vi "Omniax_MotorDrive_XYZR_20100916stable2.vi"() -> ()   [LabVIEW 2009]
uses:
  <vilib>/Utility/file.llb/Read From Spreadsheet File (DBL).vi
  <vilib>/Utility/file.llb/Read From Spreadsheet File (string).vi
  <vilib>/Instr/_visa.llb/VISA Configure Serial Port (Instr).vi
  <vilib>/Utility/file.llb/Write To Spreadsheet File (string).vi
  <vilib>/Utility/file.llb/Write To Spreadsheet File (DBL).vi
panel:
  out "Scanning":bool
  out "Laser Shutter":bool
  in  "SHUTTER SYNC":bool
  in  "Laser Shutter":bool
  out "#th loop":dbl
  in  "# of loops":dbl
  in  "LOOP":bool
  out "OP":bool
  out "CL":bool
  out "Valve \nopend/closed":bool
  in  "OK Button":bool
  out "STATUS":string
  in  "Delete Button":bool
  in  "String":string
  in  "Add Button":bool
  in  "Set Button":bool
  in  "Preset positions":i32(ring) items=["ZERO", "Default", "CDOSE", "QMS", "test", "test2", "test3", "yag position", "Sample Long Edge  ", "SPUTTER POS"]
  out "Presets":i32[][](array[numeric])
  out "X MINPOS":i32=-94296
  out "X MAXPOS":i32=-34296
  out "Y MINPOS":i32=-94296
  out "Y MAXPOS":i32=-34296
  out "R MAXPOS":i32=-34296
  out "R MINPOS":i32=-94296
  out "Z MINPOS":i32=-94296
  out "Z MAXPOS":i32=-34296
  in  "HARDSTOP":bool
  in  "GO":bool
  out "XYZR VEL PV Array":i32[](array[numeric])
  out "XYZ in RANGE Array":bool[](array[boolean])
  out "STEP SP Array":i32[](array[numeric])
  out "RUNHOLDArray":i32[](array[numeric])
  out "ZCONSTArray":dbl[](array[numeric])
  out "RCONSTArray":dbl[](array[numeric])
  out "XCONSTArray":dbl[](array[numeric])
  out "YCONSTArray":dbl[](array[numeric])
  out "Error Array":errorcluster[](array[cluster])
  out "COM PORT Array":refnum<visa-resource-name>[](array[refnum])
  out "Z COM PORT":refnum<visa-resource-name>="COM6"
  in  "Tab Control 3":enum32{"Status", "Reset"}(tab)
  out "Y in Range":bool
  out "Y Scan":bool
  out "Y in Motion":bool
  out "Y Backlash corr":bool
  out "X  in Range":bool
  out "X Scan":bool
  out "X  in Motion":bool
  out "X Backlash corr":bool
  out "Z in Range":bool
  out "Z Scan":bool
  out "Z in Motion":bool
  out "Z Backlash corr":bool
  out "R in Range":bool
  out "R Scan":bool
  out "R in Motion":bool
  out "R Backlash corr":bool
  out "X Ready":bool
  out "Y Ready":bool
  out "Z Ready":bool
  out "R Ready":bool
  in  "Reset Y Position mm":dbl
  out "Reset Y Motor Steps":i32
  in  "Reset X Position mm":dbl
  out "Reset X Motor Steps":i32
  in  "Reset Z Position mm":dbl
  out "Reset Z Motor Steps":i32
  in  "Reset R Position deg":dbl
  out "Reset R Motor Steps":i32
  in  "Reset":bool
  in  "Tab Control 2":enum32{"mm", "step"}(tab)
  in  "X Scan Length SP mm":dbl
  in  "X Scan Velocity SP mm/sec":dbl
  in  "Y Scan Length SP mm":dbl
  in  "Y Scan Velocity SP mm/sec":dbl
  in  "Set Scan \nParameters":bool
  in  "Z Scan Length SP mm":dbl
  in  "Z Scan Velocity SP mm/sec":dbl
  in  "R Scan Length SP deg":dbl
  in  "R Scan Velocity SP deg/sec":dbl
  in  "Z as dominating length":bool
  in  "X Scan Velocity SP steps/sec":i32=1 min=1 max=102400 step=1
  in  "X Scan Length SP steps":i32 min=-2304000 max=2304000 step=100
  out "X Scan length MV mm":dbl
  out "X Scan velocity MV mm/sec":dbl format="%#_6f"
  in  "Y Scan Velocity SP steps/sec":i32=1 min=1 max=102400 step=1
  in  "Y Scan Length SP steps":i32 min=-2304000 max=2304000 step=100
  out "Y Scan length MV mm":dbl
  out "Y Scan velocity MV mm/sec":dbl format="%#_6f"
  in  "Z Scan Velocity SP steps/sec":i32=1 min=1 max=204800 step=1
  in  "Z Scan Length SP steps":i32 min=-10240000 max=92160000 step=100
  out "Z Scan length MV mm":dbl
  out "Z Scan velocity MV mm/sec":dbl format="%#_6f"
  in  "R Scan Velocity SP steps/sec":i32=1 min=1 max=102400 step=1
  in  "R Scan Length SP steps":i32 min=-1501867 max=4642133 step=100
  out "R Scan length MV deg":dbl
  out "R Scan velocity MV deg/sec":dbl format="%#_6f"
  out "atan Y/Z":dbl
  in  "Tab Control":enum32{"mm", "step"}(tab)
  in  "X Position SP mm":dbl
  in  "X Velocity SP mm/sec":dbl
  in  "X Move Set":bool
  in  "Y Move Set":bool
  in  "Y Position SP mm":dbl
  in  "Y Velocity SP mm/sec":dbl
  in  "Z Position SP mm":dbl
  in  "Z Velocity SP mm/sec":dbl
  in  "Z Move Set":bool
  in  "R Position SP deg":dbl
  in  "R Velocity SP deg/sec":dbl
  in  "R Move Set":bool
  in  "X Velocity SP step/sec":i32 min=1 max=128000
  out "X Velocity MV mm/sec":dbl
  in  "Y Velocity SP step/sec":i32 min=1 max=128000
  out "Y Velocity MV mm/sec":dbl
  in  "Z Velocity SP step/sec":i32 min=1 max=204800
  out "Z Velocity MV mm/sec":dbl
  in  "R Velocity SP step/sec":i32 min=1 max=20000
  out "R Velocity MVdeg/sec":dbl
  in  "Y Step SP":i32=-20000 min=-2304000 max=2304000 step=500
  out "Y Position MV mm":dbl
  in  "X Step SP":i32=-20000 min=-2304000 max=2304000 step=500
  out "X Position MV mm":dbl
  in  "Z Step SP":i32=-20000 min=0 max=102400000 step=500
  out "Z Position MV mm":dbl
  in  "R Step SP":i32=-20000 min=-6144000 max=0 step=500
  out "R Position MV deg":dbl
  out "X Step PV":i32 max=2000
  out "Y Step PV":i32 max=2000
  out "Z Step PV":i32 max=2000
  out "R Step PV":i32 max=2000
  in  "Clear ZY":bool
  out "ZY Graph":cluster{dbl[], dbl[]}(graph)
  out "ZR Graph":cluster{"Y":dbl[], "Y":dbl[]}[](graph)
  out "XY Graph":cluster{"Y":dbl[], "Y":dbl[]}[](graph)
  out "X Scan Duration":dbl
  out "Y Scan Duration":dbl
  out "Z Scan Duration":dbl
  out "R Scan Duration":dbl
  out "R Backlash steps/sec":i32
  out "R Backlash":i32
  out "R Holding Current %":i32
  out "R Run Current %":i32
  out "R offset deg":dbl
  out "R deg/rev":dbl
  out "R steps/rev":u32
  out "R velocity PV step/sec":i32
  out "R COM PORT":refnum<visa-resource-name>="COM5"
  out "R Position deg PV":dbl
  out "Z Backlash steps/sec":i32
  out "Z Backlash":i32
  out "Z Holding Current %":i32
  out "Z Run Current %":i32
  out "Z offset mm":dbl
  out "Z mm/rev":dbl
  out "Z steps/rev":u32
  out "Z  velocity PV step/sec":i32
  out "Z Position mm PV":dbl
  out "X Position mm PV":dbl
  out "X velocity PV step/sec":i32
  in  "Send scan parameter":bool
  out "X Backlash steps/sec":i32
  out "X Backlash":i32
  out "X Holding Current %":i32
  out "X Run Current %":i32
  out "X offset mm":dbl
  out "X mm/rev":dbl
  out "X steps/rev":u32
  out "X COM PORT":refnum<visa-resource-name>="COM5"
  out "Y Backlash steps/sec":i32
  out "Y Backlash":i32
  out "Y Holding Current %":i32
  out "Y Run Current %":i32
  in  "Scan Cancel":bool
  out "Y Position mm PV":dbl
  out "Y offset mm":dbl
  out "Y mm/rev":dbl
  out "Y steps/rev":u32
  out "Y velocity PV step/sec":i32
  in  "Scan Go":bool
  in  "Stop":bool
  out "Y COM PORT":refnum<visa-resource-name>="COM5"
  # "MX"
  # "MY"
  # "MZ"
  # "MR"
  # "Indicators"
  # "L"
  # "M"
  # "B"
  # "S"
  # "R"
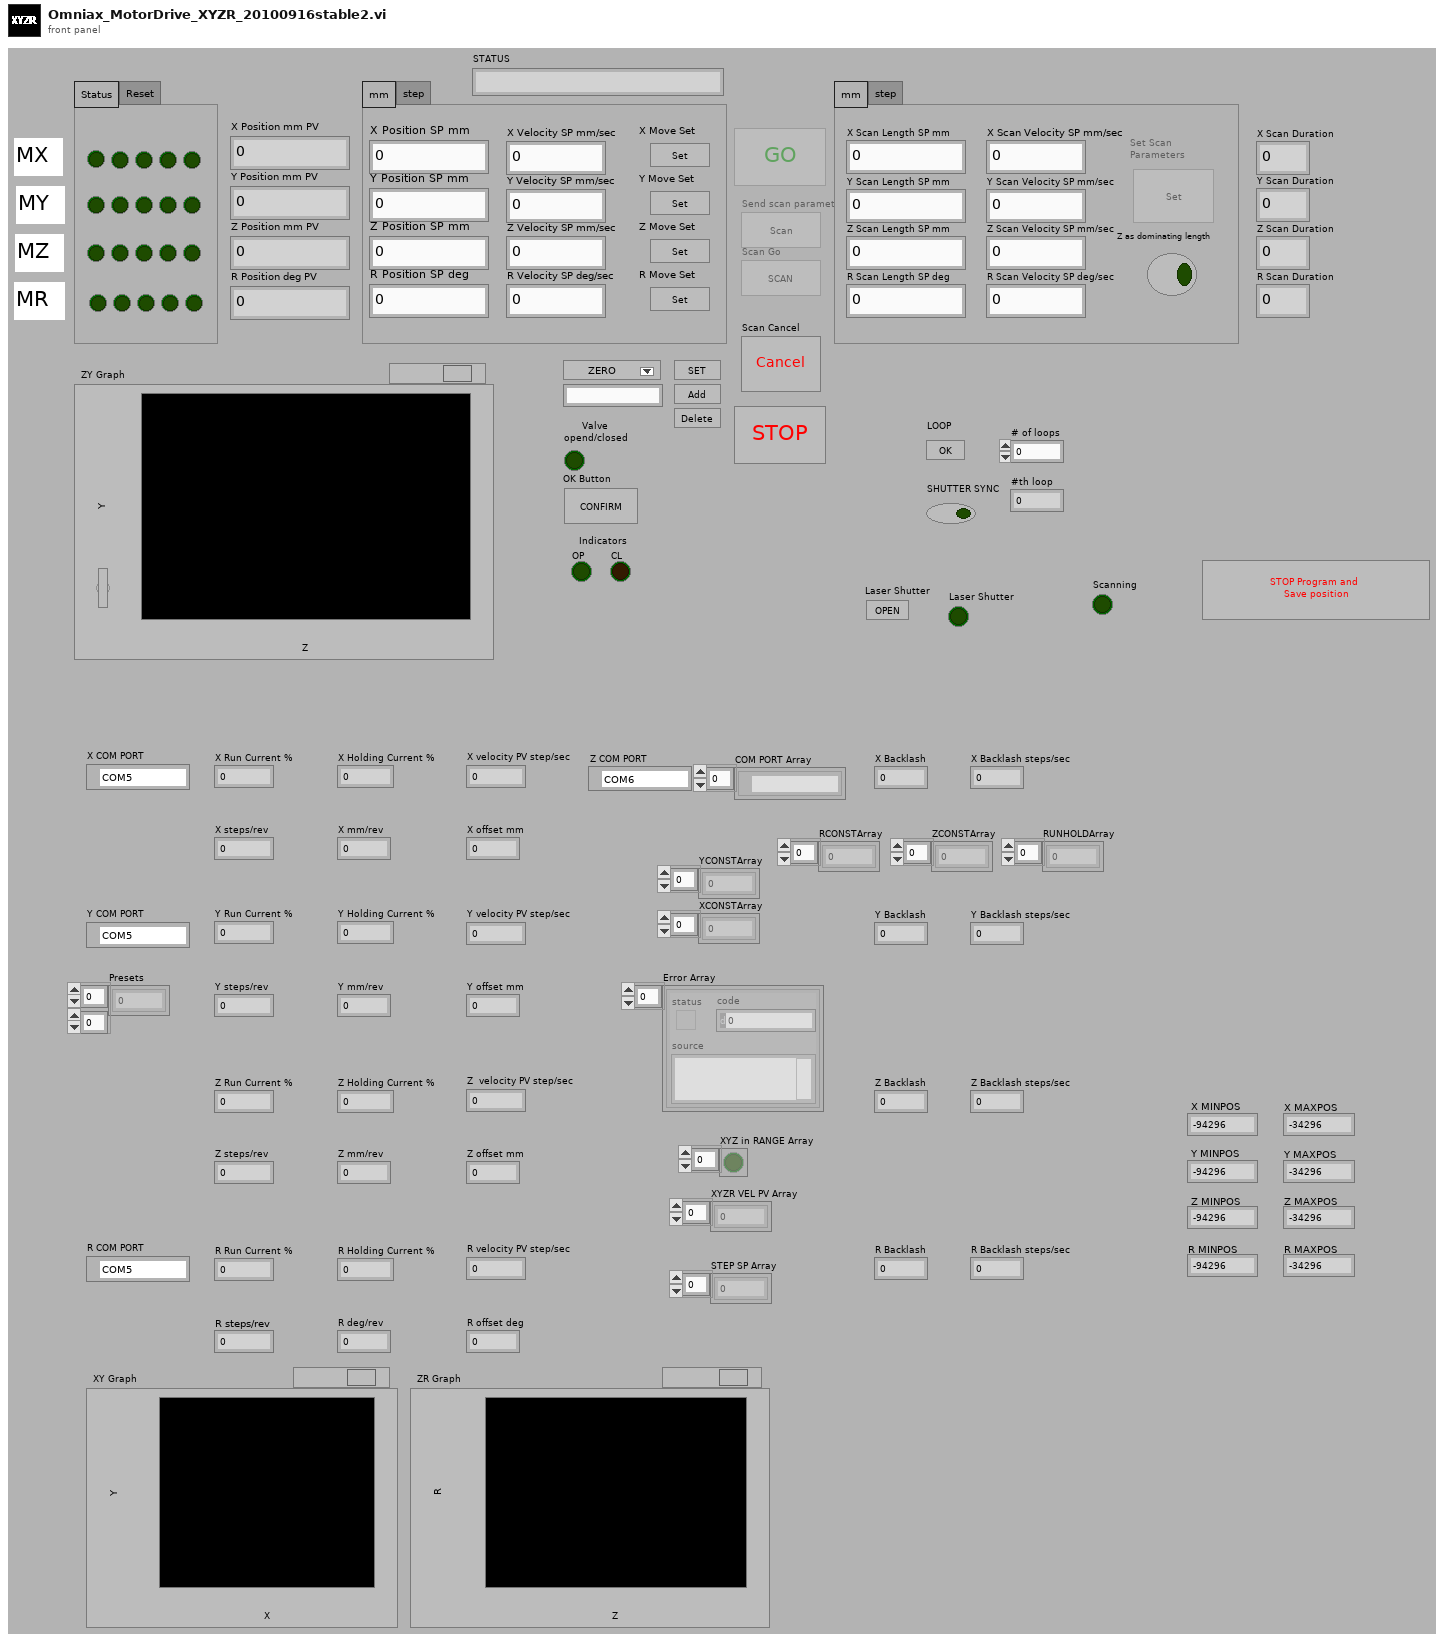
[diagram p1: front panel]
types:
  T1 = cluster{"Error Array OUT[0]":errorcluster, "Error Array OUT[1]":errorcluster, "Error Array OUT[2]":errorcluster, "Error Array OUT[3]":errorcluster, "Error Array OUT[4]":errorcluster, "Error Array OUT[5]":errorcluster, "Error Array OUT[6]":errorcluster, "Error Array OUT[7]":errorcluster, "Error Array OUT[8]":errorcluster}
  T2 = cluster{"COM PORT Array OUT[0]":refnum<visa-resource-name>, "COM PORT Array OUT[1]":refnum<visa-resource-name>, "COM PORT Array OUT[2]":refnum<visa-resource-name>, "COM PORT Array OUT[3]":refnum<visa-resource-name>, "COM PORT Array OUT[4]":refnum<visa-resource-name>, "COM PORT Array OUT[5]":refnum<visa-resource-name>, "COM PORT Array OUT[6]":refnum<visa-resource-name>, "COM PORT Array OUT[7]":refnum<visa-resource-name>, "COM PORT Array OUT[8]":refnum<visa-resource-name>}
  T3 = cluster{"STEP SP Array OUT[0]":i32, "STEP SP Array OUT[1]":i32, "STEP SP Array OUT[2]":i32, "STEP SP Array OUT[3]":i32, "STEP SP Array OUT[4]":i32, "STEP SP Array OUT[5]":i32, "STEP SP Array OUT[6]":i32, "STEP SP Array OUT[7]":i32, "STEP SP Array OUT[8]":i32}
  T4 = cluster{"XYZR MAX MIN POS[0]":i32, "XYZR MAX MIN POS[1]":i32, "XYZR MAX MIN POS[2]":i32, "XYZR MAX MIN POS[3]":i32, "XYZR MAX MIN POS[4]":i32, "XYZR MAX MIN POS[5]":i32, "XYZR MAX MIN POS[6]":i32, "XYZR MAX MIN POS[7]":i32, "XYZR MAX MIN POS[8]":i32}
  T5 = cluster{"XYZ in RANGE Array OUT[0]":bool, "XYZ in RANGE Array OUT[1]":bool, "XYZ in RANGE Array OUT[2]":bool, "XYZ in RANGE Array OUT[3]":bool, "XYZ in RANGE Array OUT[4]":bool, "XYZ in RANGE Array OUT[5]":bool, "XYZ in RANGE Array OUT[6]":bool, "XYZ in RANGE Array OUT[7]":bool, "XYZ in RANGE Array OUT[8]":bool}
  T6 = cluster{"XY Max Min array OUT[0]":dbl, "XY Max Min array OUT[1]":dbl, "XY Max Min array OUT[2]":dbl, "XY Max Min array OUT[3]":dbl, "XY Max Min array OUT[4]":dbl, "XY Max Min array OUT[5]":dbl, "XY Max Min array OUT[6]":dbl, "XY Max Min array OUT[7]":dbl, "XY Max Min array OUT[8]":dbl}
  T7 = cluster{"XYZR VEL PV Array OUT[0]":i32, "XYZR VEL PV Array OUT[1]":i32, "XYZR VEL PV Array OUT[2]":i32, "XYZR VEL PV Array OUT[3]":i32, "XYZR VEL PV Array OUT[4]":i32, "XYZR VEL PV Array OUT[5]":i32, "XYZR VEL PV Array OUT[6]":i32, "XYZR VEL PV Array OUT[7]":i32, "XYZR VEL PV Array OUT[8]":i32}
  T8 = cluster{"[0]":i32, "[1]":i32, "[2]":i32, "[3]":i32, "[4]":i32, "[5]":i32, "[6]":i32, "[7]":i32, "[8]":i32}
  T9 = enum8{"Enabled", "Disabled", "Disabled and Grayed Out"}
  T10 = enum16{"Stop", "Reset", "Run Current", "Holding Current", "Accel Rate", "Decel Rate", "Move to Relative Position", "Move to Absolute Position", "Echo Mode", "Print Parameter", "Send String", "Microstep Resolution", "Set Current Position", "Max Velocity"}
  T11 = cluster{"Presets[0]":i32, "Presets[1]":i32, "Presets[2]":i32, "Presets[3]":i32, "Presets[4]":i32, "Presets[5]":i32, "Presets[6]":i32, "Presets[7]":i32, "Presets[8]":i32}
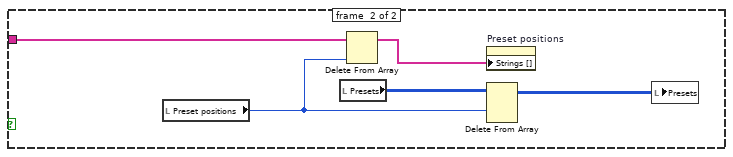
[diagram p4: hidden frame]
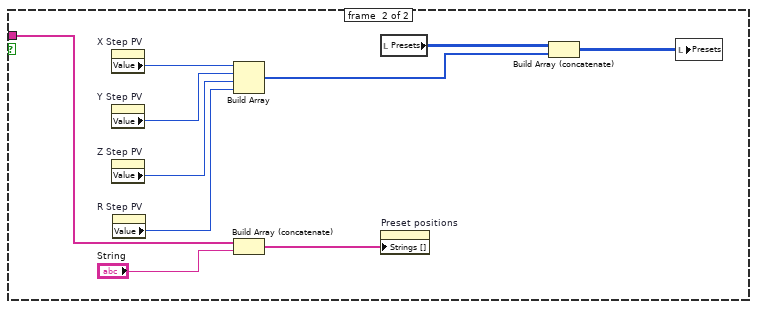
[diagram p5: hidden frame]
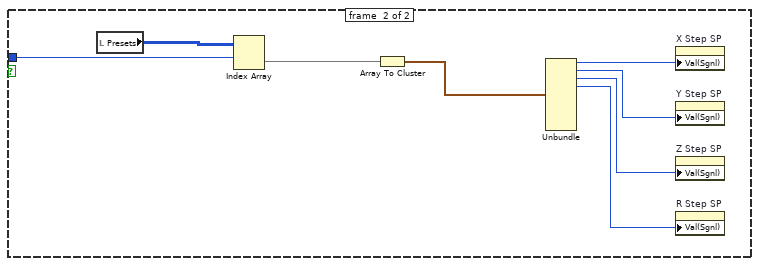
[diagram p6: hidden frame]
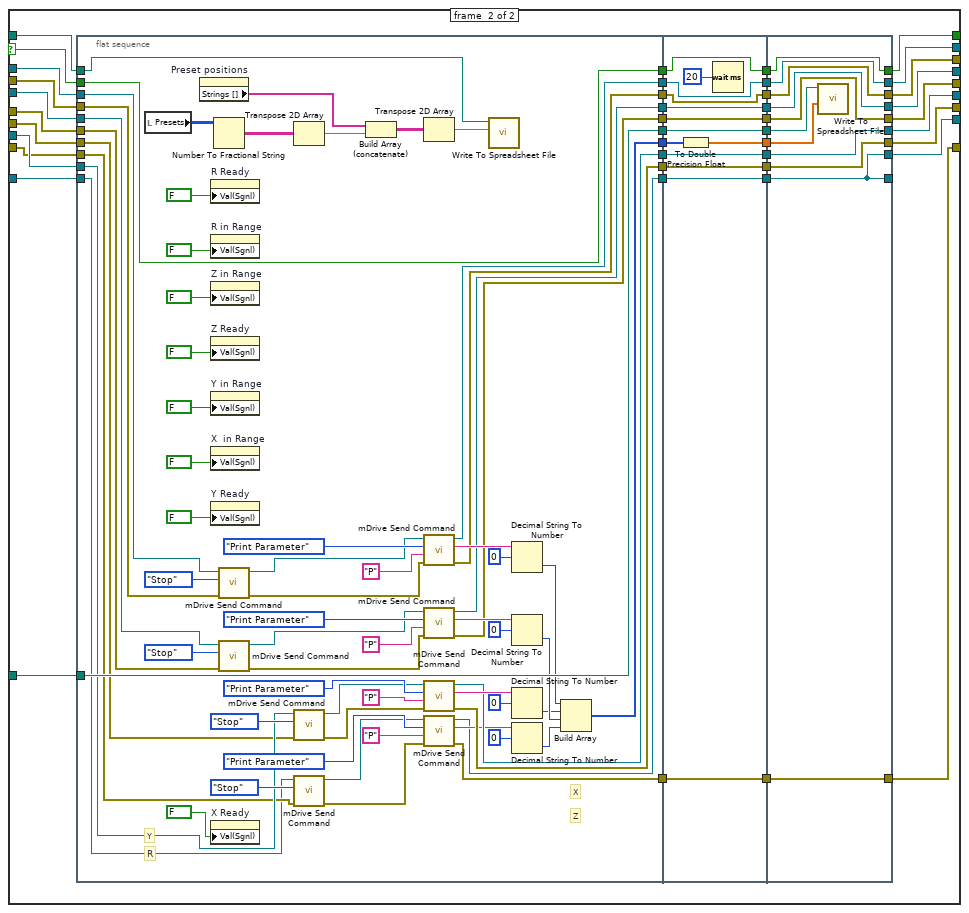
[diagram p7: hidden frame]
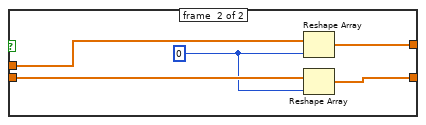
[diagram p8: hidden frame]
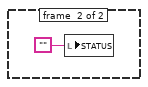
[diagram p10: hidden frame]
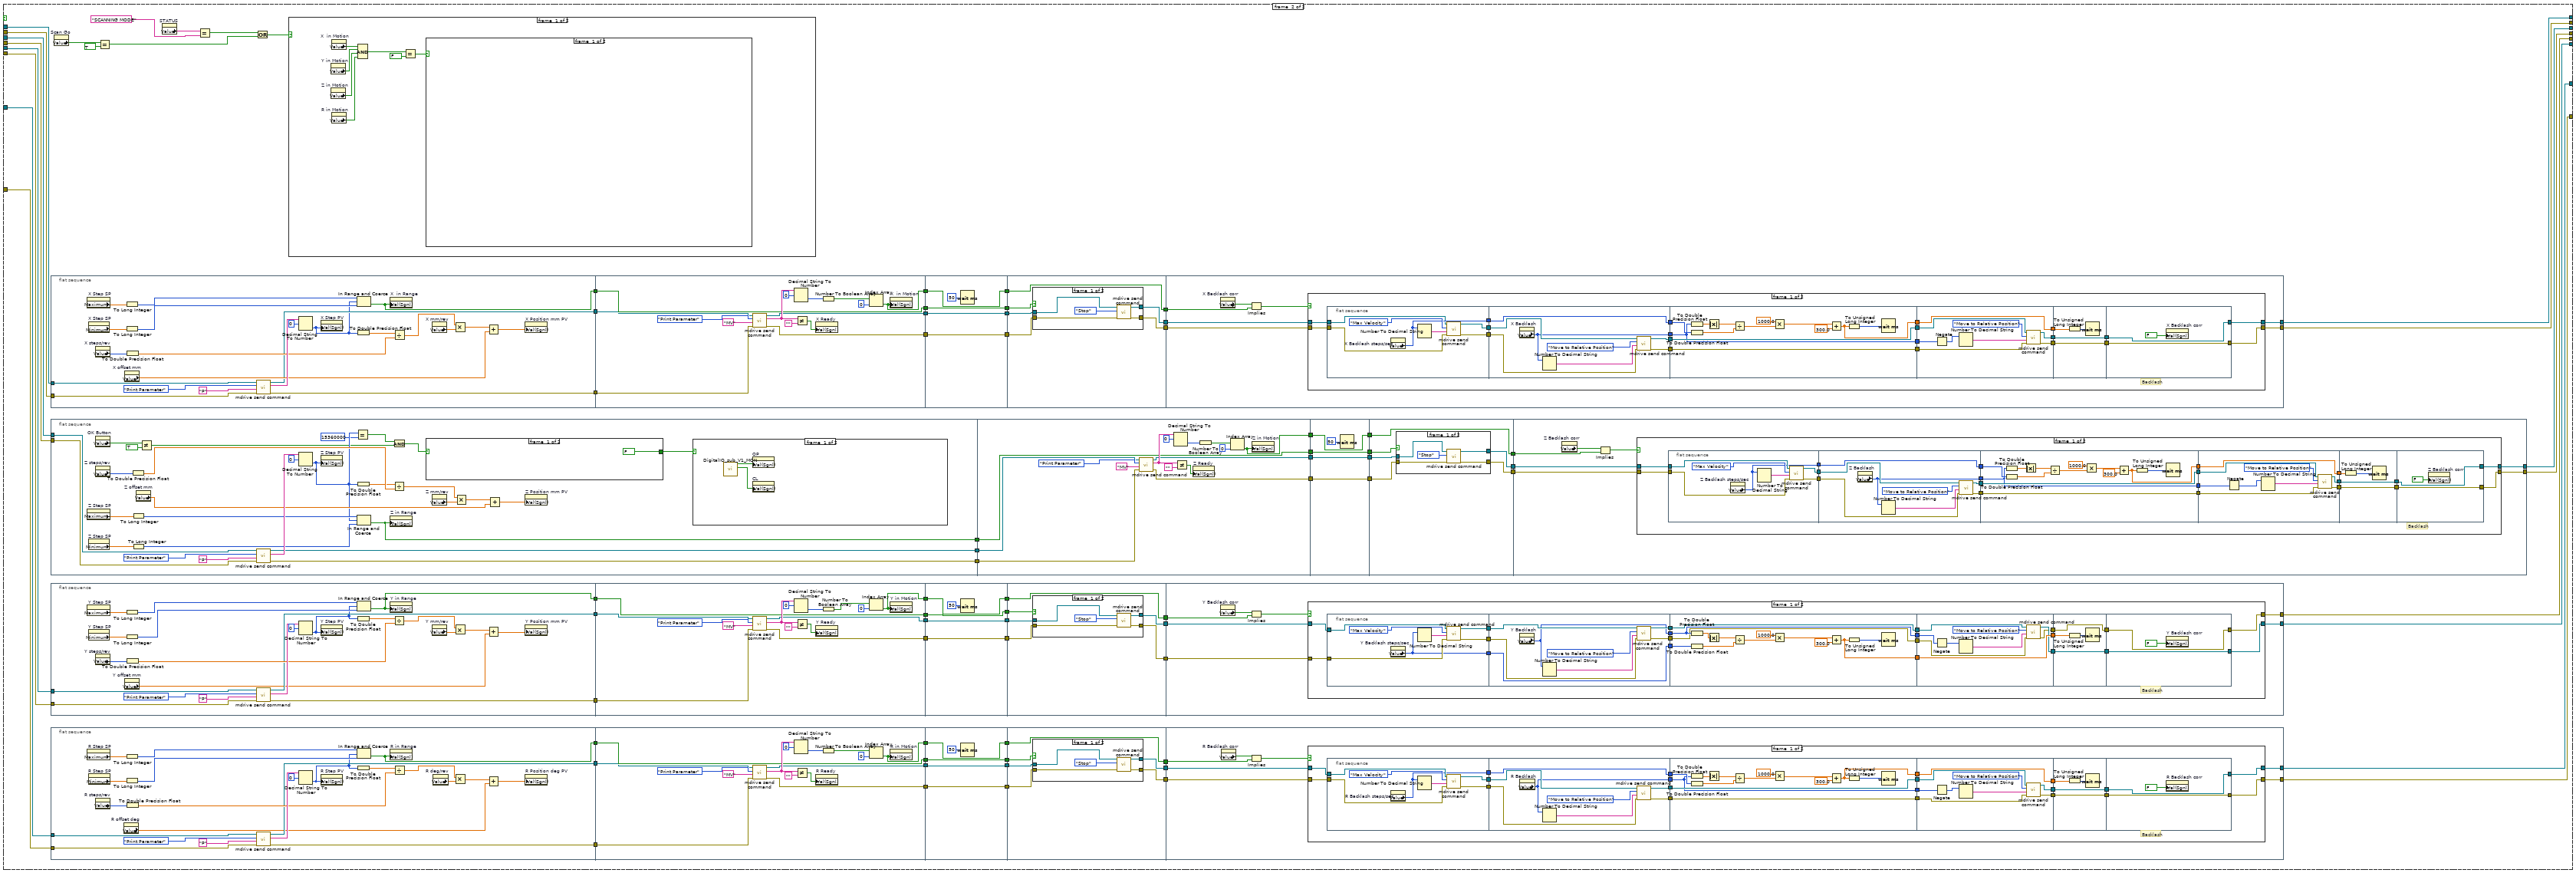
[diagram p11: hidden frame]
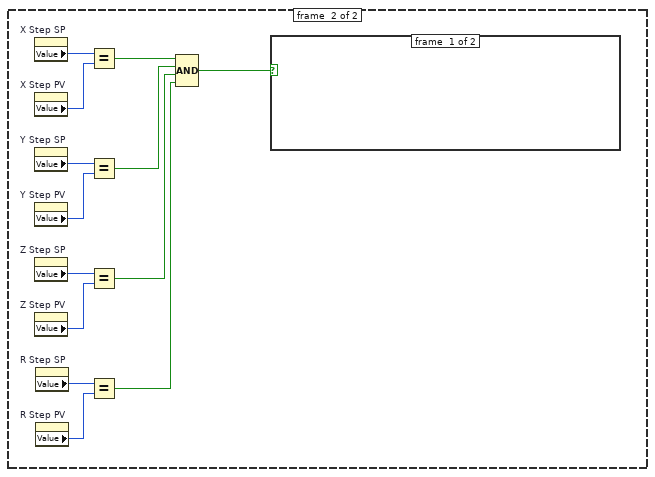
[diagram p12: hidden frame]
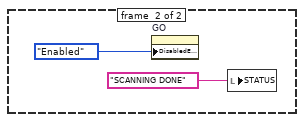
[diagram p13: hidden frame]
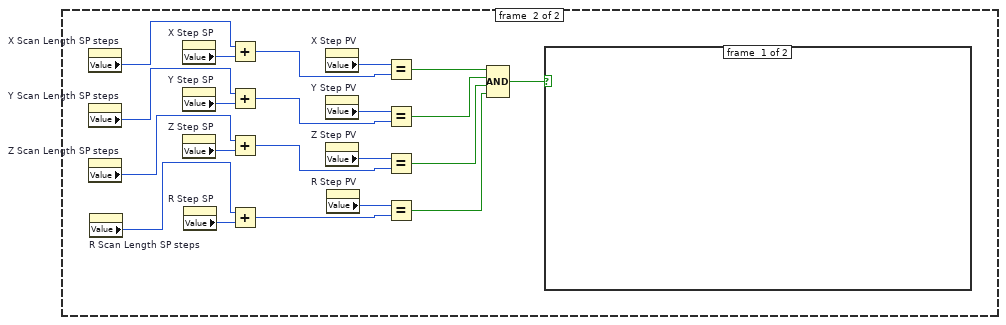
[diagram p14: hidden frame]
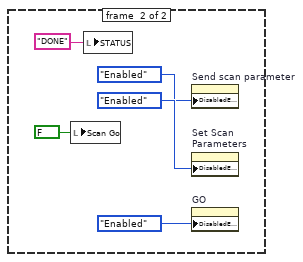
[diagram p15: hidden frame]
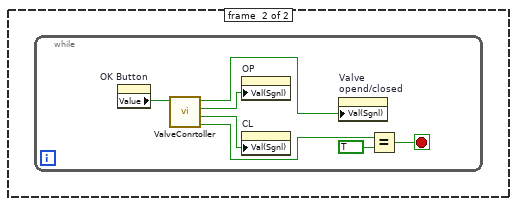
[diagram p20: hidden frame]
diagram:
  (unwired) FALSE ("LOOP MODE")
  n1 = flat-sequence {
    tunnel: [w153] -> w10
    tunnel: [w152] -> w9
    tunnel: [w151] -> w8
    tunnel: [w150] -> w7
    tunnel: [w149] -> w6
    tunnel: [w148] -> w5
    tunnel: [w147] -> w4
    tunnel: [w146] -> w3
    tunnel: [w143] -> w2
    tunnel: [w113] -> w1
    tunnel: [w188] -> w13
    tunnel: [w189] -> w14
    tunnel: [w190] -> w15
    tunnel: [w191] -> w16
    tunnel: [w192] -> w17
    tunnel: [w193] -> w18
    tunnel: [w194] -> w19
    tunnel: [w195] -> w20
    tunnel: [w196] -> w21
    tunnel: [w197] -> w22
    tunnel: w10 -> [w197]
    tunnel: w9 -> [w196]
    tunnel: w8 -> [w195]
    tunnel: w7 -> [w194]
    tunnel: w6 -> [w193]
    tunnel: w5 -> [w192]
    tunnel: w4 -> [w191]
    tunnel: w3 -> [w190]
    tunnel: w2 -> [w189]
    tunnel: w1 -> [w188]
    frame #0 {
      w113 = path "C:/Documents and Settings/b_ogasawara/Desktop/lv1/LV codes/IMS/PRESET.TXT"
      w111 = 0 ("element")
      w143 = path "C:/Documents and Settings/b_ogasawara/Desktop/lv1/LV codes/IMS/POS.TXT"
      w173 = refnum<visa-resource-name> "COM7" ("COM PORT")
      w174 = refnum<visa-resource-name> "COM5" ("COM PORT")
      w175 = refnum<visa-resource-name> "COM6" ("VISA resource name")
      w176 = refnum<visa-resource-name> "COM4" ("COM PORT")
      n2 = property on="Z Step SP" class="DigNum (strict)"() -> ("Maximum"=w68:dbl)  [unwired: 2 in, 2 out]
      n3 = property on="R Step SP" class="DigNum (strict)"() -> ("Maximum"=w66:dbl)  [unwired: 2 in, 2 out]
      n4 = property on="Z Step SP" class="DigNum (strict)"() -> ("Minimum"=w69:dbl)  [unwired: 2 in, 2 out]
      n5 = property on="R Step SP" class="DigNum (strict)"() -> ("Minimum"=w67:dbl)  [unwired: 2 in, 2 out]
      n6 = property on="X steps/rev" class="DigNum (strict)"() -> ("Value"=w84:u32)  [unwired: 2 in, 2 out]
      n7 = property on="Y steps/rev" class="DigNum (strict)"() -> ("Value"=w83:u32)  [unwired: 2 in, 2 out]
      n8 = property on="Z steps/rev" class="DigNum (strict)"() -> ("Value"=w82:u32)  [unwired: 2 in, 2 out]
      n9 = property on="R steps/rev" class="DigNum (strict)"() -> ("Value"=w81:u32)  [unwired: 2 in, 2 out]
      n10 = call "DigitalIO_sub_V1_MON.vi"() -> ("CL"=w70:bool, "OP"=w71:bool)  [unwired: 8 in]
      n11 = local read "RUNHOLDArray"() -> (w163:i32[])
      n12 = local read "STEP SP Array"() -> (w166:i32[])
      n13 = local read "XYZ in RANGE Array"() -> (w165:bool[])
      n14 = local read "XYZR VEL PV Array"() -> (w164:i32[])
      n15 = property on="R offset deg" class="DigNum (strict)"() -> ("Value"=w76:dbl)  [unwired: 2 in, 2 out]
      n16 = property on="X offset mm" class="DigNum (strict)"() -> ("Value"=w73:dbl)  [unwired: 2 in, 2 out]
      n17 = property on="Y offset mm" class="DigNum (strict)"() -> ("Value"=w74:dbl)  [unwired: 2 in, 2 out]
      n18 = property on="Z offset mm" class="DigNum (strict)"() -> ("Value"=w75:dbl)  [unwired: 2 in, 2 out]
      n19 = property on="OP" class="Bool (strict)"("Val(Sgnl)"=w71) -> ()  [unwired: 2 in, 2 out]
      n20 = property on="CL" class="Bool (strict)"("Val(Sgnl)"=w70) -> ()  [unwired: 2 in, 2 out]
      n21 = Build Array(w176, w175, w174, w173) -> (w171:refnum<visa-resource-name>[])
      n22 = Build Array(w68, w69, w66, w67) -> (w65:dbl[])
      n23 = local write "STATUS"("INITIALIZING" ("STATUS")) -> ()
      n24 = for {
        N: 4 -> [_]
        tunnel: w171 -> [w179] mode=indexing
        tunnel: [w178] -> w169 mode=indexing
        tunnel: [w177] -> w170 mode=indexing
        w181 = u16 0 items=["None", "XON/XOFF", "RTS/CTS", "XON/XOFF & RTS/CTS", "DTR/DSR", "XON/XOFF & DTR/DSR"] ("flow control (0:none)")
        w182 = u16 10 items=["1.0"=10, "1.5"=15, "2.0"=20] ("stop bits (10: 1 bit)")
        # "Stop bits"
        n25 = call-poly "VISA Configure Serial Port"("VISA resource name"=w179, "timeout (10sec)"=u32 10000, "baud rate (9600)"=u32 9600, "data bits (8)"=u16 8, "parity (0:none)"=enum16{"None", "Odd", "Even", "Mark", "Space"}."None", "stop bits (10: 1 bit)"=w182, "flow control (0:none)"=w181) -> ("VISA resource name out"=w178:refnum<visa-resource-name>, "error out"=w177:errorcluster)  [unwired: 7 in]
      }
      "COM PORT Array" <- w169
      "Error Array" <- w170
      n26 = call "InitializeMotorsXYZR_V2.vi"("COM PORT Array IN"=w169, "STEP SP Array IN"=w166, "XYZ in RANGE Array IN"=w165, "XYZR VEL PV Array IN"=w164, "RUNHOLDArray IN"=w163, "Error Array IN"=w170, "ZR Max Min array"=w65) -> ("XY Max Min array OUT"=w64:dbl[], "COM PORT Array OUT"=w168:refnum<visa-resource-name>[], "STEP SP Array OUT"=w162:i32[], "XYZ in RANGE Array OUT"=w161:bool[], "XYZR VEL PV Array OUT"=w160:i32[], "XYZR MAX MIN POS"=w145:i32[], "Error Array OUT"=w167:errorcluster[])  [unwired: 6 in]
      n27 = Array To Cluster(array=w167) -> (cluster=w158:T1)
      n28 = Array To Cluster(array=w168) -> (cluster=w159:T2)
      n29 = Array To Cluster(array=w162) -> (cluster=w157:T3)
      n30 = Array To Cluster(array=w145) -> (cluster=w154:T4)
      n31 = Array To Cluster(array=w161) -> (cluster=w156:T5)
      n32 = Array To Cluster(array=w64) -> (cluster=w63:T6)
      n33 = Array To Cluster(array=w160) -> (cluster=w155:T7)
      n34 = Unbundle(w157) -> ("STEP SP Array OUT[0]"=w127:i32, "STEP SP Array OUT[1]"=w128:i32, "STEP SP Array OUT[2]"=w129:i32, "STEP SP Array OUT[3]"=w130:i32)  [unwired: 5 out]
      n35 = Unbundle(w154) -> ("XYZR MAX MIN POS[0]"=w138:i32, "XYZR MAX MIN POS[1]"=w137:i32, "XYZR MAX MIN POS[2]"=w136:i32, "XYZR MAX MIN POS[3]"=w135:i32, "XYZR MAX MIN POS[4]"=w134:i32, "XYZR MAX MIN POS[5]"=w133:i32, "XYZR MAX MIN POS[6]"=w132:i32, "XYZR MAX MIN POS[7]"=w131:i32)  [unwired: 1 out]
      n36 = Unbundle(w156) -> ("XYZ in RANGE Array OUT[0]"=w142:bool, "XYZ in RANGE Array OUT[1]"=w141:bool, "XYZ in RANGE Array OUT[2]"=w140:bool, "XYZ in RANGE Array OUT[3]"=w139:bool)  [unwired: 5 out]
      n37 = Unbundle(w63) -> ("XY Max Min array OUT[0]"=w62:dbl, "XY Max Min array OUT[1]"=w60:dbl, "XY Max Min array OUT[2]"=w59:dbl, "XY Max Min array OUT[3]"=w61:dbl)  [unwired: 5 out]
      n38 = Unbundle(w155) -> ("XYZR VEL PV Array OUT[0]"=w126:i32, "XYZR VEL PV Array OUT[1]"=w125:i32, "XYZR VEL PV Array OUT[2]"=w124:i32, "XYZR VEL PV Array OUT[3]"=w123:i32)  [unwired: 5 out]
      n39 = call-poly <vilib>:"Read From Spreadsheet File.vi"("file path (dialog if empty)"=w113) -> ("all rows"=w118:string[][])  [unwired: 6 in, 4 out]
      n40 = call-poly <vilib>:"Read From Spreadsheet File.vi"("file path (dialog if empty)"=w143) -> ("first row"=w144:dbl[])  [unwired: 6 in, 4 out]
      n41 = To Long Integer(number=w144) -> (32bit integer=w110:i32[])
      n42 = Transpose 2D Array(2D array=w118) -> (transposed array=w117:string[][])
      n43 = property on="X Step SP" class="DigNum (strict)"("Val(Sgnl)"=w127) -> ()  [unwired: 2 in, 2 out]
      n44 = property on="Y Step SP" class="DigNum (strict)"("Val(Sgnl)"=w128) -> ()  [unwired: 2 in, 2 out]
      n45 = property on="Z Step SP" class="DigNum (strict)"("Val(Sgnl)"=w129) -> ()  [unwired: 2 in, 2 out]
      n46 = property on="R Step SP" class="DigNum (strict)"("Val(Sgnl)"=w130) -> ()  [unwired: 2 in, 2 out]
      n47 = property on="X MAXPOS" class="DigNum (strict)"("Val(Sgnl)"=w138) -> ()  [unwired: 2 in, 2 out]
      n48 = property on="X MINPOS" class="DigNum (strict)"("Val(Sgnl)"=w137) -> ()  [unwired: 2 in, 2 out]
      n49 = property on="Y MAXPOS" class="DigNum (strict)"("Val(Sgnl)"=w136) -> ()  [unwired: 2 in, 2 out]
      n50 = property on="Y MINPOS" class="DigNum (strict)"("Val(Sgnl)"=w135) -> ()  [unwired: 2 in, 2 out]
      n51 = property on="Z MAXPOS" class="DigNum (strict)"("Val(Sgnl)"=w134) -> ()  [unwired: 2 in, 2 out]
      n52 = property on="Z MINPOS" class="DigNum (strict)"("Val(Sgnl)"=w133) -> ()  [unwired: 2 in, 2 out]
      n53 = property on="R MAXPOS" class="DigNum (strict)"("Val(Sgnl)"=w132) -> ()  [unwired: 2 in, 2 out]
      n54 = property on="R MINPOS" class="DigNum (strict)"("Val(Sgnl)"=w131) -> ()  [unwired: 2 in, 2 out]
      n55 = property on="X  in Range" class="Bool (strict)"("Val(Sgnl)"=w142) -> ()  [unwired: 2 in, 2 out]
      n56 = property on="Y in Range" class="Bool (strict)"("Val(Sgnl)"=w141) -> ()  [unwired: 2 in, 2 out]
      n57 = property on="Z in Range" class="Bool (strict)"("Val(Sgnl)"=w140) -> ()  [unwired: 2 in, 2 out]
      n58 = property on="R in Range" class="Bool (strict)"("Val(Sgnl)"=w139) -> ()  [unwired: 2 in, 2 out]
      n59 = property on="X velocity PV step/sec" class="DigNum (strict)"("Val(Sgnl)"=w126) -> ()  [unwired: 2 in, 2 out]
      n60 = property on="R velocity PV step/sec" class="DigNum (strict)"("Val(Sgnl)"=w123) -> ()  [unwired: 2 in, 2 out]
      n61 = property on="X Step SP" class="DigNum (strict)"("Maximum"=w62) -> ()  [unwired: 2 in, 2 out]
      n62 = property on="X Step SP" class="DigNum (strict)"("Minimum"=w60) -> ()  [unwired: 2 in, 2 out]
      n63 = property on="Y Step SP" class="DigNum (strict)"("Maximum"=w59) -> ()  [unwired: 2 in, 2 out]
      n64 = property on="Y Step SP" class="DigNum (strict)"("Minimum"=w61) -> ()  [unwired: 2 in, 2 out]
      n65 = property on="Y velocity PV step/sec" class="DigNum (strict)"("Val(Sgnl)"=w125) -> ()  [unwired: 2 in, 2 out]
      n66 = property on="Z  velocity PV step/sec" class="DigNum (strict)"("Val(Sgnl)"=w124) -> ()  [unwired: 2 in, 2 out]
      n67 = Array To Cluster(array=w110) -> (cluster=w109:T8)
      n68 = Delete From Array(array=w117, index (row)=0) -> (deleted portion=w112:string[], array with subset deleted=w115:string[][])  [unwired: 2 in]
      n69 = Transpose 2D Array(2D array=w115) -> (transposed array=w114:string[][])
      n70 = property on="Preset positions" class="Ring (strict)"("Strings []"=w112) -> ()  [unwired: 2 in, 2 out]
      n71 = Unbundle(w109) -> ("[0]"=w85:i32, "[1]"=w86:i32, "[2]"=w87:i32, "[3]"=w88:i32)  [unwired: 5 out]
      n72 = To Double Precision Float(number=w84) -> (double precision float=w105:dbl)
      n73 = To Double Precision Float(number=w85) -> (double precision float=w106:dbl)
      n74 = To Double Precision Float(number=w83) -> (double precision float=w101:dbl)
      n75 = To Double Precision Float(number=w86) -> (double precision float=w102:dbl)
      n76 = To Double Precision Float(number=w87) -> (double precision float=w98:dbl)
      n77 = To Double Precision Float(number=w82) -> (double precision float=w97:dbl)
      n78 = To Double Precision Float(number=w88) -> (double precision float=w94:dbl)
      n79 = To Double Precision Float(number=w81) -> (double precision float=w93:dbl)
      n80 = property on="Reset X Motor Steps" class="DigNum (strict)"("Val(Sgnl)"=w85) -> ()  [unwired: 2 in, 2 out]
      n81 = property on="Reset Y Motor Steps" class="DigNum (strict)"("Val(Sgnl)"=w86) -> ()  [unwired: 2 in, 2 out]
      n82 = property on="Reset Z Motor Steps" class="DigNum (strict)"("Val(Sgnl)"=w87) -> ()  [unwired: 2 in, 2 out]
      n83 = property on="Reset R Motor Steps" class="DigNum (strict)"("Val(Sgnl)"=w88) -> ()  [unwired: 2 in, 2 out]
      n84 = Decimal String To Number(string=w114) -> (number=w116:i32[][])  [unwired: 2 in, 1 out]
      n85 = Divide(x=w106, y=w105) -> (x/y=w108:dbl)
      n86 = Divide(x=w102, y=w101) -> (x/y=w104:dbl)
      n87 = Divide(x=w98, y=w97) -> (x/y=w100:dbl)
      n88 = Divide(x=w94, y=w93) -> (x/y=w96:dbl)
      n89 = Initialize Array(w111, w111, 4 ("dimension size")) -> (w121:i32[][])
      n90 = Build Array (concatenate)(w121, w116) -> (→"Presets":i32[][])
      n91 = property on="X mm/rev" class="DigNum (strict)"() -> ("Value"=w78:dbl)  [unwired: 2 in, 2 out]
      n92 = property on="Y mm/rev" class="DigNum (strict)"() -> ("Value"=w79:dbl)  [unwired: 2 in, 2 out]
      n93 = property on="Z mm/rev" class="DigNum (strict)"() -> ("Value"=w80:dbl)  [unwired: 2 in, 2 out]
      n94 = property on="R deg/rev" class="DigNum (strict)"() -> ("Value"=w77:dbl)  [unwired: 2 in, 2 out]
      n95 = Multiply(x=w108, y=w78) -> (x*y=w107:dbl)
      n96 = Multiply(x=w104, y=w79) -> (x*y=w103:dbl)
      n97 = Multiply(x=w100, y=w80) -> (x*y=w99:dbl)
      n98 = Multiply(x=w96, y=w77) -> (x*y=w95:dbl)
      n99 = Add(x=w107, y=w73) -> (x+y=w89:dbl)
      n100 = Add(x=w103, y=w74) -> (x+y=w90:dbl)
      n101 = Add(x=w99, y=w75) -> (x+y=w91:dbl)
      n102 = Add(x=w95, y=w76) -> (x+y=w92:dbl)
      n103 = property on="X Position mm PV" class="DigNum (strict)"("Val(Sgnl)"=w89) -> ()  [unwired: 2 in, 2 out]
      n104 = property on="X Position SP mm" class="DigNum (strict)"("Val(Sgnl)"=w89) -> ()  [unwired: 2 in, 2 out]
      n105 = property on="Y Position SP mm" class="DigNum (strict)"("Val(Sgnl)"=w90) -> ()  [unwired: 2 in, 2 out]
      n106 = property on="Y Position mm PV" class="DigNum (strict)"("Val(Sgnl)"=w90) -> ()  [unwired: 2 in, 2 out]
      n107 = property on="Z Position SP mm" class="DigNum (strict)"("Val(Sgnl)"=w91) -> ()  [unwired: 2 in, 2 out]
      n108 = property on="Z Position mm PV" class="DigNum (strict)"("Val(Sgnl)"=w91) -> ()  [unwired: 2 in, 2 out]
      n109 = property on="R Position deg PV" class="DigNum (strict)"("Val(Sgnl)"=w92) -> ()  [unwired: 2 in, 2 out]
      n110 = property on="R Position SP deg" class="DigNum (strict)"("Val(Sgnl)"=w92) -> ()  [unwired: 2 in, 2 out]
      n111 = Unbundle(w159) -> ("COM PORT Array OUT[0]"=w153:refnum<visa-resource-name>, "COM PORT Array OUT[1]"=w152:refnum<visa-resource-name>, "COM PORT Array OUT[2]"=w151:refnum<visa-resource-name>, "COM PORT Array OUT[3]"=w150:refnum<visa-resource-name>)  [unwired: 5 out]
      n112 = Unbundle(w158) -> ("Error Array OUT[0]"=w149:errorcluster, "Error Array OUT[1]"=w148:errorcluster, "Error Array OUT[2]"=w147:errorcluster, "Error Array OUT[3]"=w146:errorcluster)  [unwired: 5 out]
      "X COM PORT" <- w176
      "Z COM PORT" <- w175
      "Y COM PORT" <- w174
      "R COM PORT" <- w173
    }
    frame #1 {
      w186 = T9."Disabled and Grayed Out" ("Disabled")
      w187 = T9."Enabled" ("Disabled")
      n113 = property on="LOOP" class="Bool (strict)"("DisabledEnum"=w186) -> ()  [unwired: 2 in, 2 out]
      n114 = property on="GO" class="Bool"("DisabledEnum"=w187) -> ()  [unwired: 2 in, 2 out]
      n115 = property on="Set Scan \nParameters" class="Bool"("DisabledEnum"=w187) -> ()  [unwired: 2 in, 2 out]
      n116 = property on="Send scan parameter" class="Bool"("DisabledEnum"=w186) -> ()  [unwired: 2 in, 2 out]
    }
  }
  n117 = flat-sequence {
    frame #0 {
      n118 = property on="Y Scan" class="Bool (strict)"("Val(Sgnl)"=FALSE ("Value (Signaling)")) -> ()  [unwired: 2 in, 2 out]
      n119 = property on="Z Scan Velocity SP mm/sec" class="DigNum (strict)"("Val(Sgnl)"=0.1 ("Value (Signaling)")) -> ()  [unwired: 2 in, 2 out]
      n120 = property on="Z Scan Velocity SP steps/sec" class="DigNum (strict)"("Minimum"=1.0 ("Data Entry Limits:Maximum")) -> ()  [unwired: 2 in, 2 out]
      n121 = property on="R Scan" class="Bool (strict)"("Val(Sgnl)"=FALSE ("Value (Signaling)")) -> ()  [unwired: 2 in, 2 out]
      n122 = property on="X Scan Velocity SP mm/sec" class="DigNum (strict)"("Val(Sgnl)"=0.1 ("Value (Signaling)")) -> ()  [unwired: 2 in, 2 out]
      n123 = property on="R Velocity SP deg/sec" class="DigNum (strict)"("Val(Sgnl)"=0.1 ("Value (Signaling)")) -> ()  [unwired: 2 in, 2 out]
      n124 = property on="Z Scan Velocity SP steps/sec" class="DigNum (strict)"("Maximum"=204800.0 ("Data Entry Limits:Maximum")) -> ()  [unwired: 2 in, 2 out]
      n125 = property on="X Scan" class="Bool (strict)"("Val(Sgnl)"=FALSE ("Value (Signaling)")) -> ()  [unwired: 2 in, 2 out]
      n126 = property on="Y Scan Velocity SP mm/sec" class="DigNum (strict)"("Val(Sgnl)"=0.1 ("Value (Signaling)")) -> ()  [unwired: 2 in, 2 out]
      n127 = property on="Z Scan" class="Bool (strict)"("Val(Sgnl)"=FALSE ("Value (Signaling)")) -> ()  [unwired: 2 in, 2 out]
      n128 = property on="Scan Go" class="Bool (strict)"("DisabledEnum"=T9."Disabled and Grayed Out" ("Disabled")) -> ()  [unwired: 2 in, 2 out]
    }
  }
  n129 = local read "X  in Range"() -> (w33:bool)
  n130 = flat-sequence {
    tunnel: [w212] -> w45
    frame #0 {
      w210 = 0.2 ("MM/rev")
      w215 = u32 51200 ("step/rev")
      w217 = 128000 ("Value (Signaling)")
      w218 = 1.0 ("Data Entry Limits:Minimum")
      w211 = 0.0 ("offset")
      # "a=1000000"
      n131 = property on="X Velocity SP step/sec" class="DigNum (strict)"("Val(Sgnl)"=w217) -> ()  [unwired: 2 in, 2 out]
      n132 = To Double Precision Float(number=w215) -> (double precision float=w220:dbl)
      n133 = To Double Precision Float(number=w217) -> (double precision float=w209:dbl)
      n134 = Divide(x=w209, y=w220) -> (x/y=w219:dbl)
      n135 = property on="X Velocity SP step/sec" class="DigNum (strict)"("Maximum"=w209) -> ()  [unwired: 2 in, 2 out]
      n136 = Multiply(x=w219, y=w210) -> (x*y=w213:dbl)
      n137 = To Double Precision Float(number=w217) -> (double precision float=w216:dbl)
      n138 = To Double Precision Float(number=w215) -> (double precision float=w214:dbl)
      n139 = property on="X Velocity SP step/sec" class="DigNum (strict)"("Minimum"=w218) -> ()  [unwired: 2 in, 2 out]
      n140 = Build Array(w218, w216, w214, w213, w209, w210, w211) -> (w212:dbl[])
      n141 = property on="X Velocity SP mm/sec" class="DigNum (strict)"("Val(Sgnl)"=w213) -> ()  [unwired: 2 in, 2 out]
      "X offset mm" <- w211
      "X steps/rev" <- w215
      "X mm/rev" <- w210
    }
  }
  n142 = local read "Z  velocity PV step/sec"() -> (w26:i32)
  n143 = flat-sequence {
    tunnel: [w224] -> w46
    frame #0 {
      w222 = 0.2 ("MM/rev")
      w227 = u32 51200 ("step/rev")
      w229 = 128000 ("Value (Signaling)")
      w230 = 1.0 ("Data Entry Limits:Minimum")
      w223 = 0.0 ("offset")
      n144 = property on="Y Velocity SP step/sec" class="DigNum (strict)"("Val(Sgnl)"=w229) -> ()  [unwired: 2 in, 2 out]
      n145 = To Double Precision Float(number=w227) -> (double precision float=w232:dbl)
      n146 = To Double Precision Float(number=w229) -> (double precision float=w221:dbl)
      n147 = Divide(x=w221, y=w232) -> (x/y=w231:dbl)
      n148 = property on="Y Velocity SP step/sec" class="DigNum (strict)"("Maximum"=w221) -> ()  [unwired: 2 in, 2 out]
      n149 = Multiply(x=w231, y=w222) -> (x*y=w225:dbl)
      n150 = To Double Precision Float(number=w229) -> (double precision float=w228:dbl)
      n151 = To Double Precision Float(number=w227) -> (double precision float=w226:dbl)
      n152 = property on="Y Velocity SP step/sec" class="DigNum (strict)"("Minimum"=w230) -> ()  [unwired: 2 in, 2 out]
      n153 = Build Array(w230, w228, w226, w225, w221, w222, w223) -> (w224:dbl[])
      n154 = property on="Y Velocity SP mm/sec" class="DigNum (strict)"("Val(Sgnl)"=w225) -> ()  [unwired: 2 in, 2 out]
      "Y offset mm" <- w223
      "Y steps/rev" <- w227
      "Y mm/rev" <- w222
    }
  }
  n155 = flat-sequence {
    frame #0 {
      n156 = property on="X Backlash corr" class="Bool (strict)"("Val(Sgnl)"=FALSE ("Value (Signaling)")) -> ()  [unwired: 2 in, 2 out]
      n157 = property on="Y Backlash corr" class="Bool (strict)"("Val(Sgnl)"=FALSE ("Value (Signaling)")) -> ()  [unwired: 2 in, 2 out]
      n158 = property on="R Backlash corr" class="Bool (strict)"("Val(Sgnl)"=FALSE ("Value (Signaling)")) -> ()  [unwired: 2 in, 2 out]
      n159 = property on="Z Backlash corr" class="Bool (strict)"("Val(Sgnl)"=FALSE ("Value (Signaling)")) -> ()  [unwired: 2 in, 2 out]
      "Z Backlash steps/sec" <- 25600 ("Z Backlash steps/sec")
      "Z Backlash" <- -12800 ("Z Backlash")
      "X Backlash steps/sec" <- 25600 ("Value (Signaling)")
      "X Backlash" <- 5120 ("Backlash2")
      "Y Backlash" <- -5120 ("Backlash2")
      "Y Backlash steps/sec" <- 25600 ("Value (Signaling)")
      "R Backlash steps/sec" <- 6400 ("R Backlash steps/sec")
      "R Backlash" <- -12800 ("R Backlash")
    }
  }
  n160 = flat-sequence {
    tunnel: [w245] -> w43
    frame #0 {
      w247 = 0.2 ("Z mm/rev")
      w251 = u32 51200 ("step/rev")
      w253 = 204800 ("Value (Signaling)")
      w254 = 1.0 ("Data Entry Limits:Minimum")
      w246 = 0.0 ("Z offset mm")
      n161 = property on="Z Velocity SP step/sec" class="DigNum (strict)"("Val(Sgnl)"=w253) -> ()  [unwired: 2 in, 2 out]
      n162 = To Double Precision Float(number=w251) -> (double precision float=w256:dbl)
      n163 = To Double Precision Float(number=w253) -> (double precision float=w249:dbl)
      n164 = Divide(x=w249, y=w256) -> (x/y=w255:dbl)
      n165 = property on="Z Velocity SP step/sec" class="DigNum (strict)"("Maximum"=w249) -> ()  [unwired: 2 in, 2 out]
      n166 = Multiply(x=w255, y=w247) -> (x*y=w248:dbl)
      n167 = To Double Precision Float(number=w251) -> (double precision float=w250:dbl)
      n168 = To Double Precision Float(number=w253) -> (double precision float=w252:dbl)
      n169 = Build Array(w254, w252, w250, w249, w248, w247, w246) -> (w245:dbl[])
      n170 = property on="Z Velocity SP mm/sec" class="DigNum (strict)"("Val(Sgnl)"=w248) -> ()  [unwired: 2 in, 2 out]
      n171 = property on="Z Velocity SP step/sec" class="DigNum (strict)"("Minimum"=w254) -> ()  [unwired: 2 in, 2 out]
      "Z offset mm" <- w246
      "Z mm/rev" <- w247
      "Z steps/rev" <- w251
    }
  }
  n172 = flat-sequence {
    tunnel: [w257] -> w42
    frame #0 {
      w260 = 20 ("R Holding Current %")
      w259 = 100 ("R Run Current %")
      w262 = 20 ("Holding Current %")
      w261 = 40 ("Run Current %")
      w264 = 20 ("Holding Current %")
      w265 = 40 ("Run Current %")
      w263 = 40 ("Z Run Current %")
      w258 = 20 ("Z Holding Current %")
      n173 = Build Array(w265, w264, w263, w262, w261, w260, w259, w258) -> (w257:i32[])
      "Z Holding Current %" <- w258
      "Z Run Current %" <- w263
      "X Run Current %" <- w265
      "X Holding Current %" <- w264
      "Y Run Current %" <- w261
      "Y Holding Current %" <- w262
      "R Holding Current %" <- w260
      "R Run Current %" <- w259
    }
  }
  n174 = flat-sequence {
    tunnel: [w266] -> w44
    frame #0 {
      w275 = 1.0 ("Data Entry Limits:Minimum")
      w269 = 0.0 ("R offset deg")
      w270 = -3.0 ("R deg/rev")
      w273 = u32 51200 ("step/rev")
      w274 = 20000 ("Value (Signaling)")
      n175 = property on="R Velocity SP step/sec" class="DigNum (strict)"("Val(Sgnl)"=w274) -> ()  [unwired: 2 in, 2 out]
      n176 = To Double Precision Float(number=w273) -> (double precision float=w276:dbl)
      n177 = To Double Precision Float(number=w274) -> (double precision float=w272:dbl)
      n178 = Divide(x=w272, y=w276) -> (x/y=w278:dbl)
      n179 = property on="R Velocity SP step/sec" class="DigNum (strict)"("Maximum"=w272) -> ()  [unwired: 2 in, 2 out]
      n180 = Multiply(x=w278, y=w270) -> (x*y=w277:dbl)
      n181 = To Double Precision Float(number=w273) -> (double precision float=w267:dbl)
      n182 = To Double Precision Float(number=w274) -> (double precision float=w268:dbl)
      n183 = Absolute Value(x=w277) -> (abs(x)=w271:dbl)
      n184 = Build Array(w275, w268, w267, w272, w271, w270, w269) -> (w266:dbl[])
      n185 = property on="R Velocity SP deg/sec" class="DigNum (strict)"("Val(Sgnl)"=w271) -> ()  [unwired: 2 in, 2 out]
      n186 = property on="R Velocity SP step/sec" class="DigNum (strict)"("Minimum"=w275) -> ()  [unwired: 2 in, 2 out]
      "R offset deg" <- w269
      "R deg/rev" <- w270
      "R steps/rev" <- w273
    }
  }
  n187 = local read "Y in Range"() -> (w32:bool)
  n188 = local read "Z in Range"() -> (w31:bool)
  n189 = local read "R in Range"() -> (w30:bool)
  n190 = local read "X velocity PV step/sec"() -> (w29:i32)
  n191 = local read "Y velocity PV step/sec"() -> (w27:i32)
  n192 = local read "R velocity PV step/sec"() -> (w28:i32)
  n193 = property on="Z Step SP" class="DigNum (strict)"("Minimum"=0.0 ("lower limit")) -> ()  [unwired: 2 in, 2 out]
  n194 = property on="R Step SP" class="DigNum (strict)"("Maximum"=0.0 ("Data Entry Limits:Maximum")) -> ()  [unwired: 2 in, 2 out]
  n195 = property on="R Step SP" class="DigNum (strict)"("Minimum"=-6144000.0 ("Data Entry Limits:Minimum")) -> ()  [unwired: 2 in, 2 out]
  n196 = property on="Z Step SP" class="DigNum (strict)"("Maximum"=102400000.0 ("upper limit")) -> ()  [unwired: 2 in, 2 out]
  n197 = Build Array(w33, w32, w31, w30) -> (→"XYZ in RANGE Array":bool[])
  n198 = Build Array("X Step SP", "Y Step SP", "Z Step SP", "R Step SP", "X Velocity SP step/sec", "Y Velocity SP step/sec", "Z Velocity SP step/sec", "R Velocity SP step/sec") -> (→"STEP SP Array":i32[])
  n199 = Build Array(w29, w27, w26, w28) -> (→"XYZR VEL PV Array":i32[])
  n200 = while {
    tunnel: [w306] -> w49
    tunnel: [w309] -> w50
    tunnel: [w312] -> w58
    tunnel: [w305] -> w57
    tunnel: [w311] -> w52
    tunnel: [w310] -> w51
    tunnel: [w308] -> w48
    tunnel: [w307] -> w47
    tunnel: w22 -> [w320]
    tunnel: w21 -> [w318]
    tunnel: w20 -> [w316]
    tunnel: w19 -> [w314]
    tunnel: w18 -> [w319]
    tunnel: w17 -> [w317]
    tunnel: w16 -> [w315]
    tunnel: w15 -> [w313]
    tunnel: w14 -> [w302]
    tunnel: w13 -> [w301]
    shift-right: [w295] -> _
    shift-left: dbl[] [] -> [w293]
    shift-right: [w294] -> _
    shift-left: dbl[] [] -> [w292]
    stop <- w303 stop-if-true
    # "XZYR"
    n201 = property on="Preset positions" class="Ring (strict)"() -> ("Strings []"=w296:string[])  [unwired: 2 in, 2 out]
    n202 = event shown="[16] \"LOOP\": Mouse Up" {
      selector: _ -> [_ _ _ _ _ _ _ _ _ _ _ _ _ _ _ _ _]
      dyn-events: _ -> [_ _ _ _ _ _ _ _ _ _ _ _ _ _ _ _ _]
      timeout: 100 -> [_ _ _ _ _ _ _ _ _ _ _ _ _ _ _ _ _]
      tunnel: w320 -> [w524 _ w1297 w1593 _ _ _ _ _ _ _ _ w2123 w2257 w2324 w2554 w2602]
      tunnel: w319 -> [w523 _ w1296 w1614 _ _ _ _ _ _ _ _ w2124 w2255 w2323 w2558 w2598]
      tunnel: w318 -> [w522 _ w1294 w1596 _ _ _ _ _ _ _ _ w2091 w2256 w2322 w2553 w2600]
      tunnel: w317 -> [w521 _ w1295 w1613 _ _ _ _ _ _ _ _ w2092 w2254 w2321 w2557 w2596]
      tunnel: w316 -> [w520 _ w1292 w1599 _ _ _ _ _ _ _ _ w2103 w2253 w2320 w2552 w2594]
      tunnel: w315 -> [w519 _ w1293 w1612 _ _ _ _ _ _ _ _ w2104 w2251 w2319 w2556 w2592]
      tunnel: w314 -> [w518 _ w1290 w1602 _ _ _ _ _ _ _ _ w2079 w2252 w2318 w2551 w2606]
      tunnel: w313 -> [w517 _ w1291 w1611 _ _ _ _ _ _ _ _ w2080 w2250 w2317 w2555 w2604]
      tunnel: [w500 _ _ _ _ _ _ _ _ _ _ _ _ _ _ _ _] -> w295
      tunnel: [w498 _ _ _ _ _ _ _ _ _ _ _ _ _ _ _ _] -> w294
      tunnel: w293 -> [w503 _ _ _ _ _ _ _ _ _ _ _ _ _ _ _ _]
      tunnel: w292 -> [w502 _ _ _ _ _ _ _ _ _ _ _ _ _ _ _ _]
      tunnel: [w496 _ w1275 _ _ _ _ _ _ _ _ _ _ _ _ _ _] -> w286
      tunnel: [w495 _ w1274 _ _ _ _ _ _ _ _ _ _ _ _ _ _] -> w283
      tunnel: [w494 _ w1273 _ _ _ _ _ _ _ _ _ _ _ _ _ _] -> w285
      tunnel: [w493 _ w1272 _ _ _ _ _ _ _ _ _ _ _ _ _ _] -> w284
      tunnel: [w490 _ w1271 _ _ _ _ _ _ _ _ _ _ _ _ _ _] -> w282
      tunnel: [w489 _ w1270 _ _ _ _ _ _ _ _ _ _ _ _ _ _] -> w281
      tunnel: [w492 _ w1269 _ _ _ _ _ _ _ _ _ _ _ _ _ _] -> w279
      tunnel: [_ _ w1268 _ _ _ _ _ _ _ _ _ _ _ _ _ _] -> w280
      tunnel: [w491 _ _ _ _ _ _ _ _ _ _ _ _ _ _ _ _] -> _
      event #0 {
        # "R"
        # "Y"
        # "Z"
        # "X"
        n203 = event-data() -> ()  [unwired: 1 in, 2 out]
        n204 = property on="X Position mm PV" class="DigNum (strict)"() -> ("Value"=w537:dbl)  [unwired: 2 in, 2 out]
        n205 = property on="Z Position mm PV" class="DigNum (strict)"() -> ("Value"=w506:dbl)  [unwired: 2 in, 2 out]
        n206 = property on="Y Position mm PV" class="DigNum (strict)"() -> ("Value"=w505:dbl)  [unwired: 2 in, 2 out]
        n207 = property on="R Position deg PV" class="DigNum (strict)"() -> ("Value"=w538:dbl)  [unwired: 2 in, 2 out]
        n208 = property on="GO" class="Bool"() -> ("DisabledEnum"=w513:T9)  [unwired: 2 in, 2 out]
        n209 = property on="Y Scan Length SP steps" class="DigNum (strict)"() -> ("Value"=w527:i32)  [unwired: 2 in, 2 out]
        n210 = property on="Z Scan Length SP steps" class="DigNum (strict)"() -> ("Value"=w528:i32)  [unwired: 2 in, 2 out]
        n211 = call "Build XY Graph2"("Reset"=TRUE, "Y Input"=w538, "X Input"=w506) -> ("XY Graph"=→"ZR Graph":cluster{"Y":dbl[], "Y":dbl[]}[])  [unwired: 7 in, 1 out]
        n212 = call "Build XY Graph"("Reset"=TRUE, "Y Input"=w505, "X Input"=w537) -> ("XY Graph"=→"XY Graph":cluster{"Y":dbl[], "Y":dbl[]}[])  [unwired: 7 in, 1 out]
        n213 = Build Array (concatenate)(w503, w506) -> (w501:dbl[])
        n214 = Build Array (concatenate)(w502, w505) -> (w499:dbl[])
        n215 = Equal?(x=w513, y=T9."Enabled") -> (x = y?=w511:bool)
        n216 = To Double Precision Float(number=w527) -> (double precision float=w526:dbl)
        n217 = To Double Precision Float(number=w528) -> (double precision float=w525:dbl)
        n218 = Bundle(w501, w499) -> (→"ZY Graph":cluster{dbl[], dbl[]})  [unwired: 1 in]
        n219 = property on="Clear ZY" class="Bool (strict)"() -> ("Value"=w497:bool)  [unwired: 2 in, 2 out]
        n220 = property on="Scan Go" class="Bool (strict)"() -> ("DisabledEnum"=w510:T9)  [unwired: 2 in, 2 out]
        n221 = case shown="False" w497 {
          tunnel: w501 -> [w542 w547]
          tunnel: [w542 w546] -> w500
          tunnel: w499 -> [w541 w545]
          tunnel: [w541 w544] -> w498
          frame #0 {
          }
          frame #1 {
            w543 = 0 ("dimension size")
            n222 = Reshape Array(w547, w543) -> (w546:dbl[])
            n223 = Reshape Array(w545, w543) -> (w544:dbl[])
          }
        }
        n224 = property on="GO" class="Bool"() -> ("DisabledEnum"=w516:T9)  [unwired: 2 in, 2 out]
        n225 = Divide(x=w526, y=w525) -> (x/y=w529:dbl)
        n226 = Equal?(x=w510, y=T9."Disabled and Grayed Out") -> (x = y?=w507:bool)
        n227 = Equal?(x=w516, y=T9."Disabled and Grayed Out") -> (x = y?=w514:bool)
        n228 = Inverse Tangent(1:w529) -> (0:w530:dbl)
        n229 = And(x=w511, y=w507) -> (x .and. y?=w508:bool)
        n230 = case shown="False" w507 {
          frame #0 {
            n231 = local write "STATUS"("SCANNING MODE" ("STATUS")) -> ()
          }
          frame #1 {
          }
        }
        n232 = case shown="True" w514 {
          tunnel: [w563 w610] -> w496
          tunnel: [w562 w609] -> w495
          tunnel: [w561 w608] -> w494
          tunnel: [w560 w607] -> w493
          tunnel: [w559 w606] -> w490
          tunnel: [w558 w605] -> w489
          tunnel: [w557 w604] -> w492
          tunnel: [w556 w603] -> w491
          tunnel: w524 -> [w571 w602]
          tunnel: w523 -> [w570 w601]
          tunnel: w522 -> [w569 w600]
          tunnel: w521 -> [w568 w599]
          tunnel: w520 -> [w567 w598]
          tunnel: w519 -> [w566 w597]
          tunnel: w518 -> [w565 w596]
          tunnel: w517 -> [w564 w595]
          frame #0 {
            n233 = call "DigitalIO_sub_V1_MON.vi"() -> ("CL"=w550:bool, "OP"=w551:bool)  [unwired: 8 in]
            n234 = property on="OP" class="Bool (strict)"("Val(Sgnl)"=w551) -> ()  [unwired: 2 in, 2 out]
            n235 = property on="CL" class="Bool (strict)"("Val(Sgnl)"=w550) -> ()  [unwired: 2 in, 2 out]
            n236 = call "mdrive send command.vi"("error in (no error)"=w570, "Extra"="MV", "Command"=T10."Print Parameter", "VISA resource name"=w571) -> ("error out"=w562:errorcluster, "read buffer"=w585:string, "VISA resource name out"=w563:refnum<visa-resource-name>)  [unwired: 3 in]
            n237 = call "mdrive send command.vi"("error in (no error)"=w568, "Extra"="MV", "Command"=T10."Print Parameter", "VISA resource name"=w569) -> ("error out"=w560:errorcluster, "read buffer"=w581:string, "VISA resource name out"=w561:refnum<visa-resource-name>)  [unwired: 3 in]
            n238 = call "mdrive send command.vi"("error in (no error)"=w566, "Extra"="MV", "Command"=T10."Print Parameter", "VISA resource name"=w567) -> ("error out"=w558:errorcluster, "read buffer"=w577:string, "VISA resource name out"=w559:refnum<visa-resource-name>)  [unwired: 3 in]
            n239 = call "mdrive send command.vi"("error in (no error)"=w564, "Extra"="MV", "Command"=T10."Print Parameter", "VISA resource name"=w565) -> ("error out"=w556:errorcluster, "read buffer"=w573:string, "VISA resource name out"=w557:refnum<visa-resource-name>)  [unwired: 3 in]
            n240 = Not Equal?(x=w585, y="") -> (x != y?=w555:bool)
            n241 = Not Equal?(x=w581, y="") -> (x != y?=w554:bool)
            n242 = Not Equal?(x=w577, y="") -> (x != y?=w553:bool)
            n243 = Not Equal?(x=w573, y="") -> (x != y?=w552:bool)
            n244 = property on="X Ready" class="Bool (strict)"("Val(Sgnl)"=w555) -> ()  [unwired: 2 in, 2 out]
            n245 = property on="Z Ready" class="Bool (strict)"("Val(Sgnl)"=w554) -> ()  [unwired: 2 in, 2 out]
            n246 = property on="Y Ready" class="Bool (strict)"("Val(Sgnl)"=w553) -> ()  [unwired: 2 in, 2 out]
            n247 = property on="R Ready" class="Bool (strict)"("Val(Sgnl)"=w552) -> ()  [unwired: 2 in, 2 out]
          }
          frame #1 {
            n248 = flat-sequence {
              tunnel: [w1123] -> w666
              tunnel: [w1122] -> w665
              tunnel: [w1121] -> w664
              tunnel: w602 -> [w1120]
              tunnel: w601 -> [w1119]
              tunnel: [w1145] -> w663
              tunnel: [w1144] -> w662
              tunnel: [w1142] -> w661
              tunnel: [w1143] -> w660
              tunnel: w666 -> [w1142]
              tunnel: w665 -> [w1141]
              tunnel: w664 -> [w1140]
              tunnel: w663 -> [w1159]
              tunnel: [w1159] -> w659
              tunnel: w662 -> [w1158]
              tunnel: [w1158] -> w658
              tunnel: w661 -> [w1157]
              tunnel: [w1157] -> w657
              tunnel: w660 -> [w1156]
              tunnel: [w1156] -> w656
              tunnel: [w1163] -> w655
              tunnel: [w1164] -> w654
              tunnel: [w1160] -> w653
              tunnel: w656 -> [w1160]
              tunnel: w657 -> [w1161]
              tunnel: w658 -> [w1165]
              tunnel: w659 -> [w1162]
              tunnel: w655 -> [w1175]
              tunnel: w654 -> [w1176]
              tunnel: w653 -> [w1178]
              tunnel: [w1174] -> w609
              tunnel: [w1173] -> w610
              frame #0 {
                n249 = property on="X Step SP" class="DigNum (strict)"() -> ("Maximum"=w1135:dbl)  [unwired: 2 in, 2 out]
                n250 = property on="X Step SP" class="DigNum (strict)"() -> ("Minimum"=w1137:dbl)  [unwired: 2 in, 2 out]
                n251 = property on="X steps/rev" class="DigNum (strict)"() -> ("Value"=w1132:u32)  [unwired: 2 in, 2 out]
                n252 = property on="X offset mm" class="DigNum (strict)"() -> ("Value"=w1128:dbl)  [unwired: 2 in, 2 out]
                n253 = To Long Integer(number=w1135) -> (32bit integer=w1134:i32)
                n254 = To Long Integer(number=w1137) -> (32bit integer=w1136:i32)
                n255 = To Double Precision Float(number=w1132) -> (double precision float=w1133:dbl)
                n256 = call "mdrive send command.vi"("error in (no error)"=w1119, "Extra"="P", "Command"=T10."Print Parameter", "VISA resource name"=w1120) -> ("error out"=w1121:errorcluster, "read buffer"=w1139:string, "VISA resource name out"=w1122:refnum<visa-resource-name>)  [unwired: 3 in]
                n257 = Decimal String To Number(string=w1139, offset=0) -> (number=w1118:i32)  [unwired: 1 in, 1 out]
                n258 = property on="X Step PV" class="DigNum (strict)"("Val(Sgnl)"=w1118) -> ()  [unwired: 2 in, 2 out]
                n259 = In Range and Coerce(upper limit=w1134, x=w1118, lower limit=w1136) -> (In Range?=w1123:bool)  [unwired: 1 out]
                n260 = To Double Precision Float(number=w1118) -> (double precision float=w1127:dbl)
                n261 = property on="X  in Range" class="Bool (strict)"("Val(Sgnl)"=w1123) -> ()  [unwired: 2 in, 2 out]
                n262 = Divide(x=w1127, y=w1133) -> (x/y=w1131:dbl)
                n263 = property on="X mm/rev" class="DigNum (strict)"() -> ("Value"=w1130:dbl)  [unwired: 2 in, 2 out]
                n264 = Multiply(x=w1131, y=w1130) -> (x*y=w1129:dbl)
                n265 = Add(x=w1129, y=w1128) -> (x+y=w1126:dbl)
                n266 = property on="X Position mm PV" class="DigNum (strict)"("Val(Sgnl)"=w1126) -> ()  [unwired: 2 in, 2 out]
              }
              frame #1 {
                n267 = call "mdrive send command.vi"("error in (no error)"=w1140, "Extra"="MV", "Command"=T10."Print Parameter", "VISA resource name"=w1141) -> ("error out"=w1144:errorcluster, "read buffer"=w1148:string, "VISA resource name out"=w1145:refnum<visa-resource-name>)  [unwired: 3 in]
                n268 = Decimal String To Number(string=w1148, offset=0 ("offset (0)")) -> (number=w1151:i32)  [unwired: 1 in, 1 out]
                n269 = Not Equal?(x=w1148, y="") -> (x != y?=w1146:bool)
                n270 = property on="X Ready" class="Bool (strict)"("Val(Sgnl)"=w1146) -> ()  [unwired: 2 in, 2 out]
                n271 = Number To Boolean Array(number=w1151) -> (Boolean array=w1150:bool[])
                n272 = Index Array(array=w1150, index=0) -> (element=w1143:bool)
                n273 = property on="X  in Motion" class="Bool (strict)"("Val(Sgnl)"=w1143) -> ()  [unwired: 2 in, 2 out]
              }
              frame #2 {
                n274 = Wait (ms)(milliseconds to wait=u32 50) -> ()  [unwired: 1 out]
              }
              frame #3 {
                n275 = case shown="True" w1161 {
                  tunnel: w1162 -> [w1168 w1172]
                  tunnel: [w1169 w1172] -> w1163
                  tunnel: [w1170 w1171] -> w1164
                  tunnel: w1165 -> [w1167 w1171]
                  frame #0 {
                    n276 = call "mdrive send command.vi"("error in (no error)"=w1167, "Command"=T10."Stop", "VISA resource name"=w1168) -> ("error out"=w1170:errorcluster, "VISA resource name out"=w1169:refnum<visa-resource-name>)  [unwired: 4 in, 1 out]
                  }
                  frame #1 {
                  }
                }
              }
              frame #4 {
                n277 = property on="X Backlash corr" class="Bool (strict)"() -> ("Value"=w1179:bool)  [unwired: 2 in, 2 out]
                n278 = Implies(1:w1178, 2:w1179) -> (0:w1177:bool)
                n279 = case shown="False" w1177 {
                  tunnel: w1176 -> [w1187 w1244]
                  tunnel: w1175 -> [w1186 w1245]
                  tunnel: [w1181 w1244] -> w1174
                  tunnel: [w1185 w1245] -> w1173
                  frame #0 {
                    # "Backlash"
                    n280 = flat-sequence {
                      tunnel: [w1202] -> w1199
                      tunnel: [w1204] -> w1198
                      tunnel: [w1203] -> w1197
                      tunnel: w1187 -> [w1201]
                      tunnel: w1186 -> [w1200]
                      tunnel: w1199 -> [w1212]
                      tunnel: [w1212] -> w1196
                      tunnel: w1198 -> [w1211]
                      tunnel: w1197 -> [w1210]
                      tunnel: [w1209] -> w1195
                      tunnel: [w1208] -> w1194
                      tunnel: [w1207] -> w1184
                      tunnel: w1196 -> [w1226]
                      tunnel: w1195 -> [w1217]
                      tunnel: w1194 -> [w1225]
                      tunnel: [w1217] -> w1193
                      tunnel: [w1225] -> w1192
                      tunnel: [w1216] -> w1189
                      tunnel: [w1224] -> w1188
                      tunnel: w1184 -> [w1224]
                      tunnel: w1193 -> [w1229]
                      tunnel: w1192 -> [w1230]
                      tunnel: [w1228] -> w1191
                      tunnel: [w1236] -> w1190
                      tunnel: w1189 -> [w1236]
                      tunnel: w1188 -> [w1232]
                      tunnel: [w1231] -> w1182
                      tunnel: w1191 -> [w1239]
                      tunnel: w1190 -> [w1238]
                      tunnel: [w1240] -> w1183
                      tunnel: w1182 -> [w1240]
                      tunnel: [w1239] -> w1180
                      tunnel: [w1243] -> w1185
                      tunnel: w1183 -> [w1243]
                      tunnel: [w1241] -> w1181
                      tunnel: w1180 -> [w1241]
                      frame #0 {
                        n281 = property on="X Backlash steps/sec" class="DigNum (strict)"() -> ("Value"=w1202:i32)  [unwired: 2 in, 2 out]
                        n282 = Number To Decimal String(number=w1202) -> (decimal integer string=w1205:string)  [unwired: 1 in]
                        n283 = call "mdrive send command.vi"("error in (no error)"=w1201, "Extra"=w1205, "Command"=T10."Max Velocity", "VISA resource name"=w1200) -> ("error out"=w1203:errorcluster, "VISA resource name out"=w1204:refnum<visa-resource-name>)  [unwired: 3 in, 1 out]
                      }
                      frame #1 {
                        n284 = property on="X Backlash" class="DigNum (strict)"() -> ("Value"=w1207:i32)  [unwired: 2 in, 2 out]
                        n285 = Number To Decimal String(number=w1207) -> (decimal integer string=w1213:string)  [unwired: 1 in]
                        n286 = call "mdrive send command.vi"("error in (no error)"=w1210, "Extra"=w1213, "Command"=T10."Move to Relative Position", "VISA resource name"=w1211) -> ("error out"=w1209:errorcluster, "VISA resource name out"=w1208:refnum<visa-resource-name>)  [unwired: 3 in, 1 out]
                      }
                      frame #2 {
                        n287 = To Double Precision Float(number=w1224) -> (double precision float=w1222:dbl)
                        n288 = To Double Precision Float(number=w1226) -> (double precision float=w1227:dbl)
                        n289 = Absolute Value(x=w1222) -> (abs(x)=w1223:dbl)
                        n290 = Divide(x=w1223, y=w1227) -> (x/y=w1220:dbl)
                        n291 = Multiply(x=1000.0, y=w1220) -> (x*y=w1218:dbl)
                        n292 = Add(x=w1218, y=300.0) -> (x+y=w1216:dbl)
                        n293 = To Unsigned Long Integer(number=w1216) -> (unsigned 32bit integer=w1215:u32)
                        n294 = Wait (ms)(milliseconds to wait=w1215) -> ()  [unwired: 1 out]
                      }
                      frame #3 {
                        n295 = Negate(x=w1232) -> (-x=w1233:i32)
                        n296 = Number To Decimal String(number=w1233) -> (decimal integer string=w1234:string)  [unwired: 1 in]
                        n297 = call "mdrive send command.vi"("error in (no error)"=w1229, "Extra"=w1234, "Command"=T10."Move to Relative Position", "VISA resource name"=w1230) -> ("error out"=w1228:errorcluster, "VISA resource name out"=w1231:refnum<visa-resource-name>)  [unwired: 3 in, 1 out]
                      }
                      frame #4 {
                        n298 = To Unsigned Long Integer(number=w1238) -> (unsigned 32bit integer=w1237:u32)
                        n299 = Wait (ms)(milliseconds to wait=w1237) -> ()  [unwired: 1 out]
                      }
                      frame #5 {
                        n300 = property on="X Backlash corr" class="Bool (strict)"("Val(Sgnl)"=FALSE ("Value (Signaling)")) -> ()  [unwired: 2 in, 2 out]
                      }
                    }
                  }
                  frame #1 {
                  }
                }
              }
            }
            n301 = flat-sequence {
              tunnel: [w989] -> w652
              tunnel: [w980] -> w651
              tunnel: [w979] -> w650
              tunnel: w600 -> [w983]
              tunnel: w599 -> [w982]
              tunnel: [w1021] -> w649
              tunnel: [w1020] -> w648
              tunnel: [w1019] -> w647
              tunnel: [w1012] -> w646
              tunnel: w652 -> [w1019]
              tunnel: w651 -> [w1018]
              tunnel: w650 -> [w1017]
              tunnel: w649 -> [w1031]
              tunnel: [w1031] -> w645
              tunnel: w648 -> [w1030]
              tunnel: [w1030] -> w644
              tunnel: w647 -> [w1029]
              tunnel: [w1029] -> w643
              tunnel: w646 -> [w1028]
              tunnel: [w1028] -> w642
              tunnel: [w1035] -> w641
              tunnel: [w1036] -> w640
              tunnel: [w1032] -> w639
              tunnel: w642 -> [w1032]
              tunnel: w643 -> [w1033]
              tunnel: w644 -> [w1037]
              tunnel: w645 -> [w1034]
              tunnel: w641 -> [w1048]
              tunnel: w640 -> [w1049]
              tunnel: w639 -> [w1051]
              tunnel: [w1047] -> w607
              tunnel: [w1046] -> w608
              frame #0 {
                n302 = property on="Z Step SP" class="DigNum (strict)"() -> ("Maximum"=w990:dbl)  [unwired: 2 in, 2 out]
                n303 = property on="Z Step SP" class="DigNum (strict)"() -> ("Minimum"=w984:dbl)  [unwired: 2 in, 2 out]
                n304 = property on="OK Button" class="Bool (strict)"() -> ("Value"=w975:bool)  [unwired: 2 in, 2 out]
                n305 = property on="Z steps/rev" class="DigNum (strict)"() -> ("Value"=w988:u32)  [unwired: 2 in, 2 out]
                n306 = To Double Precision Float(number=w988) -> (double precision float=w995:dbl)
                n307 = To Long Integer(number=w990) -> (32bit integer=w996:i32)
                n308 = To Long Integer(number=w984) -> (32bit integer=w997:i32)
                n309 = property on="Z offset mm" class="DigNum (strict)"() -> ("Value"=w986:dbl)  [unwired: 2 in, 2 out]
                n310 = Not Equal?(x=w975, y=TRUE) -> (x != y?=w973:bool)
                n311 = call "mdrive send command.vi"("error in (no error)"=w982, "Extra"="P", "Command"=T10."Print Parameter", "VISA resource name"=w983) -> ("error out"=w979:errorcluster, "read buffer"=w999:string, "VISA resource name out"=w980:refnum<visa-resource-name>)  [unwired: 3 in]
                n312 = Decimal String To Number(string=w999, offset=0) -> (number=w978:i32)  [unwired: 1 in, 1 out]
                n313 = property on="Z Step PV" class="DigNum (strict)"("Val(Sgnl)"=w978) -> ()  [unwired: 2 in, 2 out]
                n314 = Equal?(x=w978, y=15360000) -> (x = y?=w972:bool)
                n315 = To Double Precision Float(number=w978) -> (double precision float=w993:dbl)
                n316 = In Range and Coerce(upper limit=w996, x=w978, lower limit=w997) -> (In Range?=w989:bool)  [unwired: 1 out]
                n317 = property on="Z in Range" class="Bool (strict)"("Val(Sgnl)"=w989) -> ()  [unwired: 2 in, 2 out]
                n318 = Divide(x=w993, y=w995) -> (x/y=w994:dbl)
                n319 = And(x=w972, y=w973) -> (x .and. y?=w971:bool)
                n320 = case shown="True" w971 {
                  tunnel: [FALSE ("true") w1010] -> w976
                  frame #0 {
                  }
                  frame #1 {
                    n321 = One Button Dialog(message="HAVE YOU OPEND THE VALVE???\nTHEN REWRITE YOUR POSITION\n AND PRESS GO!") -> (true=w1010:bool)  [unwired: 1 in]
                  }
                }
                n322 = property on="Z mm/rev" class="DigNum (strict)"() -> ("Value"=w987:dbl)  [unwired: 2 in, 2 out]
                n323 = Multiply(x=w994, y=w987) -> (x*y=w981:dbl)
                n324 = Add(x=w981, y=w986) -> (x+y=w985:dbl)
                n325 = property on="Z Position mm PV" class="DigNum (strict)"("Val(Sgnl)"=w985) -> ()  [unwired: 2 in, 2 out]
                n326 = case shown="True" w976 {
                  frame #0 {
                    n327 = call "DigitalIO_sub_V1_MON.vi"() -> ("CL"=w1000:bool, "OP"=w1001:bool)  [unwired: 8 in]
                    n328 = property on="OP" class="Bool (strict)"("Val(Sgnl)"=w1001) -> ()  [unwired: 2 in, 2 out]
                    n329 = property on="CL" class="Bool (strict)"("Val(Sgnl)"=w1000) -> ()  [unwired: 2 in, 2 out]
                  }
                  frame #1 {
                    n330 = while {
                      stop <- w1008 stop-if-true
                      n331 = property on="OK Button" class="Bool (strict)"() -> ("Value"=w1002:bool)  [unwired: 2 in, 2 out]
                      n332 = call "ValveConrtoller.vi"("OK Button"=w1002) -> ("OUTGOING SIGNAL"=w1003:bool, "CL"=w1004:bool, "OP"=w1005:bool, "VALVE\nopend/closed"=w1006:bool)  [unwired: 3 in]
                      n333 = property on="OP" class="Bool (strict)"("Val(Sgnl)"=w1005) -> ()  [unwired: 2 in, 2 out]
                      n334 = property on="CL" class="Bool (strict)"("Val(Sgnl)"=w1004) -> ()  [unwired: 2 in, 2 out]
                      n335 = property on="Valve \nopend/closed" class="Bool (strict)"("Val(Sgnl)"=w1006) -> ()  [unwired: 2 in, 2 out]
                      n336 = Equal?(x=w1003, y=TRUE) -> (x = y?=w1008:bool)
                    }
                  }
                }
              }
              frame #1 {
                n337 = call "mdrive send command.vi"("error in (no error)"=w1017, "Extra"="MV", "Command"=T10."Print Parameter", "VISA resource name"=w1018) -> ("error out"=w1020:errorcluster, "read buffer"=w1023:string, "VISA resource name out"=w1021:refnum<visa-resource-name>)  [unwired: 3 in]
                n338 = Decimal String To Number(string=w1023, offset=0 ("offset (0)")) -> (number=w1013:i32)  [unwired: 1 in, 1 out]
                n339 = Not Equal?(x=w1023, y="") -> (x != y?=w1016:bool)
                n340 = property on="Z Ready" class="Bool (strict)"("Val(Sgnl)"=w1016) -> ()  [unwired: 2 in, 2 out]
                n341 = Number To Boolean Array(number=w1013) -> (Boolean array=w1015:bool[])
                n342 = Index Array(array=w1015, index=0) -> (element=w1012:bool)
                n343 = property on="Z in Motion" class="Bool (strict)"("Val(Sgnl)"=w1012) -> ()  [unwired: 2 in, 2 out]
              }
              frame #2 {
                n344 = Wait (ms)(milliseconds to wait=u32 50) -> ()  [unwired: 1 out]
              }
              frame #3 {
                n345 = case shown="False" w1033 {
                  tunnel: w1034 -> [w1040 w1044]
                  tunnel: [w1041 w1044] -> w1035
                  tunnel: [w1042 w1043] -> w1036
                  tunnel: w1037 -> [w1039 w1043]
                  frame #0 {
                    n346 = call "mdrive send command.vi"("error in (no error)"=w1039, "Command"=T10."Stop", "VISA resource name"=w1040) -> ("error out"=w1042:errorcluster, "VISA resource name out"=w1041:refnum<visa-resource-name>)  [unwired: 4 in, 1 out]
                  }
                  frame #1 {
                  }
                }
              }
              frame #4 {
                n347 = property on="Z Backlash corr" class="Bool (strict)"() -> ("Value"=w1045:bool)  [unwired: 2 in, 2 out]
                n348 = Implies(1:w1051, 2:w1045) -> (0:w1050:bool)
                n349 = case shown="False" w1050 {
                  tunnel: w1049 -> [w1059 w1116]
                  tunnel: w1048 -> [w1058 w1117]
                  tunnel: [w1053 w1116] -> w1047
                  tunnel: [w1057 w1117] -> w1046
                  frame #0 {
                    # "Backlash"
                    n350 = flat-sequence {
                      tunnel: [w1072] -> w1071
                      tunnel: [w1076] -> w1070
                      tunnel: [w1075] -> w1069
                      tunnel: w1059 -> [w1074]
                      tunnel: w1058 -> [w1073]
                      tunnel: w1071 -> [w1084]
                      tunnel: [w1084] -> w1068
                      tunnel: w1070 -> [w1083]
                      tunnel: w1069 -> [w1082]
                      tunnel: [w1081] -> w1067
                      tunnel: [w1080] -> w1066
                      tunnel: [w1079] -> w1056
                      tunnel: w1068 -> [w1098]
                      tunnel: w1067 -> [w1089]
                      tunnel: w1066 -> [w1097]
                      tunnel: [w1089] -> w1065
                      tunnel: [w1097] -> w1064
                      tunnel: [w1088] -> w1061
                      tunnel: [w1096] -> w1060
                      tunnel: w1056 -> [w1096]
                      tunnel: w1065 -> [w1101]
                      tunnel: w1064 -> [w1102]
                      tunnel: [w1100] -> w1063
                      tunnel: [w1108] -> w1062
                      tunnel: w1061 -> [w1108]
                      tunnel: w1060 -> [w1104]
                      tunnel: [w1103] -> w1054
                      tunnel: w1063 -> [w1111]
                      tunnel: w1062 -> [w1110]
                      tunnel: [w1112] -> w1055
                      tunnel: w1054 -> [w1112]
                      tunnel: [w1111] -> w1052
                      tunnel: [w1115] -> w1057
                      tunnel: w1055 -> [w1115]
                      tunnel: [w1114] -> w1053
                      tunnel: w1052 -> [w1114]
                      frame #0 {
                        n351 = property on="Z Backlash steps/sec" class="DigNum (strict)"() -> ("Value"=w1072:i32)  [unwired: 2 in, 2 out]
                        n352 = Number To Decimal String(number=w1072) -> (decimal integer string=w1077:string)  [unwired: 1 in]
                        n353 = call "mdrive send command.vi"("error in (no error)"=w1074, "Extra"=w1077, "Command"=T10."Max Velocity", "VISA resource name"=w1073) -> ("error out"=w1075:errorcluster, "VISA resource name out"=w1076:refnum<visa-resource-name>)  [unwired: 3 in, 1 out]
                      }
                      frame #1 {
                        n354 = property on="Z Backlash" class="DigNum (strict)"() -> ("Value"=w1079:i32)  [unwired: 2 in, 2 out]
                        n355 = Number To Decimal String(number=w1079) -> (decimal integer string=w1085:string)  [unwired: 1 in]
                        n356 = call "mdrive send command.vi"("error in (no error)"=w1082, "Extra"=w1085, "Command"=T10."Move to Relative Position", "VISA resource name"=w1083) -> ("error out"=w1081:errorcluster, "VISA resource name out"=w1080:refnum<visa-resource-name>)  [unwired: 3 in, 1 out]
                      }
                      frame #2 {
                        n357 = To Double Precision Float(number=w1096) -> (double precision float=w1094:dbl)
                        n358 = To Double Precision Float(number=w1098) -> (double precision float=w1099:dbl)
                        n359 = Absolute Value(x=w1094) -> (abs(x)=w1095:dbl)
                        n360 = Divide(x=w1095, y=w1099) -> (x/y=w1092:dbl)
                        n361 = Multiply(x=1000.0, y=w1092) -> (x*y=w1090:dbl)
                        n362 = Add(x=w1090, y=300.0) -> (x+y=w1088:dbl)
                        n363 = To Unsigned Long Integer(number=w1088) -> (unsigned 32bit integer=w1087:u32)
                        n364 = Wait (ms)(milliseconds to wait=w1087) -> ()  [unwired: 1 out]
                      }
                      frame #3 {
                        n365 = Negate(x=w1104) -> (-x=w1105:i32)
                        n366 = Number To Decimal String(number=w1105) -> (decimal integer string=w1106:string)  [unwired: 1 in]
                        n367 = call "mdrive send command.vi"("error in (no error)"=w1101, "Extra"=w1106, "Command"=T10."Move to Relative Position", "VISA resource name"=w1102) -> ("error out"=w1100:errorcluster, "VISA resource name out"=w1103:refnum<visa-resource-name>)  [unwired: 3 in, 1 out]
                      }
                      frame #4 {
                        n368 = To Unsigned Long Integer(number=w1110) -> (unsigned 32bit integer=w1109:u32)
                        n369 = Wait (ms)(milliseconds to wait=w1109) -> ()  [unwired: 1 out]
                      }
                      frame #5 {
                        n370 = property on="Z Backlash corr" class="Bool (strict)"("Val(Sgnl)"=FALSE ("Value (Signaling)")) -> ()  [unwired: 2 in, 2 out]
                      }
                    }
                  }
                  frame #1 {
                  }
                }
              }
            }
            n371 = flat-sequence {
              tunnel: [w852] -> w638
              tunnel: [w854] -> w637
              tunnel: [w853] -> w636
              tunnel: w598 -> [w845]
              tunnel: w597 -> [w844]
              tunnel: [w874] -> w635
              tunnel: [w873] -> w634
              tunnel: [w872] -> w633
              tunnel: [w865] -> w632
              tunnel: w638 -> [w872]
              tunnel: w637 -> [w871]
              tunnel: w636 -> [w870]
              tunnel: w635 -> [w884]
              tunnel: [w884] -> w631
              tunnel: w634 -> [w883]
              tunnel: [w883] -> w630
              tunnel: w633 -> [w882]
              tunnel: [w882] -> w629
              tunnel: w632 -> [w881]
              tunnel: [w881] -> w628
              tunnel: [w888] -> w627
              tunnel: [w889] -> w626
              tunnel: [w885] -> w625
              tunnel: w628 -> [w885]
              tunnel: w629 -> [w886]
              tunnel: w630 -> [w890]
              tunnel: w631 -> [w887]
              tunnel: w627 -> [w901]
              tunnel: w626 -> [w902]
              tunnel: w625 -> [w904]
              tunnel: [w900] -> w605
              tunnel: [w899] -> w606
              frame #0 {
                n372 = property on="Y Step SP" class="DigNum (strict)"() -> ("Maximum"=w847:dbl)  [unwired: 2 in, 2 out]
                n373 = property on="Y Step SP" class="DigNum (strict)"() -> ("Minimum"=w846:dbl)  [unwired: 2 in, 2 out]
                n374 = property on="Y steps/rev" class="DigNum (strict)"() -> ("Value"=w848:u32)  [unwired: 2 in, 2 out]
                n375 = property on="Y offset mm" class="DigNum (strict)"() -> ("Value"=w850:dbl)  [unwired: 2 in, 2 out]
                n376 = To Long Integer(number=w847) -> (32bit integer=w861:i32)
                n377 = To Long Integer(number=w846) -> (32bit integer=w862:i32)
                n378 = To Double Precision Float(number=w848) -> (double precision float=w860:dbl)
                n379 = call "mdrive send command.vi"("error in (no error)"=w844, "Extra"="P", "Command"=T10."Print Parameter", "VISA resource name"=w845) -> ("error out"=w853:errorcluster, "read buffer"=w864:string, "VISA resource name out"=w854:refnum<visa-resource-name>)  [unwired: 3 in]
                n380 = Decimal String To Number(string=w864, offset=0) -> (number=w843:i32)  [unwired: 1 in, 1 out]
                n381 = property on="Y Step PV" class="DigNum (strict)"("Val(Sgnl)"=w843) -> ()  [unwired: 2 in, 2 out]
                n382 = In Range and Coerce(upper limit=w861, x=w843, lower limit=w862) -> (In Range?=w852:bool)  [unwired: 1 out]
                n383 = To Double Precision Float(number=w843) -> (double precision float=w857:dbl)
                n384 = property on="Y in Range" class="Bool (strict)"("Val(Sgnl)"=w852) -> ()  [unwired: 2 in, 2 out]
                n385 = Divide(x=w857, y=w860) -> (x/y=w859:dbl)
                n386 = property on="Y mm/rev" class="DigNum (strict)"() -> ("Value"=w849:dbl)  [unwired: 2 in, 2 out]
                n387 = Multiply(x=w859, y=w849) -> (x*y=w858:dbl)
                n388 = Add(x=w858, y=w850) -> (x+y=w851:dbl)
                n389 = property on="Y Position mm PV" class="DigNum (strict)"("Val(Sgnl)"=w851) -> ()  [unwired: 2 in, 2 out]
              }
              frame #1 {
                n390 = call "mdrive send command.vi"("error in (no error)"=w870, "Extra"="MV", "Command"=T10."Print Parameter", "VISA resource name"=w871) -> ("error out"=w873:errorcluster, "read buffer"=w876:string, "VISA resource name out"=w874:refnum<visa-resource-name>)  [unwired: 3 in]
                n391 = Decimal String To Number(string=w876, offset=0 ("offset (0)")) -> (number=w866:i32)  [unwired: 1 in, 1 out]
                n392 = Not Equal?(x=w876, y="") -> (x != y?=w869:bool)
                n393 = property on="Y Ready" class="Bool (strict)"("Val(Sgnl)"=w869) -> ()  [unwired: 2 in, 2 out]
                n394 = Number To Boolean Array(number=w866) -> (Boolean array=w868:bool[])
                n395 = Index Array(array=w868, index=0) -> (element=w865:bool)
                n396 = property on="Y in Motion" class="Bool (strict)"("Val(Sgnl)"=w865) -> ()  [unwired: 2 in, 2 out]
              }
              frame #2 {
                n397 = Wait (ms)(milliseconds to wait=u32 50) -> ()  [unwired: 1 out]
              }
              frame #3 {
                n398 = case shown="True" w886 {
                  tunnel: w887 -> [w893 w896]
                  tunnel: [w894 w896] -> w888
                  tunnel: [w895 w897] -> w889
                  tunnel: w890 -> [w892 w897]
                  frame #0 {
                    n399 = call "mdrive send command.vi"("error in (no error)"=w892, "Command"=T10."Stop", "VISA resource name"=w893) -> ("error out"=w895:errorcluster, "VISA resource name out"=w894:refnum<visa-resource-name>)  [unwired: 4 in, 1 out]
                  }
                  frame #1 {
                  }
                }
              }
              frame #4 {
                n400 = property on="Y Backlash corr" class="Bool (strict)"() -> ("Value"=w898:bool)  [unwired: 2 in, 2 out]
                n401 = Implies(1:w904, 2:w898) -> (0:w903:bool)
                n402 = case shown="False" w903 {
                  tunnel: w902 -> [w912 w969]
                  tunnel: w901 -> [w911 w970]
                  tunnel: [w906 w969] -> w900
                  tunnel: [w910 w970] -> w899
                  frame #0 {
                    # "Backlash"
                    n403 = flat-sequence {
                      tunnel: [w925] -> w924
                      tunnel: [w929] -> w923
                      tunnel: [w928] -> w922
                      tunnel: w912 -> [w927]
                      tunnel: w911 -> [w926]
                      tunnel: w924 -> [w937]
                      tunnel: [w937] -> w921
                      tunnel: w923 -> [w936]
                      tunnel: w922 -> [w935]
                      tunnel: [w934] -> w920
                      tunnel: [w933] -> w919
                      tunnel: [w932] -> w909
                      tunnel: w921 -> [w951]
                      tunnel: w920 -> [w942]
                      tunnel: w919 -> [w950]
                      tunnel: [w942] -> w918
                      tunnel: [w950] -> w917
                      tunnel: [w941] -> w914
                      tunnel: [w949] -> w913
                      tunnel: w909 -> [w949]
                      tunnel: w918 -> [w954]
                      tunnel: w917 -> [w955]
                      tunnel: [w953] -> w916
                      tunnel: [w961] -> w915
                      tunnel: w914 -> [w961]
                      tunnel: w913 -> [w957]
                      tunnel: [w956] -> w907
                      tunnel: w916 -> [w964]
                      tunnel: w915 -> [w963]
                      tunnel: [w965] -> w908
                      tunnel: w907 -> [w965]
                      tunnel: [w964] -> w905
                      tunnel: [w968] -> w910
                      tunnel: w908 -> [w968]
                      tunnel: [w967] -> w906
                      tunnel: w905 -> [w967]
                      frame #0 {
                        n404 = property on="Y Backlash steps/sec" class="DigNum (strict)"() -> ("Value"=w925:i32)  [unwired: 2 in, 2 out]
                        n405 = Number To Decimal String(number=w925) -> (decimal integer string=w930:string)  [unwired: 1 in]
                        n406 = call "mdrive send command.vi"("error in (no error)"=w927, "Extra"=w930, "Command"=T10."Max Velocity", "VISA resource name"=w926) -> ("error out"=w928:errorcluster, "VISA resource name out"=w929:refnum<visa-resource-name>)  [unwired: 3 in, 1 out]
                      }
                      frame #1 {
                        n407 = property on="Y Backlash" class="DigNum (strict)"() -> ("Value"=w932:i32)  [unwired: 2 in, 2 out]
                        n408 = Number To Decimal String(number=w932) -> (decimal integer string=w938:string)  [unwired: 1 in]
                        n409 = call "mdrive send command.vi"("error in (no error)"=w935, "Extra"=w938, "Command"=T10."Move to Relative Position", "VISA resource name"=w936) -> ("error out"=w934:errorcluster, "VISA resource name out"=w933:refnum<visa-resource-name>)  [unwired: 3 in, 1 out]
                      }
                      frame #2 {
                        n410 = To Double Precision Float(number=w949) -> (double precision float=w947:dbl)
                        n411 = To Double Precision Float(number=w951) -> (double precision float=w952:dbl)
                        n412 = Absolute Value(x=w947) -> (abs(x)=w948:dbl)
                        n413 = Divide(x=w948, y=w952) -> (x/y=w945:dbl)
                        n414 = Multiply(x=1000.0, y=w945) -> (x*y=w943:dbl)
                        n415 = Add(x=w943, y=300.0) -> (x+y=w941:dbl)
                        n416 = To Unsigned Long Integer(number=w941) -> (unsigned 32bit integer=w940:u32)
                        n417 = Wait (ms)(milliseconds to wait=w940) -> ()  [unwired: 1 out]
                      }
                      frame #3 {
                        n418 = Negate(x=w957) -> (-x=w958:i32)
                        n419 = Number To Decimal String(number=w958) -> (decimal integer string=w959:string)  [unwired: 1 in]
                        n420 = call "mdrive send command.vi"("error in (no error)"=w954, "Extra"=w959, "Command"=T10."Move to Relative Position", "VISA resource name"=w955) -> ("error out"=w953:errorcluster, "VISA resource name out"=w956:refnum<visa-resource-name>)  [unwired: 3 in, 1 out]
                      }
                      frame #4 {
                        n421 = To Unsigned Long Integer(number=w963) -> (unsigned 32bit integer=w962:u32)
                        n422 = Wait (ms)(milliseconds to wait=w962) -> ()  [unwired: 1 out]
                      }
                      frame #5 {
                        n423 = property on="Y Backlash corr" class="Bool (strict)"("Val(Sgnl)"=FALSE ("Value (Signaling)")) -> ()  [unwired: 2 in, 2 out]
                      }
                    }
                  }
                  frame #1 {
                  }
                }
              }
            }
            n424 = flat-sequence {
              tunnel: [w724] -> w624
              tunnel: [w726] -> w623
              tunnel: [w725] -> w622
              tunnel: w596 -> [w717]
              tunnel: w595 -> [w716]
              tunnel: [w746] -> w621
              tunnel: [w745] -> w620
              tunnel: [w744] -> w619
              tunnel: [w737] -> w618
              tunnel: w624 -> [w744]
              tunnel: w623 -> [w743]
              tunnel: w622 -> [w742]
              tunnel: w621 -> [w756]
              tunnel: [w756] -> w617
              tunnel: w620 -> [w755]
              tunnel: [w755] -> w616
              tunnel: w619 -> [w754]
              tunnel: [w754] -> w615
              tunnel: w618 -> [w753]
              tunnel: [w753] -> w614
              tunnel: [w760] -> w613
              tunnel: [w761] -> w612
              tunnel: [w757] -> w611
              tunnel: w614 -> [w757]
              tunnel: w615 -> [w758]
              tunnel: w616 -> [w762]
              tunnel: w617 -> [w759]
              tunnel: w613 -> [w773]
              tunnel: w612 -> [w774]
              tunnel: w611 -> [w776]
              tunnel: [w772] -> w603
              tunnel: [w771] -> w604
              frame #0 {
                n425 = property on="R Step SP" class="DigNum (strict)"() -> ("Maximum"=w719:dbl)  [unwired: 2 in, 2 out]
                n426 = property on="R Step SP" class="DigNum (strict)"() -> ("Minimum"=w720:dbl)  [unwired: 2 in, 2 out]
                n427 = property on="R steps/rev" class="DigNum (strict)"() -> ("Value"=w718:u32)  [unwired: 2 in, 2 out]
                n428 = property on="R offset deg" class="DigNum (strict)"() -> ("Value"=w722:dbl)  [unwired: 2 in, 2 out]
                n429 = To Long Integer(number=w719) -> (32bit integer=w733:i32)
                n430 = To Long Integer(number=w720) -> (32bit integer=w734:i32)
                n431 = To Double Precision Float(number=w718) -> (double precision float=w732:dbl)
                n432 = call "mdrive send command.vi"("error in (no error)"=w716, "Extra"="P", "Command"=T10."Print Parameter", "VISA resource name"=w717) -> ("error out"=w725:errorcluster, "read buffer"=w736:string, "VISA resource name out"=w726:refnum<visa-resource-name>)  [unwired: 3 in]
                n433 = Decimal String To Number(string=w736, offset=0) -> (number=w715:i32)  [unwired: 1 in, 1 out]
                n434 = property on="R Step PV" class="DigNum (strict)"("Val(Sgnl)"=w715) -> ()  [unwired: 2 in, 2 out]
                n435 = In Range and Coerce(upper limit=w733, x=w715, lower limit=w734) -> (In Range?=w724:bool)  [unwired: 1 out]
                n436 = To Double Precision Float(number=w715) -> (double precision float=w729:dbl)
                n437 = property on="R in Range" class="Bool (strict)"("Val(Sgnl)"=w724) -> ()  [unwired: 2 in, 2 out]
                n438 = Divide(x=w729, y=w732) -> (x/y=w731:dbl)
                n439 = property on="R deg/rev" class="DigNum (strict)"() -> ("Value"=w721:dbl)  [unwired: 2 in, 2 out]
                n440 = Multiply(x=w731, y=w721) -> (x*y=w730:dbl)
                n441 = Add(x=w730, y=w722) -> (x+y=w723:dbl)
                n442 = property on="R Position deg PV" class="DigNum (strict)"("Val(Sgnl)"=w723) -> ()  [unwired: 2 in, 2 out]
              }
              frame #1 {
                n443 = call "mdrive send command.vi"("error in (no error)"=w742, "Extra"="MV", "Command"=T10."Print Parameter", "VISA resource name"=w743) -> ("error out"=w745:errorcluster, "read buffer"=w748:string, "VISA resource name out"=w746:refnum<visa-resource-name>)  [unwired: 3 in]
                n444 = Decimal String To Number(string=w748, offset=0 ("offset (0)")) -> (number=w738:i32)  [unwired: 1 in, 1 out]
                n445 = Not Equal?(x=w748, y="") -> (x != y?=w741:bool)
                n446 = property on="R Ready" class="Bool (strict)"("Val(Sgnl)"=w741) -> ()  [unwired: 2 in, 2 out]
                n447 = Number To Boolean Array(number=w738) -> (Boolean array=w740:bool[])
                n448 = Index Array(array=w740, index=0) -> (element=w737:bool)
                n449 = property on="R in Motion" class="Bool (strict)"("Val(Sgnl)"=w737) -> ()  [unwired: 2 in, 2 out]
              }
              frame #2 {
                n450 = Wait (ms)(milliseconds to wait=u32 50) -> ()  [unwired: 1 out]
              }
              frame #3 {
                n451 = case shown="True" w758 {
                  tunnel: w759 -> [w765 w769]
                  tunnel: [w766 w769] -> w760
                  tunnel: [w767 w768] -> w761
                  tunnel: w762 -> [w764 w768]
                  frame #0 {
                    n452 = call "mdrive send command.vi"("error in (no error)"=w764, "Command"=T10."Stop", "VISA resource name"=w765) -> ("error out"=w767:errorcluster, "VISA resource name out"=w766:refnum<visa-resource-name>)  [unwired: 4 in, 1 out]
                  }
                  frame #1 {
                  }
                }
              }
              frame #4 {
                n453 = property on="R Backlash corr" class="Bool (strict)"() -> ("Value"=w770:bool)  [unwired: 2 in, 2 out]
                n454 = Implies(1:w776, 2:w770) -> (0:w775:bool)
                n455 = case shown="False" w775 {
                  tunnel: w774 -> [w784 w841]
                  tunnel: w773 -> [w783 w842]
                  tunnel: [w778 w841] -> w772
                  tunnel: [w782 w842] -> w771
                  frame #0 {
                    # "Backlash"
                    n456 = flat-sequence {
                      tunnel: [w797] -> w796
                      tunnel: [w801] -> w795
                      tunnel: [w800] -> w794
                      tunnel: w784 -> [w799]
                      tunnel: w783 -> [w798]
                      tunnel: w796 -> [w809]
                      tunnel: [w809] -> w793
                      tunnel: w795 -> [w808]
                      tunnel: w794 -> [w807]
                      tunnel: [w806] -> w792
                      tunnel: [w805] -> w791
                      tunnel: [w804] -> w781
                      tunnel: w793 -> [w823]
                      tunnel: w792 -> [w814]
                      tunnel: w791 -> [w822]
                      tunnel: [w814] -> w790
                      tunnel: [w822] -> w789
                      tunnel: [w813] -> w786
                      tunnel: [w821] -> w785
                      tunnel: w781 -> [w821]
                      tunnel: w790 -> [w826]
                      tunnel: w789 -> [w827]
                      tunnel: [w825] -> w788
                      tunnel: [w833] -> w787
                      tunnel: w786 -> [w833]
                      tunnel: w785 -> [w829]
                      tunnel: [w828] -> w779
                      tunnel: w788 -> [w836]
                      tunnel: w787 -> [w835]
                      tunnel: [w837] -> w780
                      tunnel: w779 -> [w837]
                      tunnel: [w836] -> w777
                      tunnel: [w840] -> w782
                      tunnel: w780 -> [w840]
                      tunnel: [w839] -> w778
                      tunnel: w777 -> [w839]
                      frame #0 {
                        n457 = property on="R Backlash steps/sec" class="DigNum (strict)"() -> ("Value"=w797:i32)  [unwired: 2 in, 2 out]
                        n458 = Number To Decimal String(number=w797) -> (decimal integer string=w802:string)  [unwired: 1 in]
                        n459 = call "mdrive send command.vi"("error in (no error)"=w799, "Extra"=w802, "Command"=T10."Max Velocity", "VISA resource name"=w798) -> ("error out"=w800:errorcluster, "VISA resource name out"=w801:refnum<visa-resource-name>)  [unwired: 3 in, 1 out]
                      }
                      frame #1 {
                        n460 = property on="R Backlash" class="DigNum (strict)"() -> ("Value"=w804:i32)  [unwired: 2 in, 2 out]
                        n461 = Number To Decimal String(number=w804) -> (decimal integer string=w810:string)  [unwired: 1 in]
                        n462 = call "mdrive send command.vi"("error in (no error)"=w807, "Extra"=w810, "Command"=T10."Move to Relative Position", "VISA resource name"=w808) -> ("error out"=w806:errorcluster, "VISA resource name out"=w805:refnum<visa-resource-name>)  [unwired: 3 in, 1 out]
                      }
                      frame #2 {
                        n463 = To Double Precision Float(number=w821) -> (double precision float=w819:dbl)
                        n464 = To Double Precision Float(number=w823) -> (double precision float=w824:dbl)
                        n465 = Absolute Value(x=w819) -> (abs(x)=w820:dbl)
                        n466 = Divide(x=w820, y=w824) -> (x/y=w817:dbl)
                        n467 = Multiply(x=1000.0, y=w817) -> (x*y=w815:dbl)
                        n468 = Add(x=w815, y=300.0) -> (x+y=w813:dbl)
                        n469 = To Unsigned Long Integer(number=w813) -> (unsigned 32bit integer=w812:u32)
                        n470 = Wait (ms)(milliseconds to wait=w812) -> ()  [unwired: 1 out]
                      }
                      frame #3 {
                        n471 = Negate(x=w829) -> (-x=w830:i32)
                        n472 = Number To Decimal String(number=w830) -> (decimal integer string=w831:string)  [unwired: 1 in]
                        n473 = call "mdrive send command.vi"("error in (no error)"=w826, "Extra"=w831, "Command"=T10."Move to Relative Position", "VISA resource name"=w827) -> ("error out"=w825:errorcluster, "VISA resource name out"=w828:refnum<visa-resource-name>)  [unwired: 3 in, 1 out]
                      }
                      frame #4 {
                        n474 = To Unsigned Long Integer(number=w835) -> (unsigned 32bit integer=w834:u32)
                        n475 = Wait (ms)(milliseconds to wait=w834) -> ()  [unwired: 1 out]
                      }
                      frame #5 {
                        n476 = property on="R Backlash corr" class="Bool (strict)"("Val(Sgnl)"=FALSE ("Value (Signaling)")) -> ()  [unwired: 2 in, 2 out]
                      }
                    }
                  }
                  frame #1 {
                  }
                }
              }
            }
            n477 = property on="Scan Go" class="Bool (strict)"() -> ("Value"=w594:bool)  [unwired: 2 in, 2 out]
            n478 = Equal?(x=w594, y=TRUE) -> (x = y?=w589:bool)
            n479 = property on="STATUS" class="Str"() -> ("Value"=w592:string)  [unwired: 2 in, 2 out]
            n480 = Equal?(x=w592, y="SCANNING MODE" ("STATUS")) -> (x = y?=w590:bool)
            n481 = Or(x=w590, y=w589) -> (x .or. y?=w588:bool)
            n482 = case shown="False" w588 {
              frame #0 {
                n483 = property on="Y in Motion" class="Bool (strict)"() -> ("Value"=w670:bool)  [unwired: 2 in, 2 out]
                n484 = property on="Z in Motion" class="Bool (strict)"() -> ("Value"=w673:bool)  [unwired: 2 in, 2 out]
                n485 = property on="X  in Motion" class="Bool (strict)"() -> ("Value"=w671:bool)  [unwired: 2 in, 2 out]
                n486 = property on="R in Motion" class="Bool (strict)"() -> ("Value"=w672:bool)  [unwired: 2 in, 2 out]
                n487 = Compound Arithmetic op=AND(w671, w670, w673, w672) -> (w668:bool)
                n488 = Equal?(x=w668, y=FALSE) -> (x = y?=w669:bool)
                n489 = case shown="True" w669 {
                  frame #0 {
                  }
                  frame #1 {
                    n490 = property on="X Step SP" class="DigNum (strict)"() -> ("Value"=w681:i32)  [unwired: 2 in, 2 out]
                    n491 = property on="X Step PV" class="DigNum (strict)"() -> ("Value"=w680:i32)  [unwired: 2 in, 2 out]
                    n492 = property on="Y Step SP" class="DigNum (strict)"() -> ("Value"=w679:i32)  [unwired: 2 in, 2 out]
                    n493 = property on="Y Step PV" class="DigNum (strict)"() -> ("Value"=w678:i32)  [unwired: 2 in, 2 out]
                    n494 = property on="Z Step SP" class="DigNum (strict)"() -> ("Value"=w677:i32)  [unwired: 2 in, 2 out]
                    n495 = property on="Z Step PV" class="DigNum (strict)"() -> ("Value"=w676:i32)  [unwired: 2 in, 2 out]
                    n496 = property on="R Step SP" class="DigNum (strict)"() -> ("Value"=w674:i32)  [unwired: 2 in, 2 out]
                    n497 = property on="R Step PV" class="DigNum (strict)"() -> ("Value"=w675:i32)  [unwired: 2 in, 2 out]
                    n498 = Equal?(x=w681, y=w680) -> (x = y?=w686:bool)
                    n499 = Equal?(x=w679, y=w678) -> (x = y?=w685:bool)
                    n500 = Equal?(x=w677, y=w676) -> (x = y?=w683:bool)
                    n501 = Equal?(x=w674, y=w675) -> (x = y?=w684:bool)
                    n502 = Compound Arithmetic op=AND(w686, w685, w683, w684) -> (w682:bool)
                    n503 = case shown="True" w682 {
                      frame #0 {
                      }
                      frame #1 {
                        n504 = property on="GO" class="Bool"("DisabledEnum"=T9."Enabled" ("Disabled")) -> ()  [unwired: 2 in, 2 out]
                        n505 = local write "STATUS"("SCANNING DONE" ("STATUS")) -> ()
                      }
                    }
                  }
                }
              }
              frame #1 {
                n506 = property on="X Scan Length SP steps" class="DigNum (strict)"() -> ("Value"=w700:i32)  [unwired: 2 in, 2 out]
                n507 = property on="Y Scan Length SP steps" class="DigNum (strict)"() -> ("Value"=w699:i32)  [unwired: 2 in, 2 out]
                n508 = property on="Z Scan Length SP steps" class="DigNum (strict)"() -> ("Value"=w698:i32)  [unwired: 2 in, 2 out]
                n509 = property on="R Scan Length SP steps" class="DigNum (strict)"() -> ("Value"=w697:i32)  [unwired: 2 in, 2 out]
                n510 = property on="X Step SP" class="DigNum (strict)"() -> ("Value"=w696:i32)  [unwired: 2 in, 2 out]
                n511 = property on="Y Step SP" class="DigNum (strict)"() -> ("Value"=w695:i32)  [unwired: 2 in, 2 out]
                n512 = property on="Z Step SP" class="DigNum (strict)"() -> ("Value"=w694:i32)  [unwired: 2 in, 2 out]
                n513 = property on="R Step SP" class="DigNum (strict)"() -> ("Value"=w693:i32)  [unwired: 2 in, 2 out]
                n514 = Add(x=w700, y=w696) -> (x+y=w709:i32)
                n515 = Add(x=w699, y=w695) -> (x+y=w708:i32)
                n516 = Add(x=w698, y=w694) -> (x+y=w707:i32)
                n517 = Add(x=w697, y=w693) -> (x+y=w706:i32)
                n518 = property on="X Step PV" class="DigNum (strict)"() -> ("Value"=w692:i32)  [unwired: 2 in, 2 out]
                n519 = property on="Y Step PV" class="DigNum (strict)"() -> ("Value"=w691:i32)  [unwired: 2 in, 2 out]
                n520 = property on="Z Step PV" class="DigNum (strict)"() -> ("Value"=w690:i32)  [unwired: 2 in, 2 out]
                n521 = property on="R Step PV" class="DigNum (strict)"() -> ("Value"=w689:i32)  [unwired: 2 in, 2 out]
                n522 = Equal?(x=w692, y=w709) -> (x = y?=w705:bool)
                n523 = Equal?(x=w691, y=w708) -> (x = y?=w704:bool)
                n524 = Equal?(x=w690, y=w707) -> (x = y?=w702:bool)
                n525 = Equal?(x=w689, y=w706) -> (x = y?=w703:bool)
                n526 = Compound Arithmetic op=AND(w705, w704, w702, w703) -> (w701:bool)
                n527 = case shown="True" w701 {
                  frame #0 {
                  }
                  frame #1 {
                    n528 = local write "Scan Go"(FALSE ("Scan Go")) -> ()
                    n529 = local write "STATUS"("DONE" ("STATUS")) -> ()
                    n530 = property on="Send scan parameter" class="Bool"("DisabledEnum"=T9."Enabled" ("Disabled")) -> ()  [unwired: 2 in, 2 out]
                    n531 = property on="Set Scan \nParameters" class="Bool"("DisabledEnum"=T9."Enabled" ("Disabled")) -> ()  [unwired: 2 in, 2 out]
                    n532 = property on="GO" class="Bool"("DisabledEnum"=T9."Enabled" ("Disabled")) -> ()  [unwired: 2 in, 2 out]
                  }
                }
              }
            }
          }
        }
        n533 = Divide(x=w530, y=6.283185307179586) -> (x/y=w531:dbl)
        n534 = case shown="False" w508 {
          frame #0 {
          }
          frame #1 {
            n535 = local write "STATUS"("") -> ()
          }
        }
        n536 = Multiply(x=360.0, y=w531) -> (x*y=w534:dbl)
        n537 = property on="atan Y/Z" class="DigNum (strict)"("Val(Sgnl)"=w534) -> ()  [unwired: 2 in, 2 out]
      }
      event #1 {
        n538 = event-data() -> ()  [unwired: 1 in, 5 out]
        n539 = property on="OK Button" class="Bool (strict)"() -> ("Value"=w1246:bool)  [unwired: 2 in, 2 out]
        n540 = property on="Z Step PV" class="DigNum (strict)"() -> ("Value"=w1251:i32)  [unwired: 2 in, 2 out]
        n541 = Greater?(x=w1251, y=15360000) -> (0:w1248:bool)
        n542 = Equal?(x=w1246, y=TRUE) -> (x = y?=w1249:bool)
        n543 = local write "STATUS"("VALVE CHANGED" ("STATUS")) -> ()
        n544 = And(x=w1249, y=w1248) -> (x .and. y?=w1247:bool)
        n545 = case shown="False" w1247 {
          frame #0 {
            n546 = property on="OK Button" class="Bool (strict)"() -> ("Value"=w1254:bool)  [unwired: 2 in, 2 out]
            n547 = property on="Z Step PV" class="DigNum (strict)"() -> ("Value"=w1259:i32)  [unwired: 2 in, 2 out]
            n548 = Greater?(x=w1259, y=15360000) -> (0:w1257:bool)
            n549 = Equal?(x=w1254, y=FALSE) -> (x = y?=w1256:bool)
            n550 = And(x=w1256, y=w1257) -> (x .and. y?=w1255:bool)
            n551 = case shown="True" w1255 {
              frame #0 {
              }
              frame #1 {
                n552 = One Button Dialog(message="YOU CAN'T CLOSE THE VALVE\nWHEN YOU ARE IN THE THIS\nPOSITION!!") -> (true=w1261:bool)  [unwired: 1 in]
                n553 = property on="OK Button" class="Bool (strict)"("Val(Sgnl)"=w1261) -> ()  [unwired: 2 in, 2 out]
              }
            }
          }
          frame #1 {
            n554 = flat-sequence {
              frame #0 {
                n555 = local read "OK Button"() -> (w1264:bool)
                n556 = call "DigitalIO_sub_V1_CNTL.vi"("OK Button"=w1264) -> ("Boolean"=w1263:bool)  [unwired: 2 in]
                n557 = property on="Valve \nopend/closed" class="Bool (strict)"("Val(Sgnl)"=w1263) -> ()  [unwired: 2 in, 2 out]
              }
              frame #1 {
                n558 = call "DigitalIO_sub_V1_MON.vi"() -> ("CL"=w1266:bool, "OP"=w1265:bool)  [unwired: 8 in]
                n559 = property on="OP" class="Bool (strict)"("Val(Sgnl)"=w1265) -> ()  [unwired: 2 in, 2 out]
                n560 = property on="CL" class="Bool (strict)"("Val(Sgnl)"=w1266) -> ()  [unwired: 2 in, 2 out]
              }
              frame #2 {
                n561 = Wait (ms)(milliseconds to wait=u32 100) -> ()  [unwired: 1 out]
              }
            }
          }
        }
      }
      event #2 {
        n562 = event-data() -> ()  [unwired: 1 in, 7 out]
        n563 = local write "STATUS"("MOVING" ("STATUS")) -> ()
        n564 = property on="X Position mm PV" class="DigNum (strict)"() -> ("Value"=w1288:dbl)  [unwired: 2 in, 2 out]
        n565 = property on="X Position SP mm" class="DigNum (strict)"() -> ("Value"=w1287:dbl)  [unwired: 2 in, 2 out]
        n566 = property on="Z Position mm PV" class="DigNum (strict)"() -> ("Value"=w1284:dbl)  [unwired: 2 in, 2 out]
        n567 = property on="Z Position SP mm" class="DigNum (strict)"() -> ("Value"=w1276:dbl)  [unwired: 2 in, 2 out]
        n568 = property on="Y Position mm PV" class="DigNum (strict)"() -> ("Value"=w1282:dbl)  [unwired: 2 in, 2 out]
        n569 = property on="Y Position SP mm" class="DigNum (strict)"() -> ("Value"=w1281:dbl)  [unwired: 2 in, 2 out]
        n570 = property on="R Position SP deg" class="DigNum (strict)"() -> ("Value"=w1279:dbl)  [unwired: 2 in, 2 out]
        n571 = property on="R Position deg PV" class="DigNum (strict)"() -> ("Value"=w1278:dbl)  [unwired: 2 in, 2 out]
        n572 = Not Equal?(x=w1288, y=w1287) -> (x != y?=w1286:bool)
        n573 = Not Equal?(x=w1284, y=w1276) -> (x != y?=w1285:bool)
        n574 = Not Equal?(x=w1282, y=w1281) -> (x != y?=w1283:bool)
        n575 = Not Equal?(x=w1279, y=w1278) -> (x != y?=w1280:bool)
        n576 = case shown="True" w1286 {
          tunnel: w1297 -> [w1521 w1525]
          tunnel: w1296 -> [w1520 w1524]
          tunnel: [w1521 w1523] -> w1275
          tunnel: [w1520 w1522] -> w1274
          frame #0 {
          }
          frame #1 {
            n577 = flat-sequence {
              tunnel: w1524 -> [w1552]
              tunnel: w1525 -> [w1553]
              tunnel: [w1553] -> w1539
              tunnel: [w1552] -> w1538
              tunnel: [w1541] -> w1537
              tunnel: [w1556] -> w1536
              tunnel: [w1555] -> w1535
              tunnel: [w1554] -> w1534
              tunnel: w1537 -> [w1554]
              tunnel: w1538 -> [w1555]
              tunnel: w1539 -> [w1556]
              tunnel: [w1572] -> w1533
              tunnel: [w1571] -> w1532
              tunnel: w1536 -> [w1570]
              tunnel: w1535 -> [w1569]
              tunnel: w1534 -> [w1568]
              tunnel: [w1568] -> w1531
              tunnel: w1533 -> [w1579]
              tunnel: [w1579] -> w1530
              tunnel: w1532 -> [w1578]
              tunnel: [w1578] -> w1529
              tunnel: [w1576] -> w1528
              tunnel: w1531 -> [w1576]
              tunnel: [w1584] -> w1527
              tunnel: [w1583] -> w1526
              tunnel: w1530 -> [w1582]
              tunnel: w1529 -> [w1581]
              tunnel: w1528 -> [w1580]
              tunnel: [w1588] -> w1522
              tunnel: [w1589] -> w1523
              tunnel: w1527 -> [w1589]
              tunnel: w1526 -> [w1588]
              frame #0 {
                n578 = property on="X steps/rev" class="DigNum (strict)"() -> ("Value"=w1551:u32)  [unwired: 2 in, 2 out]
                n579 = To Double Precision Float(number=w1551) -> (double precision float=w1546:dbl)
                n580 = property on="X offset mm" class="DigNum (strict)"() -> ("Value"=w1550:dbl)  [unwired: 2 in, 2 out]
                n581 = property on="X Position SP mm" class="DigNum (strict)"() -> ("Value"=w1549:dbl)  [unwired: 2 in, 2 out]
                n582 = Subtract(x=w1549, y=w1550) -> (x-y=w1543:dbl)
                n583 = property on="X mm/rev" class="DigNum (strict)"() -> ("Value"=w1540:dbl)  [unwired: 2 in, 2 out]
                n584 = Divide(x=w1543, y=w1540) -> (x/y=w1542:dbl)
                n585 = property on="X Step SP" class="DigNum (strict)"() -> ("Maximum"=w1548:dbl)  [unwired: 2 in, 2 out]
                n586 = property on="X Step SP" class="DigNum (strict)"() -> ("Minimum"=w1547:dbl)  [unwired: 2 in, 2 out]
                n587 = Multiply(x=w1542, y=w1546) -> (x*y=w1544:dbl)
                n588 = In Range and Coerce(upper limit=w1548, x=w1544, lower limit=w1547) -> (coerced(x)=w1545:dbl)  [unwired: 1 out]
                n589 = To Long Integer(number=w1545) -> (32bit integer=w1541:i32)
                n590 = property on="X Step SP" class="DigNum (strict)"("Val(Sgnl)"=w1541) -> ()  [unwired: 2 in, 2 out]
              }
              frame #1 {
                n591 = property on="X Step SP" class="DigNum (strict)"() -> ("Value"=w1565:i32)  [unwired: 2 in, 2 out]
                n592 = property on="X Step PV" class="DigNum (strict)"() -> ("Value"=w1564:i32)  [unwired: 2 in, 2 out]
                n593 = property on="X Backlash" class="DigNum (strict)"() -> ("Value"=w1557:i32)  [unwired: 2 in, 2 out]
                n594 = Subtract(x=w1565, y=w1564) -> (x-y=w1563:i32)
                n595 = Sign(1:w1557) -> (0:w1561:i32)
                n596 = Sign(1:w1563) -> (0:w1562:i32)
                n597 = Multiply(x=w1562, y=w1561) -> (x*y=w1560:i32)
                n598 = Equal?(x=w1560, y=1) -> (x = y?=w1558:bool)
                n599 = case shown="False" w1558 {
                  frame #0 {
                    n600 = property on="X Backlash corr" class="Bool (strict)"("Val(Sgnl)"=FALSE ("Value (Signaling)")) -> ()  [unwired: 2 in, 2 out]
                  }
                  frame #1 {
                    n601 = property on="X Backlash corr" class="Bool (strict)"("Val(Sgnl)"=TRUE ("Value (Signaling)")) -> ()  [unwired: 2 in, 2 out]
                  }
                }
              }
              frame #2 {
                # "Velocity Setting"
                n602 = property on="X Velocity SP step/sec" class="DigNum (strict)"() -> ("Value"=w1573:i32)  [unwired: 2 in, 2 out]
                n603 = Number To Decimal String(number=w1573) -> (decimal integer string=w1574:string)  [unwired: 1 in]
                n604 = call "mDrive Send Command.vi"("error in (no error)"=w1569, "Extra"=w1574, "Command"=T10."Max Velocity", "VISA resource name"=w1570) -> ("error out"=w1571:errorcluster, "VISA resource name out"=w1572:refnum<visa-resource-name>)  [unwired: 3 in, 1 out]
              }
              frame #3 {
                n605 = Wait (ms)(milliseconds to wait=u32 50) -> ()  [unwired: 1 out]
              }
              frame #4 {
                # "Move to Abs Position"
                n606 = Number To Decimal String(number=w1580) -> (decimal integer string=w1586:string)  [unwired: 1 in]
                n607 = call "mDrive Send Command.vi"("error in (no error)"=w1581, "Extra"=w1586, "Command"=T10."Move to Absolute Position", "VISA resource name"=w1582) -> ("error out"=w1583:errorcluster, "VISA resource name out"=w1584:refnum<visa-resource-name>)  [unwired: 3 in, 1 out]
              }
              frame #5 {
                n608 = Wait (ms)(milliseconds to wait=u32 50) -> ()  [unwired: 1 out]
              }
            }
          }
        }
        n609 = case shown="True" w1285 {
          tunnel: w1295 -> [w1438 w1445]
          tunnel: w1294 -> [w1439 w1444]
          tunnel: [w1439 w1443] -> w1273
          tunnel: [w1438 w1442] -> w1272
          frame #0 {
          }
          frame #1 {
            n610 = flat-sequence {
              tunnel: w1444 -> [w1467]
              tunnel: w1445 -> [w1468]
              tunnel: [w1468] -> w1441
              tunnel: [w1467] -> w1440
              tunnel: [w1483] -> w1459
              tunnel: [w1482] -> w1458
              tunnel: [w1470] -> w1457
              tunnel: w1441 -> [w1483]
              tunnel: w1440 -> [w1482]
              tunnel: [w1486] -> w1456
              tunnel: [w1485] -> w1455
              tunnel: [w1484] -> w1454
              tunnel: w1457 -> [w1484]
              tunnel: w1458 -> [w1485]
              tunnel: w1459 -> [w1486]
              tunnel: [w1502] -> w1453
              tunnel: [w1501] -> w1452
              tunnel: w1456 -> [w1500]
              tunnel: w1455 -> [w1499]
              tunnel: [w1498] -> w1451
              tunnel: w1454 -> [w1498]
              tunnel: w1453 -> [w1509]
              tunnel: [w1509] -> w1450
              tunnel: w1452 -> [w1508]
              tunnel: [w1508] -> w1449
              tunnel: w1451 -> [w1507]
              tunnel: [w1507] -> w1448
              tunnel: [w1514] -> w1447
              tunnel: [w1513] -> w1446
              tunnel: w1450 -> [w1512]
              tunnel: w1449 -> [w1511]
              tunnel: w1448 -> [w1510]
              tunnel: [w1518] -> w1442
              tunnel: [w1519] -> w1443
              tunnel: w1447 -> [w1519]
              tunnel: w1446 -> [w1518]
              frame #0 {
                n611 = property on="Z Position mm PV" class="DigNum (strict)"() -> ("Value"=w1460:dbl)  [unwired: 2 in, 2 out]
                n612 = property on="Z Position SP mm" class="DigNum (strict)"() -> ("Value"=w1462:dbl)  [unwired: 2 in, 2 out]
                n613 = Less?(x=w1460, y=60.0) -> (x < y?=w1464:bool)
                n614 = Greater?(x=w1462, y=60.0) -> (0:w1465:bool)
                n615 = And(x=w1464, y=w1465) -> (x .and. y?=w1466:bool)
                n616 = case shown="True" w1466 {
                  frame #0 {
                  }
                  frame #1 {
                    n617 = property on="Z Position SP mm" class="DigNum (strict)"("Val(Sgnl)"=60.0 ("Value (Signaling)")) -> ()  [unwired: 2 in, 2 out]
                  }
                }
              }
              frame #1 {
                n618 = property on="Z steps/rev" class="DigNum (strict)"() -> ("Value"=w1479:u32)  [unwired: 2 in, 2 out]
                n619 = To Double Precision Float(number=w1479) -> (double precision float=w1475:dbl)
                n620 = property on="Z offset mm" class="DigNum (strict)"() -> ("Value"=w1477:dbl)  [unwired: 2 in, 2 out]
                n621 = property on="Z Position SP mm" class="DigNum (strict)"() -> ("Value"=w1476:dbl)  [unwired: 2 in, 2 out]
                n622 = Subtract(x=w1476, y=w1477) -> (x-y=w1472:dbl)
                n623 = property on="Z mm/rev" class="DigNum (strict)"() -> ("Value"=w1478:dbl)  [unwired: 2 in, 2 out]
                n624 = Divide(x=w1472, y=w1478) -> (x/y=w1471:dbl)
                n625 = property on="Z Step SP" class="DigNum (strict)"() -> ("Maximum"=w1481:dbl)  [unwired: 2 in, 2 out]
                n626 = property on="Z Step SP" class="DigNum (strict)"() -> ("Minimum"=w1480:dbl)  [unwired: 2 in, 2 out]
                n627 = Multiply(x=w1471, y=w1475) -> (x*y=w1473:dbl)
                n628 = In Range and Coerce(upper limit=w1481, x=w1473, lower limit=w1480) -> (coerced(x)=w1474:dbl)  [unwired: 1 out]
                n629 = To Long Integer(number=w1474) -> (32bit integer=w1470:i32)
                n630 = property on="Z Step SP" class="DigNum (strict)"("Val(Sgnl)"=w1470) -> ()  [unwired: 2 in, 2 out]
              }
              frame #2 {
                n631 = property on="Z Step SP" class="DigNum (strict)"() -> ("Value"=w1495:i32)  [unwired: 2 in, 2 out]
                n632 = property on="Z Step PV" class="DigNum (strict)"() -> ("Value"=w1494:i32)  [unwired: 2 in, 2 out]
                n633 = property on="Z Backlash" class="DigNum (strict)"() -> ("Value"=w1487:i32)  [unwired: 2 in, 2 out]
                n634 = Subtract(x=w1495, y=w1494) -> (x-y=w1493:i32)
                n635 = Sign(1:w1487) -> (0:w1491:i32)
                n636 = Sign(1:w1493) -> (0:w1492:i32)
                n637 = Multiply(x=w1492, y=w1491) -> (x*y=w1490:i32)
                n638 = Equal?(x=w1490, y=1) -> (x = y?=w1488:bool)
                n639 = case shown="False" w1488 {
                  frame #0 {
                    n640 = property on="Z Backlash corr" class="Bool (strict)"("Val(Sgnl)"=FALSE ("Value (Signaling)")) -> ()  [unwired: 2 in, 2 out]
                  }
                  frame #1 {
                    n641 = property on="Z Backlash corr" class="Bool (strict)"("Val(Sgnl)"=TRUE ("Value (Signaling)")) -> ()  [unwired: 2 in, 2 out]
                  }
                }
              }
              frame #3 {
                # "Velocity Setting"
                n642 = property on="Z Velocity SP step/sec" class="DigNum (strict)"() -> ("Value"=w1503:i32)  [unwired: 2 in, 2 out]
                n643 = Number To Decimal String(number=w1503) -> (decimal integer string=w1504:string)  [unwired: 1 in]
                n644 = call "mdrive send command.vi"("error in (no error)"=w1500, "Extra"=w1504, "Command"=T10."Max Velocity", "VISA resource name"=w1499) -> ("error out"=w1501:errorcluster, "VISA resource name out"=w1502:refnum<visa-resource-name>)  [unwired: 3 in, 1 out]
              }
              frame #4 {
                n645 = Wait (ms)(milliseconds to wait=u32 50) -> ()  [unwired: 1 out]
              }
              frame #5 {
                # "Move to Abs Position"
                n646 = Number To Decimal String(number=w1510) -> (decimal integer string=w1516:string)  [unwired: 1 in]
                n647 = call "mdrive send command.vi"("error in (no error)"=w1511, "Extra"=w1516, "Command"=T10."Move to Absolute Position", "VISA resource name"=w1512) -> ("error out"=w1513:errorcluster, "VISA resource name out"=w1514:refnum<visa-resource-name>)  [unwired: 3 in, 1 out]
              }
              frame #6 {
                n648 = Wait (ms)(milliseconds to wait=u32 50) -> ()  [unwired: 1 out]
              }
            }
          }
        }
        n649 = case shown="True" w1283 {
          tunnel: w1293 -> [w1368 w1373]
          tunnel: w1292 -> [w1369 w1372]
          tunnel: [w1369 w1371] -> w1271
          tunnel: [w1368 w1370] -> w1270
          frame #0 {
          }
          frame #1 {
            n650 = flat-sequence {
              tunnel: [w1401] -> w1387
              tunnel: [w1400] -> w1386
              tunnel: [w1388] -> w1385
              tunnel: w1372 -> [w1400]
              tunnel: w1373 -> [w1401]
              tunnel: [w1404] -> w1384
              tunnel: [w1403] -> w1383
              tunnel: [w1402] -> w1382
              tunnel: w1385 -> [w1402]
              tunnel: w1386 -> [w1403]
              tunnel: w1387 -> [w1404]
              tunnel: [w1420] -> w1381
              tunnel: [w1419] -> w1380
              tunnel: w1384 -> [w1418]
              tunnel: w1383 -> [w1417]
              tunnel: [w1416] -> w1379
              tunnel: w1382 -> [w1416]
              tunnel: w1381 -> [w1427]
              tunnel: [w1427] -> w1378
              tunnel: w1380 -> [w1426]
              tunnel: [w1426] -> w1377
              tunnel: [w1424] -> w1376
              tunnel: w1379 -> [w1424]
              tunnel: [w1432] -> w1375
              tunnel: [w1431] -> w1374
              tunnel: w1378 -> [w1430]
              tunnel: w1377 -> [w1429]
              tunnel: w1376 -> [w1428]
              tunnel: [w1435] -> w1370
              tunnel: [w1437] -> w1371
              tunnel: w1375 -> [w1437]
              tunnel: w1374 -> [w1435]
              frame #0 {
                n651 = property on="Y steps/rev" class="DigNum (strict)"() -> ("Value"=w1397:u32)  [unwired: 2 in, 2 out]
                n652 = To Double Precision Float(number=w1397) -> (double precision float=w1393:dbl)
                n653 = property on="Y offset mm" class="DigNum (strict)"() -> ("Value"=w1395:dbl)  [unwired: 2 in, 2 out]
                n654 = property on="Y Position SP mm" class="DigNum (strict)"() -> ("Value"=w1394:dbl)  [unwired: 2 in, 2 out]
                n655 = Subtract(x=w1394, y=w1395) -> (x-y=w1390:dbl)
                n656 = property on="Y mm/rev" class="DigNum (strict)"() -> ("Value"=w1396:dbl)  [unwired: 2 in, 2 out]
                n657 = Divide(x=w1390, y=w1396) -> (x/y=w1389:dbl)
                n658 = property on="Y Step SP" class="DigNum (strict)"() -> ("Maximum"=w1398:dbl)  [unwired: 2 in, 2 out]
                n659 = property on="Y Step SP" class="DigNum (strict)"() -> ("Minimum"=w1399:dbl)  [unwired: 2 in, 2 out]
                n660 = Multiply(x=w1389, y=w1393) -> (x*y=w1391:dbl)
                n661 = In Range and Coerce(upper limit=w1398, x=w1391, lower limit=w1399) -> (coerced(x)=w1392:dbl)  [unwired: 1 out]
                n662 = To Long Integer(number=w1392) -> (32bit integer=w1388:i32)
                n663 = property on="Y Step SP" class="DigNum (strict)"("Val(Sgnl)"=w1388) -> ()  [unwired: 2 in, 2 out]
              }
              frame #1 {
                n664 = property on="Y Step SP" class="DigNum (strict)"() -> ("Value"=w1413:i32)  [unwired: 2 in, 2 out]
                n665 = property on="Y Step PV" class="DigNum (strict)"() -> ("Value"=w1412:i32)  [unwired: 2 in, 2 out]
                n666 = property on="Y Backlash" class="DigNum (strict)"() -> ("Value"=w1405:i32)  [unwired: 2 in, 2 out]
                n667 = Subtract(x=w1413, y=w1412) -> (x-y=w1411:i32)
                n668 = Sign(1:w1405) -> (0:w1409:i32)
                n669 = Sign(1:w1411) -> (0:w1410:i32)
                n670 = Multiply(x=w1410, y=w1409) -> (x*y=w1408:i32)
                n671 = Equal?(x=w1408, y=1) -> (x = y?=w1406:bool)
                n672 = case shown="False" w1406 {
                  frame #0 {
                    n673 = property on="Y Backlash corr" class="Bool (strict)"("Val(Sgnl)"=FALSE ("Value (Signaling)")) -> ()  [unwired: 2 in, 2 out]
                  }
                  frame #1 {
                    n674 = property on="Y Backlash corr" class="Bool (strict)"("Val(Sgnl)"=TRUE ("Value (Signaling)")) -> ()  [unwired: 2 in, 2 out]
                  }
                }
              }
              frame #2 {
                # "Velocity Setting"
                n675 = property on="Y Velocity SP step/sec" class="DigNum (strict)"() -> ("Value"=w1421:i32)  [unwired: 2 in, 2 out]
                n676 = Number To Decimal String(number=w1421) -> (decimal integer string=w1422:string)  [unwired: 1 in]
                n677 = call "mdrive send command.vi"("error in (no error)"=w1418, "Extra"=w1422, "Command"=T10."Max Velocity", "VISA resource name"=w1417) -> ("error out"=w1419:errorcluster, "VISA resource name out"=w1420:refnum<visa-resource-name>)  [unwired: 3 in, 1 out]
              }
              frame #3 {
                n678 = Wait (ms)(milliseconds to wait=u32 50) -> ()  [unwired: 1 out]
              }
              frame #4 {
                # "Move to Abs Position"
                n679 = Number To Decimal String(number=w1428) -> (decimal integer string=w1434:string)  [unwired: 1 in]
                n680 = call "mdrive send command.vi"("error in (no error)"=w1429, "Extra"=w1434, "Command"=T10."Move to Absolute Position", "VISA resource name"=w1430) -> ("error out"=w1431:errorcluster, "VISA resource name out"=w1432:refnum<visa-resource-name>)  [unwired: 3 in, 1 out]
              }
              frame #5 {
                n681 = Wait (ms)(milliseconds to wait=u32 25) -> ()  [unwired: 1 out]
              }
            }
          }
        }
        n682 = case shown="True" w1280 {
          tunnel: w1291 -> [w1298 w1303]
          tunnel: w1290 -> [w1299 w1302]
          tunnel: [w1299 w1301] -> w1269
          tunnel: [w1298 w1300] -> w1268
          frame #0 {
          }
          frame #1 {
            n683 = flat-sequence {
              tunnel: w1302 -> [w1330]
              tunnel: w1303 -> [w1331]
              tunnel: [w1331] -> w1317
              tunnel: [w1330] -> w1316
              tunnel: [w1318] -> w1315
              tunnel: [w1334] -> w1314
              tunnel: [w1333] -> w1313
              tunnel: [w1332] -> w1312
              tunnel: w1315 -> [w1332]
              tunnel: w1316 -> [w1333]
              tunnel: w1317 -> [w1334]
              tunnel: [w1350] -> w1311
              tunnel: [w1349] -> w1310
              tunnel: w1314 -> [w1348]
              tunnel: w1313 -> [w1347]
              tunnel: [w1346] -> w1309
              tunnel: w1312 -> [w1346]
              tunnel: w1311 -> [w1357]
              tunnel: [w1357] -> w1308
              tunnel: w1310 -> [w1356]
              tunnel: [w1356] -> w1307
              tunnel: w1309 -> [w1355]
              tunnel: [w1355] -> w1306
              tunnel: [w1362] -> w1305
              tunnel: [w1361] -> w1304
              tunnel: w1308 -> [w1360]
              tunnel: w1307 -> [w1359]
              tunnel: w1306 -> [w1358]
              tunnel: [w1367] -> w1301
              tunnel: w1305 -> [w1367]
              tunnel: w1304 -> [w1366]
              tunnel: [w1366] -> w1300
              frame #0 {
                n684 = property on="R steps/rev" class="DigNum (strict)"() -> ("Value"=w1326:u32)  [unwired: 2 in, 2 out]
                n685 = To Double Precision Float(number=w1326) -> (double precision float=w1323:dbl)
                n686 = property on="R offset deg" class="DigNum (strict)"() -> ("Value"=w1327:dbl)  [unwired: 2 in, 2 out]
                n687 = property on="R Position SP deg" class="DigNum (strict)"() -> ("Value"=w1328:dbl)  [unwired: 2 in, 2 out]
                n688 = Subtract(x=w1328, y=w1327) -> (x-y=w1320:dbl)
                n689 = property on="R deg/rev" class="DigNum (strict)"() -> ("Value"=w1329:dbl)  [unwired: 2 in, 2 out]
                n690 = Divide(x=w1320, y=w1329) -> (x/y=w1319:dbl)
                n691 = property on="R Step SP" class="DigNum (strict)"() -> ("Maximum"=w1324:dbl)  [unwired: 2 in, 2 out]
                n692 = Multiply(x=w1319, y=w1323) -> (x*y=w1321:dbl)
                n693 = property on="R Step SP" class="DigNum (strict)"() -> ("Minimum"=w1325:dbl)  [unwired: 2 in, 2 out]
                n694 = In Range and Coerce(upper limit=w1324, x=w1321, lower limit=w1325) -> (coerced(x)=w1322:dbl)  [unwired: 1 out]
                n695 = To Long Integer(number=w1322) -> (32bit integer=w1318:i32)
                n696 = property on="R Step SP" class="DigNum (strict)"("Val(Sgnl)"=w1318) -> ()  [unwired: 2 in, 2 out]
              }
              frame #1 {
                n697 = property on="R Step SP" class="DigNum (strict)"() -> ("Value"=w1343:i32)  [unwired: 2 in, 2 out]
                n698 = property on="R Step PV" class="DigNum (strict)"() -> ("Value"=w1342:i32)  [unwired: 2 in, 2 out]
                n699 = property on="R Backlash" class="DigNum (strict)"() -> ("Value"=w1335:i32)  [unwired: 2 in, 2 out]
                n700 = Subtract(x=w1343, y=w1342) -> (x-y=w1341:i32)
                n701 = Sign(1:w1335) -> (0:w1339:i32)
                n702 = Sign(1:w1341) -> (0:w1340:i32)
                n703 = Multiply(x=w1340, y=w1339) -> (x*y=w1338:i32)
                n704 = Equal?(x=w1338, y=1) -> (x = y?=w1336:bool)
                n705 = case shown="False" w1336 {
                  frame #0 {
                    n706 = property on="R Backlash corr" class="Bool (strict)"("Val(Sgnl)"=FALSE ("Value (Signaling)")) -> ()  [unwired: 2 in, 2 out]
                  }
                  frame #1 {
                    n707 = property on="R Backlash corr" class="Bool (strict)"("Val(Sgnl)"=TRUE ("Value (Signaling)")) -> ()  [unwired: 2 in, 2 out]
                  }
                }
              }
              frame #2 {
                # "Velocity Setting"
                n708 = property on="R Velocity SP step/sec" class="DigNum (strict)"() -> ("Value"=w1351:i32)  [unwired: 2 in, 2 out]
                n709 = Number To Decimal String(number=w1351) -> (decimal integer string=w1352:string)  [unwired: 1 in]
                n710 = call "mdrive send command.vi"("error in (no error)"=w1348, "Extra"=w1352, "Command"=T10."Max Velocity", "VISA resource name"=w1347) -> ("error out"=w1349:errorcluster, "VISA resource name out"=w1350:refnum<visa-resource-name>)  [unwired: 3 in, 1 out]
              }
              frame #3 {
                n711 = Wait (ms)(milliseconds to wait=u32 50) -> ()  [unwired: 1 out]
              }
              frame #4 {
                # "Move to Abs Position"
                n712 = Number To Decimal String(number=w1358) -> (decimal integer string=w1364:string)  [unwired: 1 in]
                n713 = call "mdrive send command.vi"("error in (no error)"=w1359, "Extra"=w1364, "Command"=T10."Move to Absolute Position", "VISA resource name"=w1360) -> ("error out"=w1361:errorcluster, "VISA resource name out"=w1362:refnum<visa-resource-name>)  [unwired: 3 in, 1 out]
              }
              frame #5 {
                n714 = Wait (ms)(milliseconds to wait=u32 25) -> ()  [unwired: 1 out]
              }
            }
          }
        }
        n715 = property on="GO" class="Bool"("DisabledEnum"=T9."Disabled and Grayed Out" ("Disabled")) -> ()  [unwired: 2 in, 2 out]
      }
      event #3 {
        n716 = event-data() -> ()  [unwired: 1 in, 7 out]
        n717 = flat-sequence {
          tunnel: w1611 -> [w1618]
          tunnel: [w1617] -> w1603
          tunnel: w1602 -> [w1616]
          tunnel: [w1615] -> w1600
          tunnel: [w1622] -> w1604
          tunnel: w1603 -> [w1622]
          tunnel: [w1621] -> w1601
          tunnel: w1600 -> [w1621]
          tunnel: w1604 -> [w1639]
          tunnel: w1601 -> [w1636]
          tunnel: [w1635] -> _
          tunnel: [w1634] -> _
          frame #0 {
            n718 = call "mDrive Send Command.vi"("error in (no error)"=w1618, "Command"=T10."Stop", "VISA resource name"=w1616) -> ("error out"=w1617:errorcluster, "VISA resource name out"=w1615:refnum<visa-resource-name>)  [unwired: 4 in, 1 out]
          }
          frame #1 {
            n719 = Wait (ms)(milliseconds to wait=u32 50) -> ()  [unwired: 1 out]
          }
          frame #2 {
            n720 = property on="R steps/rev" class="DigNum (strict)"() -> ("Value"=w1627:u32)  [unwired: 2 in, 2 out]
            n721 = property on="R offset deg" class="DigNum (strict)"() -> ("Value"=w1624:dbl)  [unwired: 2 in, 2 out]
            n722 = To Double Precision Float(number=w1627) -> (double precision float=w1630:dbl)
            n723 = call "mDrive Send Command.vi"("error in (no error)"=w1639, "Extra"="P", "Command"=T10."Print Parameter", "VISA resource name"=w1636) -> ("error out"=w1634:errorcluster, "read buffer"=w1629:string, "VISA resource name out"=w1635:refnum<visa-resource-name>)  [unwired: 3 in]
            n724 = Decimal String To Number(string=w1629, offset=0) -> (number=w1626:i32)  [unwired: 1 in, 1 out]
            n725 = property on="R Step PV" class="DigNum (strict)"("Val(Sgnl)"=w1626) -> ()  [unwired: 2 in, 2 out]
            n726 = To Double Precision Float(number=w1626) -> (double precision float=w1631:dbl)
            n727 = Divide(x=w1631, y=w1630) -> (x/y=w1633:dbl)
            n728 = property on="R deg/rev" class="DigNum (strict)"() -> ("Value"=w1625:dbl)  [unwired: 2 in, 2 out]
            n729 = Multiply(x=w1633, y=w1625) -> (x*y=w1632:dbl)
            n730 = Add(x=w1632, y=w1624) -> (x+y=w1623:dbl)
            n731 = property on="R Position deg PV" class="DigNum (strict)"("Val(Sgnl)"=w1623) -> ()  [unwired: 2 in, 2 out]
          }
        }
        n732 = flat-sequence {
          tunnel: w1614 -> [w1643]
          tunnel: [w1642] -> w1609
          tunnel: w1593 -> [w1641]
          tunnel: [w1640] -> w1591
          tunnel: [w1647] -> w1610
          tunnel: w1609 -> [w1647]
          tunnel: [w1646] -> w1592
          tunnel: w1591 -> [w1646]
          tunnel: w1610 -> [w1664]
          tunnel: w1592 -> [w1661]
          tunnel: [w1660] -> _
          tunnel: [w1659] -> _
          frame #0 {
            n733 = call "mDrive Send Command.vi"("error in (no error)"=w1643, "Command"=T10."Stop", "VISA resource name"=w1641) -> ("error out"=w1642:errorcluster, "VISA resource name out"=w1640:refnum<visa-resource-name>)  [unwired: 4 in, 1 out]
          }
          frame #1 {
            n734 = Wait (ms)(milliseconds to wait=u32 50) -> ()  [unwired: 1 out]
          }
          frame #2 {
            n735 = property on="X steps/rev" class="DigNum (strict)"() -> ("Value"=w1650:u32)  [unwired: 2 in, 2 out]
            n736 = property on="X offset mm" class="DigNum (strict)"() -> ("Value"=w1648:dbl)  [unwired: 2 in, 2 out]
            n737 = To Double Precision Float(number=w1650) -> (double precision float=w1655:dbl)
            n738 = call "mDrive Send Command.vi"("error in (no error)"=w1664, "Extra"="P", "Command"=T10."Print Parameter", "VISA resource name"=w1661) -> ("error out"=w1659:errorcluster, "read buffer"=w1654:string, "VISA resource name out"=w1660:refnum<visa-resource-name>)  [unwired: 3 in]
            n739 = Decimal String To Number(string=w1654, offset=0) -> (number=w1652:i32)  [unwired: 1 in, 1 out]
            n740 = property on="X Step PV" class="DigNum (strict)"("Val(Sgnl)"=w1652) -> ()  [unwired: 2 in, 2 out]
            n741 = To Double Precision Float(number=w1652) -> (double precision float=w1656:dbl)
            n742 = Divide(x=w1656, y=w1655) -> (x/y=w1658:dbl)
            n743 = property on="X mm/rev" class="DigNum (strict)"() -> ("Value"=w1649:dbl)  [unwired: 2 in, 2 out]
            n744 = Multiply(x=w1658, y=w1649) -> (x*y=w1657:dbl)
            n745 = Add(x=w1657, y=w1648) -> (x+y=w1651:dbl)
            n746 = property on="X Position mm PV" class="DigNum (strict)"("Val(Sgnl)"=w1651) -> ()  [unwired: 2 in, 2 out]
          }
        }
        n747 = flat-sequence {
          tunnel: w1613 -> [w1668]
          tunnel: [w1667] -> w1607
          tunnel: w1596 -> [w1666]
          tunnel: [w1665] -> w1594
          tunnel: [w1672] -> w1608
          tunnel: w1607 -> [w1672]
          tunnel: [w1671] -> w1595
          tunnel: w1594 -> [w1671]
          tunnel: w1608 -> [w1689]
          tunnel: w1595 -> [w1686]
          tunnel: [w1685] -> _
          tunnel: [w1684] -> _
          frame #0 {
            n748 = call "mDrive Send Command.vi"("error in (no error)"=w1668, "Command"=T10."Stop", "VISA resource name"=w1666) -> ("error out"=w1667:errorcluster, "VISA resource name out"=w1665:refnum<visa-resource-name>)  [unwired: 4 in, 1 out]
          }
          frame #1 {
            n749 = Wait (ms)(milliseconds to wait=u32 50) -> ()  [unwired: 1 out]
          }
          frame #2 {
            n750 = property on="Z steps/rev" class="DigNum (strict)"() -> ("Value"=w1675:u32)  [unwired: 2 in, 2 out]
            n751 = property on="Z offset mm" class="DigNum (strict)"() -> ("Value"=w1673:dbl)  [unwired: 2 in, 2 out]
            n752 = To Double Precision Float(number=w1675) -> (double precision float=w1680:dbl)
            n753 = call "mDrive Send Command.vi"("error in (no error)"=w1689, "Extra"="P", "Command"=T10."Print Parameter", "VISA resource name"=w1686) -> ("error out"=w1684:errorcluster, "read buffer"=w1679:string, "VISA resource name out"=w1685:refnum<visa-resource-name>)  [unwired: 3 in]
            n754 = Decimal String To Number(string=w1679, offset=0) -> (number=w1677:i32)  [unwired: 1 in, 1 out]
            n755 = property on="Z Step PV" class="DigNum (strict)"("Val(Sgnl)"=w1677) -> ()  [unwired: 2 in, 2 out]
            n756 = To Double Precision Float(number=w1677) -> (double precision float=w1681:dbl)
            n757 = Divide(x=w1681, y=w1680) -> (x/y=w1683:dbl)
            n758 = property on="Z mm/rev" class="DigNum (strict)"() -> ("Value"=w1674:dbl)  [unwired: 2 in, 2 out]
            n759 = Multiply(x=w1683, y=w1674) -> (x*y=w1682:dbl)
            n760 = Add(x=w1682, y=w1673) -> (x+y=w1676:dbl)
            n761 = property on="Z Position mm PV" class="DigNum (strict)"("Val(Sgnl)"=w1676) -> ()  [unwired: 2 in, 2 out]
          }
        }
        n762 = flat-sequence {
          tunnel: w1612 -> [w1693]
          tunnel: [w1692] -> w1605
          tunnel: w1599 -> [w1691]
          tunnel: [w1690] -> w1597
          tunnel: [w1697] -> w1606
          tunnel: w1605 -> [w1697]
          tunnel: [w1696] -> w1598
          tunnel: w1597 -> [w1696]
          tunnel: w1606 -> [w1714]
          tunnel: w1598 -> [w1711]
          tunnel: [w1710] -> _
          tunnel: [w1709] -> _
          frame #0 {
            n763 = call "mDrive Send Command.vi"("error in (no error)"=w1693, "Command"=T10."Stop", "VISA resource name"=w1691) -> ("error out"=w1692:errorcluster, "VISA resource name out"=w1690:refnum<visa-resource-name>)  [unwired: 4 in, 1 out]
          }
          frame #1 {
            n764 = Wait (ms)(milliseconds to wait=u32 50) -> ()  [unwired: 1 out]
          }
          frame #2 {
            n765 = property on="Y steps/rev" class="DigNum (strict)"() -> ("Value"=w1700:u32)  [unwired: 2 in, 2 out]
            n766 = property on="Y offset mm" class="DigNum (strict)"() -> ("Value"=w1698:dbl)  [unwired: 2 in, 2 out]
            n767 = To Double Precision Float(number=w1700) -> (double precision float=w1705:dbl)
            n768 = call "mDrive Send Command.vi"("error in (no error)"=w1714, "Extra"="P", "Command"=T10."Print Parameter", "VISA resource name"=w1711) -> ("error out"=w1709:errorcluster, "read buffer"=w1704:string, "VISA resource name out"=w1710:refnum<visa-resource-name>)  [unwired: 3 in]
            n769 = Decimal String To Number(string=w1704, offset=0) -> (number=w1701:i32)  [unwired: 1 in, 1 out]
            n770 = property on="Y Step PV" class="DigNum (strict)"("Val(Sgnl)"=w1701) -> ()  [unwired: 2 in, 2 out]
            n771 = To Double Precision Float(number=w1701) -> (double precision float=w1706:dbl)
            n772 = Divide(x=w1706, y=w1705) -> (x/y=w1708:dbl)
            n773 = property on="Y mm/rev" class="DigNum (strict)"() -> ("Value"=w1699:dbl)  [unwired: 2 in, 2 out]
            n774 = Multiply(x=w1708, y=w1699) -> (x*y=w1707:dbl)
            n775 = Add(x=w1707, y=w1698) -> (x+y=w1702:dbl)
            n776 = property on="Y Position mm PV" class="DigNum (strict)"("Val(Sgnl)"=w1702) -> ()  [unwired: 2 in, 2 out]
          }
        }
        n777 = property on="GO" class="Bool"("DisabledEnum"=T9."Enabled" ("Disabled")) -> ()  [unwired: 2 in, 2 out]
      }
      event #4 {
        n778 = event-data() -> ()  [unwired: 1 in, 5 out]
        n779 = property on="Y steps/rev" class="DigNum (strict)"() -> ("Value"=w1745:u32)  [unwired: 2 in, 2 out]
        n780 = property on="X steps/rev" class="DigNum (strict)"() -> ("Value"=w1736:u32)  [unwired: 2 in, 2 out]
        n781 = property on="Z steps/rev" class="DigNum (strict)"() -> ("Value"=w1727:u32)  [unwired: 2 in, 2 out]
        n782 = property on="R steps/rev" class="DigNum (strict)"() -> ("Value"=w1718:u32)  [unwired: 2 in, 2 out]
        n783 = property on="R offset deg" class="DigNum (strict)"() -> ("Value"=w1716:dbl)  [unwired: 2 in, 2 out]
        n784 = property on="Y offset mm" class="DigNum (strict)"() -> ("Value"=w1743:dbl)  [unwired: 2 in, 2 out]
        n785 = property on="X offset mm" class="DigNum (strict)"() -> ("Value"=w1734:dbl)  [unwired: 2 in, 2 out]
        n786 = property on="Z offset mm" class="DigNum (strict)"() -> ("Value"=w1725:dbl)  [unwired: 2 in, 2 out]
        n787 = To Double Precision Float(number=w1718) -> (double precision float=w1721:dbl)
        n788 = To Double Precision Float(number=w1736) -> (double precision float=w1739:dbl)
        n789 = To Double Precision Float(number=w1727) -> (double precision float=w1730:dbl)
        n790 = property on="Reset Y Position mm" class="DigNum (strict)"() -> ("Value"=w1751:dbl)  [unwired: 2 in, 2 out]
        n791 = property on="Reset X Position mm" class="DigNum (strict)"() -> ("Value"=w1742:dbl)  [unwired: 2 in, 2 out]
        n792 = property on="Reset Z Position mm" class="DigNum (strict)"() -> ("Value"=w1733:dbl)  [unwired: 2 in, 2 out]
        n793 = property on="Reset R Position deg" class="DigNum (strict)"() -> ("Value"=w1724:dbl)  [unwired: 2 in, 2 out]
        n794 = local write "STATUS"("RESSETTING" ("STATUS")) -> ()
        n795 = Subtract(x=w1751, y=w1743) -> (x-y=w1750:dbl)
        n796 = Subtract(x=w1724, y=w1716) -> (x-y=w1723:dbl)
        n797 = Subtract(x=w1742, y=w1734) -> (x-y=w1741:dbl)
        n798 = Subtract(x=w1733, y=w1725) -> (x-y=w1732:dbl)
        n799 = property on="Y mm/rev" class="DigNum (strict)"() -> ("Value"=w1744:dbl)  [unwired: 2 in, 2 out]
        n800 = property on="X mm/rev" class="DigNum (strict)"() -> ("Value"=w1735:dbl)  [unwired: 2 in, 2 out]
        n801 = property on="Z mm/rev" class="DigNum (strict)"() -> ("Value"=w1726:dbl)  [unwired: 2 in, 2 out]
        n802 = property on="R deg/rev" class="DigNum (strict)"() -> ("Value"=w1717:dbl)  [unwired: 2 in, 2 out]
        n803 = Divide(x=w1723, y=w1717) -> (x/y=w1722:dbl)
        n804 = Divide(x=w1741, y=w1735) -> (x/y=w1740:dbl)
        n805 = Divide(x=w1732, y=w1726) -> (x/y=w1731:dbl)
        n806 = Divide(x=w1750, y=w1744) -> (x/y=w1749:dbl)
        n807 = To Double Precision Float(number=w1745) -> (double precision float=w1748:dbl)
        n808 = Multiply(x=w1749, y=w1748) -> (x*y=w1747:dbl)
        n809 = Multiply(x=w1722, y=w1721) -> (x*y=w1720:dbl)
        n810 = Multiply(x=w1740, y=w1739) -> (x*y=w1738:dbl)
        n811 = Multiply(x=w1731, y=w1730) -> (x*y=w1729:dbl)
        n812 = To Long Integer(number=w1747) -> (32bit integer=w1746:i32)
        n813 = To Long Integer(number=w1720) -> (32bit integer=w1719:i32)
        n814 = To Long Integer(number=w1738) -> (32bit integer=w1737:i32)
        n815 = To Long Integer(number=w1729) -> (32bit integer=w1728:i32)
        n816 = property on="Reset Y Motor Steps" class="DigNum (strict)"("Val(Sgnl)"=w1746) -> ()  [unwired: 2 in, 2 out]
        n817 = property on="Reset R Motor Steps" class="DigNum (strict)"("Val(Sgnl)"=w1719) -> ()  [unwired: 2 in, 2 out]
        n818 = property on="Reset X Motor Steps" class="DigNum (strict)"("Val(Sgnl)"=w1737) -> ()  [unwired: 2 in, 2 out]
        n819 = property on="Reset Z Motor Steps" class="DigNum (strict)"("Val(Sgnl)"=w1728) -> ()  [unwired: 2 in, 2 out]
      }
      event #5 {
        n820 = event-data() -> ()  [unwired: 1 in, 5 out]
        n821 = property on="X Step SP" class="DigNum (strict)"() -> ("Value"=w1776:i32)  [unwired: 2 in, 2 out]
        n822 = property on="Z Step SP" class="DigNum (strict)"() -> ("Value"=w1768:i32)  [unwired: 2 in, 2 out]
        n823 = property on="Y Step SP" class="DigNum (strict)"() -> ("Value"=w1784:i32)  [unwired: 2 in, 2 out]
        n824 = property on="X steps/rev" class="DigNum (strict)"() -> ("Value"=w1801:u32)  [unwired: 2 in, 2 out]
        n825 = property on="X steps/rev" class="DigNum (strict)"() -> ("Value"=w1774:u32)  [unwired: 2 in, 2 out]
        n826 = property on="R Step SP" class="DigNum (strict)"() -> ("Value"=w1760:i32)  [unwired: 2 in, 2 out]
        n827 = property on="Z steps/rev" class="DigNum (strict)"() -> ("Value"=w1795:u32)  [unwired: 2 in, 2 out]
        n828 = property on="Z steps/rev" class="DigNum (strict)"() -> ("Value"=w1766:u32)  [unwired: 2 in, 2 out]
        n829 = property on="Y steps/rev" class="DigNum (strict)"() -> ("Value"=w1807:u32)  [unwired: 2 in, 2 out]
        n830 = property on="Y steps/rev" class="DigNum (strict)"() -> ("Value"=w1782:u32)  [unwired: 2 in, 2 out]
        n831 = property on="R steps/rev" class="DigNum (strict)"() -> ("Value"=w1789:u32)  [unwired: 2 in, 2 out]
        n832 = property on="R steps/rev" class="DigNum (strict)"() -> ("Value"=w1758:u32)  [unwired: 2 in, 2 out]
        n833 = property on="R offset deg" class="DigNum (strict)"() -> ("Value"=w1757:dbl)  [unwired: 2 in, 2 out]
        n834 = property on="X offset mm" class="DigNum (strict)"() -> ("Value"=w1773:dbl)  [unwired: 2 in, 2 out]
        n835 = property on="Z offset mm" class="DigNum (strict)"() -> ("Value"=w1765:dbl)  [unwired: 2 in, 2 out]
        n836 = property on="Y offset mm" class="DigNum (strict)"() -> ("Value"=w1781:dbl)  [unwired: 2 in, 2 out]
        n837 = To Double Precision Float(number=w1801) -> (double precision float=w1806:dbl)
        n838 = To Double Precision Float(number=w1776) -> (double precision float=w1777:dbl)
        n839 = To Double Precision Float(number=w1774) -> (double precision float=w1780:dbl)
        n840 = To Double Precision Float(number=w1789) -> (double precision float=w1794:dbl)
        n841 = To Double Precision Float(number=w1760) -> (double precision float=w1761:dbl)
        n842 = To Double Precision Float(number=w1758) -> (double precision float=w1764:dbl)
        n843 = To Double Precision Float(number=w1795) -> (double precision float=w1800:dbl)
        n844 = To Double Precision Float(number=w1768) -> (double precision float=w1769:dbl)
        n845 = To Double Precision Float(number=w1766) -> (double precision float=w1772:dbl)
        n846 = To Double Precision Float(number=w1807) -> (double precision float=w1812:dbl)
        n847 = To Double Precision Float(number=w1784) -> (double precision float=w1785:dbl)
        n848 = To Double Precision Float(number=w1782) -> (double precision float=w1788:dbl)
        n849 = Divide(x=w1777, y=w1780) -> (x/y=w1779:dbl)
        n850 = Divide(x=w1769, y=w1772) -> (x/y=w1771:dbl)
        n851 = Divide(x=w1785, y=w1788) -> (x/y=w1787:dbl)
        n852 = Divide(x=w1761, y=w1764) -> (x/y=w1763:dbl)
        n853 = property on="X Velocity SP step/sec" class="DigNum (strict)"() -> ("Value"=w1803:i32)  [unwired: 2 in, 2 out]
        n854 = property on="X mm/rev" class="DigNum (strict)"() -> ("Value"=w1754:dbl)  [unwired: 2 in, 2 out]
        n855 = property on="Z Velocity SP step/sec" class="DigNum (strict)"() -> ("Value"=w1797:i32)  [unwired: 2 in, 2 out]
        n856 = property on="Z mm/rev" class="DigNum (strict)"() -> ("Value"=w1755:dbl)  [unwired: 2 in, 2 out]
        n857 = property on="Y Velocity SP step/sec" class="DigNum (strict)"() -> ("Value"=w1809:i32)  [unwired: 2 in, 2 out]
        n858 = property on="Y mm/rev" class="DigNum (strict)"() -> ("Value"=w1753:dbl)  [unwired: 2 in, 2 out]
        n859 = property on="R Velocity SP step/sec" class="DigNum (strict)"() -> ("Value"=w1791:i32)  [unwired: 2 in, 2 out]
        n860 = property on="R deg/rev" class="DigNum (strict)"() -> ("Value"=w1756:dbl)  [unwired: 2 in, 2 out]
        n861 = Multiply(x=w1779, y=w1754) -> (x*y=w1778:dbl)
        n862 = Multiply(x=w1763, y=w1756) -> (x*y=w1762:dbl)
        n863 = Multiply(x=w1771, y=w1755) -> (x*y=w1770:dbl)
        n864 = Multiply(x=w1787, y=w1753) -> (x*y=w1786:dbl)
        n865 = To Double Precision Float(number=w1803) -> (double precision float=w1804:dbl)
        n866 = To Double Precision Float(number=w1791) -> (double precision float=w1792:dbl)
        n867 = To Double Precision Float(number=w1797) -> (double precision float=w1798:dbl)
        n868 = To Double Precision Float(number=w1809) -> (double precision float=w1810:dbl)
        n869 = Divide(x=w1804, y=w1806) -> (x/y=w1805:dbl)
        n870 = Add(x=w1778, y=w1773) -> (x+y=w1775:dbl)
        n871 = Divide(x=w1792, y=w1794) -> (x/y=w1793:dbl)
        n872 = Add(x=w1762, y=w1757) -> (x+y=w1759:dbl)
        n873 = Divide(x=w1798, y=w1800) -> (x/y=w1799:dbl)
        n874 = Add(x=w1770, y=w1765) -> (x+y=w1767:dbl)
        n875 = Divide(x=w1810, y=w1812) -> (x/y=w1811:dbl)
        n876 = Add(x=w1786, y=w1781) -> (x+y=w1783:dbl)
        n877 = Multiply(x=w1805, y=w1754) -> (x*y=w1802:dbl)
        n878 = Multiply(x=w1793, y=w1756) -> (x*y=w1790:dbl)
        n879 = Multiply(x=w1799, y=w1755) -> (x*y=w1796:dbl)
        n880 = Multiply(x=w1811, y=w1753) -> (x*y=w1808:dbl)
        n881 = property on="X Position MV mm" class="DigNum (strict)"("Val(Sgnl)"=w1775) -> ()  [unwired: 2 in, 2 out]
        n882 = property on="R Position MV deg" class="DigNum (strict)"("Val(Sgnl)"=w1759) -> ()  [unwired: 2 in, 2 out]
        n883 = property on="Z Position MV mm" class="DigNum (strict)"("Val(Sgnl)"=w1767) -> ()  [unwired: 2 in, 2 out]
        n884 = property on="Y Position MV mm" class="DigNum (strict)"("Val(Sgnl)"=w1783) -> ()  [unwired: 2 in, 2 out]
        n885 = property on="X Velocity MV mm/sec" class="DigNum (strict)"("Val(Sgnl)"=w1802) -> ()  [unwired: 2 in, 2 out]
        n886 = property on="Z Velocity MV mm/sec" class="DigNum (strict)"("Val(Sgnl)"=w1796) -> ()  [unwired: 2 in, 2 out]
        n887 = property on="Y Velocity MV mm/sec" class="DigNum (strict)"("Val(Sgnl)"=w1808) -> ()  [unwired: 2 in, 2 out]
        n888 = Absolute Value(x=w1790) -> (abs(x)=w1752:dbl)
        n889 = property on="R Velocity MVdeg/sec" class="DigNum (strict)"("Val(Sgnl)"=w1752) -> ()  [unwired: 2 in, 2 out]
      }
      event #6 {
        n890 = event-data() -> ()  [unwired: 1 in, 5 out]
        n891 = property on="R Step PV" class="DigNum (strict)"() -> ("Value"=w1845:i32)  [unwired: 2 in, 2 out]
        n892 = property on="X steps/rev" class="DigNum (strict)"() -> ("Value"=w1886:u32)  [unwired: 2 in, 2 out]
        n893 = property on="Y steps/rev" class="DigNum (strict)"() -> ("Value"=w1874:u32)  [unwired: 2 in, 2 out]
        n894 = property on="Z steps/rev" class="DigNum (strict)"() -> ("Value"=w1861:u32)  [unwired: 2 in, 2 out]
        n895 = property on="X Step PV" class="DigNum (strict)"() -> ("Value"=w1885:i32)  [unwired: 2 in, 2 out]
        n896 = property on="Y Step PV" class="DigNum (strict)"() -> ("Value"=w1872:i32)  [unwired: 2 in, 2 out]
        n897 = property on="Z Step PV" class="DigNum (strict)"() -> ("Value"=w1859:i32)  [unwired: 2 in, 2 out]
        n898 = property on="R steps/rev" class="DigNum (strict)"() -> ("Value"=w1847:u32)  [unwired: 2 in, 2 out]
        n899 = To Double Precision Float(number=w1885) -> (double precision float=w1839:dbl)
        n900 = To Double Precision Float(number=w1872) -> (double precision float=w1838:dbl)
        n901 = To Double Precision Float(number=w1859) -> (double precision float=w1837:dbl)
        n902 = To Double Precision Float(number=w1845) -> (double precision float=w1836:dbl)
        n903 = To Double Precision Float(number=w1886) -> (double precision float=w1884:dbl)
        n904 = To Double Precision Float(number=w1874) -> (double precision float=w1829:dbl)
        n905 = To Double Precision Float(number=w1847) -> (double precision float=w1844:dbl)
        n906 = To Double Precision Float(number=w1861) -> (double precision float=w1858:dbl)
        n907 = property on="X Step SP" class="DigNum (strict)"() -> ("Maximum"=w1889:dbl)  [unwired: 2 in, 2 out]
        n908 = property on="Y Step SP" class="DigNum (strict)"() -> ("Maximum"=w1878:dbl)  [unwired: 2 in, 2 out]
        n909 = property on="Z Step SP" class="DigNum (strict)"() -> ("Maximum"=w1865:dbl)  [unwired: 2 in, 2 out]
        n910 = property on="R Step SP" class="DigNum (strict)"() -> ("Maximum"=w1853:dbl)  [unwired: 2 in, 2 out]
        n911 = property on="X Scan Length SP steps" class="DigNum (strict)"() -> ("Value"=w1883:i32)  [unwired: 2 in, 2 out]
        n912 = property on="X Scan Length SP mm" class="DigNum (strict)"() -> ("Value"=w1815:dbl)  [unwired: 2 in, 2 out]
        n913 = property on="Y Scan Length SP mm" class="DigNum (strict)"() -> ("Value"=w1816:dbl)  [unwired: 2 in, 2 out]
        n914 = property on="Y Scan Length SP steps" class="DigNum (strict)"() -> ("Value"=w1875:i32)  [unwired: 2 in, 2 out]
        n915 = property on="Z Scan Length SP steps" class="DigNum (strict)"() -> ("Value"=w1862:i32)  [unwired: 2 in, 2 out]
        n916 = property on="R Scan Length SP steps" class="DigNum (strict)"() -> ("Value"=w1848:i32)  [unwired: 2 in, 2 out]
        n917 = property on="X Step SP" class="DigNum (strict)"() -> ("Minimum"=w1890:dbl)  [unwired: 2 in, 2 out]
        n918 = property on="Y Step SP" class="DigNum (strict)"() -> ("Minimum"=w1879:dbl)  [unwired: 2 in, 2 out]
        n919 = property on="Z Step SP" class="DigNum (strict)"() -> ("Minimum"=w1866:dbl)  [unwired: 2 in, 2 out]
        n920 = property on="R Step SP" class="DigNum (strict)"() -> ("Minimum"=w1850:dbl)  [unwired: 2 in, 2 out]
        n921 = property on="Z Scan Velocity SP steps/sec" class="DigNum (strict)"() -> ("Value"=w1857:i32)  [unwired: 2 in, 2 out]
        n922 = property on="R Scan Velocity SP steps/sec" class="DigNum (strict)"() -> ("Value"=w1843:i32)  [unwired: 2 in, 2 out]
        n923 = Subtract(x=w1889, y=w1839) -> (x-y=w1888:dbl)
        n924 = Subtract(x=w1890, y=w1839) -> (x-y=w1891:dbl)
        n925 = Subtract(x=w1879, y=w1838) -> (x-y=w1880:dbl)
        n926 = Subtract(x=w1878, y=w1838) -> (x-y=w1877:dbl)
        n927 = Subtract(x=w1866, y=w1837) -> (x-y=w1867:dbl)
        n928 = Subtract(x=w1865, y=w1837) -> (x-y=w1864:dbl)
        n929 = Subtract(x=w1850, y=w1836) -> (x-y=w1851:dbl)
        n930 = Subtract(x=w1853, y=w1836) -> (x-y=w1852:dbl)
        n931 = To Double Precision Float(number=w1848) -> (double precision float=w1833:dbl)
        n932 = To Double Precision Float(number=w1862) -> (double precision float=w1835:dbl)
        n933 = To Double Precision Float(number=w1883) -> (double precision float=w1826:dbl)
        n934 = To Double Precision Float(number=w1875) -> (double precision float=w1828:dbl)
        n935 = property on="X Scan Velocity SP steps/sec" class="DigNum (strict)"() -> ("Value"=w1887:i32)  [unwired: 2 in, 2 out]
        n936 = property on="Y Scan Velocity SP steps/sec" class="DigNum (strict)"() -> ("Value"=w1871:i32)  [unwired: 2 in, 2 out]
        n937 = Equal?(x=w1815, y=0.0) -> (x = y?=w1813:bool)
        n938 = Equal?(x=w1816, y=0.0) -> (x = y?=w1814:bool)
        n939 = property on="X Scan Length SP steps" class="DigNum (strict)"("Maximum"=w1888) -> ()  [unwired: 2 in, 2 out]
        n940 = property on="X Scan Length SP steps" class="DigNum (strict)"("Minimum"=w1891) -> ()  [unwired: 2 in, 2 out]
        n941 = property on="Y Scan Length SP steps" class="DigNum (strict)"("Minimum"=w1880) -> ()  [unwired: 2 in, 2 out]
        n942 = property on="Y Scan Length SP steps" class="DigNum (strict)"("Maximum"=w1877) -> ()  [unwired: 2 in, 2 out]
        n943 = property on="Z Scan Length SP steps" class="DigNum (strict)"("Minimum"=w1867) -> ()  [unwired: 2 in, 2 out]
        n944 = property on="Z Scan Length SP steps" class="DigNum (strict)"("Maximum"=w1864) -> ()  [unwired: 2 in, 2 out]
        n945 = property on="R Scan Length SP steps" class="DigNum (strict)"("Minimum"=w1851) -> ()  [unwired: 2 in, 2 out]
        n946 = property on="R Scan Length SP steps" class="DigNum (strict)"("Maximum"=w1852) -> ()  [unwired: 2 in, 2 out]
        n947 = Divide(x=w1826, y=w1884) -> (x/y=w1821:dbl)
        n948 = Divide(x=w1828, y=w1829) -> (x/y=w1876:dbl)
        n949 = Divide(x=w1835, y=w1858) -> (x/y=w1863:dbl)
        n950 = Divide(x=w1833, y=w1844) -> (x/y=w1849:dbl)
        n951 = To Double Precision Float(number=w1887) -> (double precision float=w1825:dbl)
        n952 = To Double Precision Float(number=w1871) -> (double precision float=w1827:dbl)
        n953 = To Double Precision Float(number=w1857) -> (double precision float=w1834:dbl)
        n954 = To Double Precision Float(number=w1843) -> (double precision float=w1832:dbl)
        n955 = property on="X mm/rev" class="DigNum (strict)"() -> ("Value"=w1820:dbl)  [unwired: 2 in, 2 out]
        n956 = property on="Y mm/rev" class="DigNum (strict)"() -> ("Value"=w1873:dbl)  [unwired: 2 in, 2 out]
        n957 = property on="Z mm/rev" class="DigNum (strict)"() -> ("Value"=w1860:dbl)  [unwired: 2 in, 2 out]
        n958 = property on="R deg/rev" class="DigNum (strict)"() -> ("Value"=w1846:dbl)  [unwired: 2 in, 2 out]
        n959 = Multiply(x=w1821, y=w1820) -> (x*y=w1881:dbl)
        n960 = Divide(x=w1825, y=w1884) -> (x/y=w1819:dbl)
        n961 = Multiply(x=w1876, y=w1873) -> (x*y=w1869:dbl)
        n962 = Divide(x=w1827, y=w1829) -> (x/y=w1870:dbl)
        n963 = Divide(x=w1833, y=w1832) -> (x/y=w1831:dbl)
        n964 = Multiply(x=w1849, y=w1846) -> (x*y=w1841:dbl)
        n965 = Divide(x=w1832, y=w1844) -> (x/y=w1842:dbl)
        n966 = Multiply(x=w1863, y=w1860) -> (x*y=w1855:dbl)
        n967 = Divide(x=w1835, y=w1834) -> (x/y=w1830:dbl)
        n968 = Divide(x=w1834, y=w1858) -> (x/y=w1856:dbl)
        n969 = case shown="True" w1813 {
          tunnel: w1826 -> [w1894 _]
          tunnel: w1825 -> [w1893 _]
          frame #0 {
            n970 = Divide(x=w1894, y=w1893) -> (x/y=w1895:dbl)
            n971 = Absolute Value(x=w1895) -> (abs(x)=→"X Scan Duration":dbl)
          }
          frame #1 {
            n972 = local write "X Scan Duration"(0.0 ("X Scan Duration")) -> ()
          }
        }
        n973 = case shown="True" w1814 {
          tunnel: w1828 -> [w1900 _]
          tunnel: w1827 -> [w1899 _]
          frame #0 {
            n974 = Divide(x=w1900, y=w1899) -> (x/y=w1898:dbl)
            n975 = Absolute Value(x=w1898) -> (abs(x)=→"Y Scan Duration":dbl)
          }
          frame #1 {
            n976 = local write "Y Scan Duration"(0.0 ("Y Scan Duration")) -> ()
          }
        }
        n977 = Multiply(x=w1820, y=w1819) -> (x*y=w1882:dbl)
        n978 = Multiply(x=w1873, y=w1870) -> (x*y=w1868:dbl)
        n979 = Multiply(x=w1846, y=w1842) -> (x*y=w1840:dbl)
        n980 = Multiply(x=w1860, y=w1856) -> (x*y=w1854:dbl)
        n981 = Absolute Value(x=w1831) -> (abs(x)=→"R Scan Duration":dbl)
        n982 = Absolute Value(x=w1830) -> (abs(x)=→"Z Scan Duration":dbl)
        n983 = property on="X Scan length MV mm" class="DigNum (strict)"("Val(Sgnl)"=w1881) -> ()  [unwired: 2 in, 2 out]
        n984 = property on="Y Scan length MV mm" class="DigNum (strict)"("Value"=w1869) -> ()  [unwired: 2 in, 2 out]
        n985 = property on="R Scan length MV deg" class="DigNum (strict)"("Value"=w1841) -> ()  [unwired: 2 in, 2 out]
        n986 = property on="Z Scan length MV mm" class="DigNum (strict)"("Value"=w1855) -> ()  [unwired: 2 in, 2 out]
        n987 = Absolute Value(x=w1840) -> (abs(x)=w1824:dbl)
        n988 = property on="X Scan velocity MV mm/sec" class="DigNum (strict)"("Value"=w1882) -> ()  [unwired: 2 in, 2 out]
        n989 = property on="Y Scan velocity MV mm/sec" class="DigNum (strict)"("Val(Sgnl)"=w1868) -> ()  [unwired: 2 in, 2 out]
        n990 = property on="Z Scan velocity MV mm/sec" class="DigNum (strict)"("Val(Sgnl)"=w1854) -> ()  [unwired: 2 in, 2 out]
        n991 = property on="R Scan Velocity SP deg/sec" class="DigNum (strict)"("Val(Sgnl)"=w1824) -> ()  [unwired: 2 in, 2 out]
      }
      event #7 {
        n992 = event-data() -> ()  [unwired: 1 in, 7 out]
        n993 = property on="Y steps/rev" class="DigNum (strict)"() -> ("Value"=w1920:u32)  [unwired: 2 in, 2 out]
        n994 = Wait (ms)(milliseconds to wait=u32 100) -> ()  [unwired: 1 out]
        n995 = To Double Precision Float(number=w1920) -> (double precision float=w1905:dbl)
        n996 = property on="Y offset mm" class="DigNum (strict)"() -> ("Value"=w1918:dbl)  [unwired: 2 in, 2 out]
        n997 = property on="Y Position SP mm" class="DigNum (strict)"() -> ("Value"=w1917:dbl)  [unwired: 2 in, 2 out]
        n998 = property on="Y Velocity SP step/sec" class="DigNum (strict)"() -> ("Maximum"=w1907:dbl)  [unwired: 2 in, 2 out]
        n999 = local write "STATUS"("SETTING Y" ("STATUS")) -> ()
        n1000 = property on="Y Velocity SP step/sec" class="DigNum (strict)"() -> ("Minimum"=w1906:dbl)  [unwired: 2 in, 2 out]
        n1001 = Subtract(x=w1917, y=w1918) -> (x-y=w1921:dbl)
        n1002 = property on="Y Velocity SP mm/sec" class="DigNum (strict)"() -> ("Value"=w1911:dbl)  [unwired: 2 in, 2 out]
        n1003 = property on="Y mm/rev" class="DigNum (strict)"() -> ("Value"=w1904:dbl)  [unwired: 2 in, 2 out]
        n1004 = Divide(x=w1921, y=w1904) -> (x/y=w1922:dbl)
        n1005 = Divide(x=w1911, y=w1904) -> (x/y=w1912:dbl)
        n1006 = Multiply(x=w1922, y=w1905) -> (x*y=w1916:dbl)
        n1007 = Multiply(x=w1912, y=w1905) -> (x*y=w1909:dbl)
        n1008 = property on="Y Step SP" class="DigNum (strict)"() -> ("Maximum"=w1914:dbl)  [unwired: 2 in, 2 out]
        n1009 = property on="Y Step SP" class="DigNum (strict)"() -> ("Minimum"=w1913:dbl)  [unwired: 2 in, 2 out]
        n1010 = In Range and Coerce(upper limit=w1907, x=w1909, lower limit=w1906) -> (coerced(x)=w1908:dbl)  [unwired: 1 out]
        n1011 = To Long Integer(number=w1908) -> (32bit integer=w1910:i32)
        n1012 = In Range and Coerce(upper limit=w1914, x=w1916, lower limit=w1913) -> (coerced(x)=w1915:dbl)  [unwired: 1 out]
        n1013 = To Long Integer(number=w1915) -> (32bit integer=w1919:i32)
        n1014 = property on="Y Velocity SP step/sec" class="DigNum (strict)"("Val(Sgnl)"=w1910) -> ()  [unwired: 2 in, 2 out]
        n1015 = property on="Y Step SP" class="DigNum (strict)"("Val(Sgnl)"=w1919) -> ()  [unwired: 2 in, 2 out]
      }
      event #8 {
        n1016 = event-data() -> ()  [unwired: 1 in, 7 out]
        n1017 = property on="X steps/rev" class="DigNum (strict)"() -> ("Value"=w1941:u32)  [unwired: 2 in, 2 out]
        n1018 = Wait (ms)(milliseconds to wait=u32 100) -> ()  [unwired: 1 out]
        n1019 = property on="X offset mm" class="DigNum (strict)"() -> ("Value"=w1939:dbl)  [unwired: 2 in, 2 out]
        n1020 = property on="X Position SP mm" class="DigNum (strict)"() -> ("Value"=w1938:dbl)  [unwired: 2 in, 2 out]
        n1021 = property on="X Velocity SP step/sec" class="DigNum (strict)"() -> ("Maximum"=w1928:dbl)  [unwired: 2 in, 2 out]
        n1022 = local write "STATUS"("SETTING X" ("STATUS")) -> ()
        n1023 = property on="X Velocity SP step/sec" class="DigNum (strict)"() -> ("Minimum"=w1927:dbl)  [unwired: 2 in, 2 out]
        n1024 = Subtract(x=w1938, y=w1939) -> (x-y=w1942:dbl)
        n1025 = property on="X Velocity SP mm/sec" class="DigNum (strict)"() -> ("Value"=w1932:dbl)  [unwired: 2 in, 2 out]
        n1026 = property on="X mm/rev" class="DigNum (strict)"() -> ("Value"=w1925:dbl)  [unwired: 2 in, 2 out]
        n1027 = Divide(x=w1942, y=w1925) -> (x/y=w1943:dbl)
        n1028 = Divide(x=w1932, y=w1925) -> (x/y=w1933:dbl)
        n1029 = To Double Precision Float(number=w1941) -> (double precision float=w1926:dbl)
        n1030 = Multiply(x=w1943, y=w1926) -> (x*y=w1937:dbl)
        n1031 = Multiply(x=w1933, y=w1926) -> (x*y=w1930:dbl)
        n1032 = property on="X Step SP" class="DigNum (strict)"() -> ("Maximum"=w1935:dbl)  [unwired: 2 in, 2 out]
        n1033 = property on="X Step SP" class="DigNum (strict)"() -> ("Minimum"=w1934:dbl)  [unwired: 2 in, 2 out]
        n1034 = In Range and Coerce(upper limit=w1928, x=w1930, lower limit=w1927) -> (coerced(x)=w1929:dbl)  [unwired: 1 out]
        n1035 = To Long Integer(number=w1929) -> (32bit integer=w1931:i32)
        n1036 = In Range and Coerce(upper limit=w1935, x=w1937, lower limit=w1934) -> (coerced(x)=w1936:dbl)  [unwired: 1 out]
        n1037 = To Long Integer(number=w1936) -> (32bit integer=w1940:i32)
        n1038 = property on="X Velocity SP step/sec" class="DigNum (strict)"("Val(Sgnl)"=w1931) -> ()  [unwired: 2 in, 2 out]
        n1039 = property on="X Step SP" class="DigNum (strict)"("Val(Sgnl)"=w1940) -> ()  [unwired: 2 in, 2 out]
      }
      event #9 {
        n1040 = event-data() -> ()  [unwired: 1 in, 7 out]
        n1041 = property on="Z steps/rev" class="DigNum (strict)"() -> ("Value"=w1960:u32)  [unwired: 2 in, 2 out]
        n1042 = Wait (ms)(milliseconds to wait=u32 100) -> ()  [unwired: 1 out]
        n1043 = property on="Z offset mm" class="DigNum (strict)"() -> ("Value"=w1958:dbl)  [unwired: 2 in, 2 out]
        n1044 = property on="Z Position SP mm" class="DigNum (strict)"() -> ("Value"=w1957:dbl)  [unwired: 2 in, 2 out]
        n1045 = property on="Z Velocity SP step/sec" class="DigNum (strict)"() -> ("Maximum"=w1947:dbl)  [unwired: 2 in, 2 out]
        n1046 = local write "STATUS"("SETTING Z" ("STATUS")) -> ()
        n1047 = property on="Z Velocity SP step/sec" class="DigNum (strict)"() -> ("Minimum"=w1946:dbl)  [unwired: 2 in, 2 out]
        n1048 = Subtract(x=w1957, y=w1958) -> (x-y=w1961:dbl)
        n1049 = property on="Z Velocity SP mm/sec" class="DigNum (strict)"() -> ("Value"=w1951:dbl)  [unwired: 2 in, 2 out]
        n1050 = property on="Z mm/rev" class="DigNum (strict)"() -> ("Value"=w1963:dbl)  [unwired: 2 in, 2 out]
        n1051 = Divide(x=w1961, y=w1963) -> (x/y=w1962:dbl)
        n1052 = Divide(x=w1951, y=w1963) -> (x/y=w1952:dbl)
        n1053 = To Double Precision Float(number=w1960) -> (double precision float=w1964:dbl)
        n1054 = Multiply(x=w1962, y=w1964) -> (x*y=w1956:dbl)
        n1055 = Multiply(x=w1952, y=w1964) -> (x*y=w1949:dbl)
        n1056 = property on="Z Step SP" class="DigNum (strict)"() -> ("Maximum"=w1954:dbl)  [unwired: 2 in, 2 out]
        n1057 = property on="Z Step SP" class="DigNum (strict)"() -> ("Minimum"=w1953:dbl)  [unwired: 2 in, 2 out]
        n1058 = In Range and Coerce(upper limit=w1947, x=w1949, lower limit=w1946) -> (coerced(x)=w1948:dbl)  [unwired: 1 out]
        n1059 = To Long Integer(number=w1948) -> (32bit integer=w1950:i32)
        n1060 = In Range and Coerce(upper limit=w1954, x=w1956, lower limit=w1953) -> (coerced(x)=w1955:dbl)  [unwired: 1 out]
        n1061 = To Long Integer(number=w1955) -> (32bit integer=w1959:i32)
        n1062 = property on="Z Velocity SP step/sec" class="DigNum (strict)"("Val(Sgnl)"=w1950) -> ()  [unwired: 2 in, 2 out]
        n1063 = property on="Z Step SP" class="DigNum (strict)"("Val(Sgnl)"=w1959) -> ()  [unwired: 2 in, 2 out]
      }
      event #10 {
        n1064 = event-data() -> ()  [unwired: 1 in, 7 out]
        n1065 = property on="R steps/rev" class="DigNum (strict)"() -> ("Value"=w1984:u32)  [unwired: 2 in, 2 out]
        n1066 = Wait (ms)(milliseconds to wait=u32 100) -> ()  [unwired: 1 out]
        n1067 = property on="R offset deg" class="DigNum (strict)"() -> ("Value"=w1982:dbl)  [unwired: 2 in, 2 out]
        n1068 = property on="R Position SP deg" class="DigNum (strict)"() -> ("Value"=w1981:dbl)  [unwired: 2 in, 2 out]
        n1069 = property on="R Velocity SP step/sec" class="DigNum (strict)"() -> ("Maximum"=w1971:dbl)  [unwired: 2 in, 2 out]
        n1070 = local write "STATUS"("SETTING R" ("STATUS")) -> ()
        n1071 = property on="R Velocity SP step/sec" class="DigNum (strict)"() -> ("Minimum"=w1970:dbl)  [unwired: 2 in, 2 out]
        n1072 = Subtract(x=w1981, y=w1982) -> (x-y=w1985:dbl)
        n1073 = property on="R Velocity SP deg/sec" class="DigNum (strict)"() -> ("Value"=w1975:dbl)  [unwired: 2 in, 2 out]
        n1074 = property on="R deg/rev" class="DigNum (strict)"() -> ("Value"=w1968:dbl)  [unwired: 2 in, 2 out]
        n1075 = Divide(x=w1985, y=w1968) -> (x/y=w1986:dbl)
        n1076 = Divide(x=w1975, y=w1968) -> (x/y=w1976:dbl)
        n1077 = To Double Precision Float(number=w1984) -> (double precision float=w1969:dbl)
        n1078 = Multiply(x=w1986, y=w1969) -> (x*y=w1980:dbl)
        n1079 = Multiply(x=w1976, y=w1969) -> (x*y=w1973:dbl)
        n1080 = property on="R Step SP" class="DigNum (strict)"() -> ("Maximum"=w1978:dbl)  [unwired: 2 in, 2 out]
        n1081 = property on="R Step SP" class="DigNum (strict)"() -> ("Minimum"=w1977:dbl)  [unwired: 2 in, 2 out]
        n1082 = Absolute Value(x=w1973) -> (abs(x)=w1967:dbl)
        n1083 = In Range and Coerce(upper limit=w1978, x=w1980, lower limit=w1977) -> (coerced(x)=w1979:dbl)  [unwired: 1 out]
        n1084 = In Range and Coerce(upper limit=w1971, x=w1967, lower limit=w1970) -> (coerced(x)=w1972:dbl)  [unwired: 1 out]
        n1085 = To Long Integer(number=w1979) -> (32bit integer=w1983:i32)
        n1086 = To Long Integer(number=w1972) -> (32bit integer=w1974:i32)
        n1087 = property on="R Step SP" class="DigNum (strict)"("Val(Sgnl)"=w1983) -> ()  [unwired: 2 in, 2 out]
        n1088 = property on="R Velocity SP step/sec" class="DigNum (strict)"("Val(Sgnl)"=w1974) -> ()  [unwired: 2 in, 2 out]
      }
      event #11 {
        n1089 = event-data() -> ()  [unwired: 1 in, 7 out]
        n1090 = flat-sequence {
          frame #0 {
            n1091 = property on="Z steps/rev" class="DigNum (strict)"() -> ("Value"=w2055:u32)  [unwired: 2 in, 2 out]
            n1092 = property on="X steps/rev" class="DigNum (strict)"() -> ("Value"=w2038:u32)  [unwired: 2 in, 2 out]
            n1093 = property on="Y steps/rev" class="DigNum (strict)"() -> ("Value"=w2003:u32)  [unwired: 2 in, 2 out]
            n1094 = property on="R steps/rev" class="DigNum (strict)"() -> ("Value"=w2021:u32)  [unwired: 2 in, 2 out]
            n1095 = To Double Precision Float(number=w2055) -> (double precision float=w2041:dbl)
            n1096 = To Double Precision Float(number=w2038) -> (double precision float=w2024:dbl)
            n1097 = To Double Precision Float(number=w2003) -> (double precision float=w1989:dbl)
            n1098 = To Double Precision Float(number=w2021) -> (double precision float=w2007:dbl)
            n1099 = property on="R Velocity SP step/sec" class="DigNum (strict)"() -> ("Maximum"=w2009:dbl)  [unwired: 2 in, 2 out]
            n1100 = property on="Z mm/rev" class="DigNum (strict)"() -> ("Value"=w2040:dbl)  [unwired: 2 in, 2 out]
            n1101 = property on="X mm/rev" class="DigNum (strict)"() -> ("Value"=w2023:dbl)  [unwired: 2 in, 2 out]
            n1102 = property on="Y mm/rev" class="DigNum (strict)"() -> ("Value"=w1988:dbl)  [unwired: 2 in, 2 out]
            n1103 = property on="Z Scan Length SP mm" class="DigNum (strict)"() -> ("Value"=w2053:dbl)  [unwired: 2 in, 2 out]
            n1104 = property on="Z Scan Velocity SP mm/sec" class="DigNum (strict)"() -> ("Value"=w2047:dbl)  [unwired: 2 in, 2 out]
            n1105 = property on="X Scan Length SP mm" class="DigNum (strict)"() -> ("Value"=w2036:dbl)  [unwired: 2 in, 2 out]
            n1106 = property on="X Scan Velocity SP mm/sec" class="DigNum (strict)"() -> ("Value"=w2030:dbl)  [unwired: 2 in, 2 out]
            n1107 = property on="Y Scan Length SP mm" class="DigNum (strict)"() -> ("Value"=w2001:dbl)  [unwired: 2 in, 2 out]
            n1108 = property on="Y Scan Velocity SP mm/sec" class="DigNum (strict)"() -> ("Value"=w1995:dbl)  [unwired: 2 in, 2 out]
            n1109 = property on="R Scan Length SP deg" class="DigNum (strict)"() -> ("Value"=w2019:dbl)  [unwired: 2 in, 2 out]
            n1110 = property on="R deg/rev" class="DigNum (strict)"() -> ("Value"=w2006:dbl)  [unwired: 2 in, 2 out]
            n1111 = property on="Z Scan Velocity SP steps/sec" class="DigNum (strict)"() -> ("Maximum"=w2043:dbl)  [unwired: 2 in, 2 out]
            n1112 = property on="X Scan Velocity SP steps/sec" class="DigNum (strict)"() -> ("Maximum"=w2026:dbl)  [unwired: 2 in, 2 out]
            n1113 = property on="Y Scan Velocity SP steps/sec" class="DigNum (strict)"() -> ("Maximum"=w1991:dbl)  [unwired: 2 in, 2 out]
            n1114 = property on="R Scan Velocity SP steps/sec" class="DigNum (strict)"() -> ("Minimum"=w2008:dbl)  [unwired: 2 in, 2 out]
            n1115 = property on="Z Scan Velocity SP steps/sec" class="DigNum (strict)"() -> ("Minimum"=w2042:dbl)  [unwired: 2 in, 2 out]
            n1116 = property on="X Scan Velocity SP steps/sec" class="DigNum (strict)"() -> ("Minimum"=w2025:dbl)  [unwired: 2 in, 2 out]
            n1117 = property on="Y Scan Velocity SP steps/sec" class="DigNum (strict)"() -> ("Minimum"=w1990:dbl)  [unwired: 2 in, 2 out]
            n1118 = property on="R Scan Velocity SP deg/sec" class="DigNum (strict)"() -> ("Value"=w2013:dbl)  [unwired: 2 in, 2 out]
            n1119 = Divide(x=w2053, y=w2040) -> (x/y=w2056:dbl)
            n1120 = Divide(x=w2047, y=w2040) -> (x/y=w2048:dbl)
            n1121 = Divide(x=w2036, y=w2023) -> (x/y=w2039:dbl)
            n1122 = Divide(x=w2030, y=w2023) -> (x/y=w2031:dbl)
            n1123 = Divide(x=w2001, y=w1988) -> (x/y=w2004:dbl)
            n1124 = Divide(x=w1995, y=w1988) -> (x/y=w1996:dbl)
            n1125 = Divide(x=w2019, y=w2006) -> (x/y=w2022:dbl)
            n1126 = Multiply(x=w2056, y=w2041) -> (x*y=w2052:dbl)
            n1127 = Multiply(x=w2048, y=w2041) -> (x*y=w2045:dbl)
            n1128 = Multiply(x=w2039, y=w2024) -> (x*y=w2035:dbl)
            n1129 = Multiply(x=w2031, y=w2024) -> (x*y=w2028:dbl)
            n1130 = Multiply(x=w2004, y=w1989) -> (x*y=w2000:dbl)
            n1131 = Multiply(x=w1996, y=w1989) -> (x*y=w1993:dbl)
            n1132 = Multiply(x=w2022, y=w2007) -> (x*y=w2018:dbl)
            n1133 = Divide(x=w2013, y=w2006) -> (x/y=w2014:dbl)
            n1134 = property on="Z Step SP" class="DigNum (strict)"() -> ("Maximum"=w2049:dbl)  [unwired: 2 in, 2 out]
            n1135 = property on="X Step SP" class="DigNum (strict)"() -> ("Maximum"=w2032:dbl)  [unwired: 2 in, 2 out]
            n1136 = property on="Y Step SP" class="DigNum (strict)"() -> ("Maximum"=w1997:dbl)  [unwired: 2 in, 2 out]
            n1137 = property on="R Step SP" class="DigNum (strict)"() -> ("Maximum"=w2015:dbl)  [unwired: 2 in, 2 out]
            n1138 = property on="Z Step SP" class="DigNum (strict)"() -> ("Minimum"=w2050:dbl)  [unwired: 2 in, 2 out]
            n1139 = property on="X Step SP" class="DigNum (strict)"() -> ("Minimum"=w2033:dbl)  [unwired: 2 in, 2 out]
            n1140 = property on="Y Step SP" class="DigNum (strict)"() -> ("Minimum"=w1998:dbl)  [unwired: 2 in, 2 out]
            n1141 = property on="R Step SP" class="DigNum (strict)"() -> ("Minimum"=w2016:dbl)  [unwired: 2 in, 2 out]
            n1142 = Multiply(x=w2014, y=w2007) -> (x*y=w2011:dbl)
            n1143 = In Range and Coerce(upper limit=w2043, x=w2045, lower limit=w2042) -> (coerced(x)=w2044:dbl)  [unwired: 1 out]
            n1144 = In Range and Coerce(upper limit=w2026, x=w2028, lower limit=w2025) -> (coerced(x)=w2027:dbl)  [unwired: 1 out]
            n1145 = In Range and Coerce(upper limit=w1991, x=w1993, lower limit=w1990) -> (coerced(x)=w1992:dbl)  [unwired: 1 out]
            n1146 = To Long Integer(number=w2044) -> (32bit integer=w2046:i32)
            n1147 = To Long Integer(number=w2027) -> (32bit integer=w2029:i32)
            n1148 = To Long Integer(number=w1992) -> (32bit integer=w1994:i32)
            n1149 = Absolute Value(x=w2011) -> (abs(x)=w2005:dbl)
            n1150 = In Range and Coerce(upper limit=w2049, x=w2052, lower limit=w2050) -> (coerced(x)=w2051:dbl)  [unwired: 1 out]
            n1151 = In Range and Coerce(upper limit=w2032, x=w2035, lower limit=w2033) -> (coerced(x)=w2034:dbl)  [unwired: 1 out]
            n1152 = In Range and Coerce(upper limit=w1997, x=w2000, lower limit=w1998) -> (coerced(x)=w1999:dbl)  [unwired: 1 out]
            n1153 = In Range and Coerce(upper limit=w2015, x=w2018, lower limit=w2016) -> (coerced(x)=w2017:dbl)  [unwired: 1 out]
            n1154 = To Long Integer(number=w2051) -> (32bit integer=w2054:i32)
            n1155 = To Long Integer(number=w2034) -> (32bit integer=w2037:i32)
            n1156 = To Long Integer(number=w1999) -> (32bit integer=w2002:i32)
            n1157 = To Long Integer(number=w2017) -> (32bit integer=w2020:i32)
            n1158 = property on="Z Scan Velocity SP steps/sec" class="DigNum (strict)"("Val(Sgnl)"=w2046) -> ()  [unwired: 2 in, 2 out]
            n1159 = property on="X Scan Velocity SP steps/sec" class="DigNum (strict)"("Val(Sgnl)"=w2029) -> ()  [unwired: 2 in, 2 out]
            n1160 = property on="Y Scan Velocity SP steps/sec" class="DigNum (strict)"("Val(Sgnl)"=w1994) -> ()  [unwired: 2 in, 2 out]
            n1161 = In Range and Coerce(upper limit=w2009, x=w2005, lower limit=w2008) -> (coerced(x)=w2010:dbl)  [unwired: 1 out]
            n1162 = To Long Integer(number=w2010) -> (32bit integer=w2012:i32)
            n1163 = property on="Z Scan Length SP steps" class="DigNum (strict)"("Val(Sgnl)"=w2054) -> ()  [unwired: 2 in, 2 out]
            n1164 = property on="X Scan Length SP steps" class="DigNum (strict)"("Val(Sgnl)"=w2037) -> ()  [unwired: 2 in, 2 out]
            n1165 = property on="Y Scan Length SP steps" class="DigNum (strict)"("Val(Sgnl)"=w2002) -> ()  [unwired: 2 in, 2 out]
            n1166 = property on="R Scan Length SP steps" class="DigNum (strict)"("Val(Sgnl)"=w2020) -> ()  [unwired: 2 in, 2 out]
            n1167 = property on="R Scan Velocity SP steps/sec" class="DigNum (strict)"("Val(Sgnl)"=w2012) -> ()  [unwired: 2 in, 2 out]
          }
          frame #1 {
            n1168 = case shown="True" "Z as dominating length" {
              frame #0 {
              }
              frame #1 {
                n1169 = property on="Y Scan Length SP steps" class="DigNum (strict)"() -> ("Value"=w2066:i32)  [unwired: 2 in, 2 out]
                n1170 = property on="Z Scan Length SP steps" class="DigNum (strict)"() -> ("Value"=w2065:i32)  [unwired: 2 in, 2 out]
                n1171 = property on="X Scan Length SP steps" class="DigNum (strict)"() -> ("Value"=w2074:i32)  [unwired: 2 in, 2 out]
                n1172 = property on="Z Scan Length SP steps" class="DigNum (strict)"() -> ("Value"=w2073:i32)  [unwired: 2 in, 2 out]
                n1173 = property on="Y Scan Velocity SP steps/sec" class="DigNum (strict)"() -> ("Value"=w2062:i32)  [unwired: 2 in, 2 out]
                n1174 = property on="X Scan Velocity SP steps/sec" class="DigNum (strict)"() -> ("Value"=w2072:i32)  [unwired: 2 in, 2 out]
                n1175 = To Double Precision Float(number=w2066) -> (double precision float=w2064:dbl)
                n1176 = To Double Precision Float(number=w2065) -> (double precision float=w2063:dbl)
                n1177 = To Double Precision Float(number=w2074) -> (double precision float=w2068:dbl)
                n1178 = To Double Precision Float(number=w2073) -> (double precision float=w2069:dbl)
                n1179 = Divide(x=w2064, y=w2063) -> (x/y=w2058:dbl)
                n1180 = Divide(x=w2068, y=w2069) -> (x/y=w2075:dbl)
                n1181 = To Double Precision Float(number=w2062) -> (double precision float=w2061:dbl)
                n1182 = To Double Precision Float(number=w2072) -> (double precision float=w2070:dbl)
                n1183 = Multiply(x=w2058, y=w2061) -> (x*y=w2060:dbl)
                n1184 = Multiply(x=w2075, y=w2070) -> (x*y=w2071:dbl)
                n1185 = To Long Integer(number=w2060) -> (32bit integer=w2059:i32)
                n1186 = To Long Integer(number=w2071) -> (32bit integer=w2067:i32)
                n1187 = property on="Y Scan Velocity SP steps/sec" class="DigNum (strict)"("Val(Sgnl)"=w2059) -> ()  [unwired: 2 in, 2 out]
                n1188 = property on="X Scan Velocity SP steps/sec" class="DigNum (strict)"("Val(Sgnl)"=w2067) -> ()  [unwired: 2 in, 2 out]
              }
            }
          }
          frame #2 {
            w2076 = T9."Enabled" ("Disabled")
            n1189 = property on="Send scan parameter" class="Bool"("DisabledEnum"=w2076) -> ()  [unwired: 2 in, 2 out]
            n1190 = property on="LOOP" class="Bool (strict)"("DisabledEnum"=w2076) -> ()  [unwired: 2 in, 2 out]
          }
        }
        n1191 = local write "STATUS"("SCANNING PARAMETERS SET" ("STATUS")) -> ()
      }
      event #12 {
        n1192 = event-data() -> ()  [unwired: 1 in, 7 out]
        n1193 = flat-sequence {
          tunnel: [w2130] -> w2090
          tunnel: [w2129] -> w2089
          tunnel: w2080 -> [w2128]
          tunnel: w2079 -> [w2127]
          tunnel: w2090 -> [w2136]
          tunnel: [w2136] -> w2088
          tunnel: w2089 -> [w2135]
          tunnel: [w2135] -> w2087
          tunnel: w2088 -> [w2142]
          tunnel: [w2141] -> w2086
          tunnel: w2087 -> [w2140]
          tunnel: [w2139] -> w2085
          tunnel: w2086 -> [w2148]
          tunnel: w2085 -> [w2147]
          tunnel: [w2148] -> w2084
          tunnel: [w2147] -> w2083
          tunnel: w2084 -> [w2153]
          tunnel: w2083 -> [w2152]
          tunnel: [w2153] -> w2082
          tunnel: [w2152] -> w2081
          tunnel: [w2155] -> _
          tunnel: [w2156] -> _
          tunnel: w2082 -> [w2156]
          tunnel: w2081 -> [w2155]
          frame #0 {
            n1194 = property on="R Scan Velocity SP steps/sec" class="DigNum (strict)"() -> ("Value"=w2132:i32)  [unwired: 2 in, 2 out]
            n1195 = Number To Decimal String(number=w2132) -> (decimal integer string=w2133:string)  [unwired: 1 in]
            n1196 = call "mDrive Send Command.vi"("error in (no error)"=w2128, "Extra"=w2133, "Command"=T10."Max Velocity", "VISA resource name"=w2127) -> ("error out"=w2129:errorcluster, "VISA resource name out"=w2130:refnum<visa-resource-name>)  [unwired: 3 in, 1 out]
          }
          frame #1 {
            n1197 = Wait (ms)(milliseconds to wait=u32 100) -> ()  [unwired: 1 out]
          }
          frame #2 {
            # "VELOCITY"
            n1198 = call "mdrive send command.vi"("error in (no error)"=w2140, "Extra"="VM", "Command"=T10."Print Parameter", "VISA resource name"=w2142) -> ("error out"=w2139:errorcluster, "read buffer"=w2144:string, "VISA resource name out"=w2141:refnum<visa-resource-name>)  [unwired: 3 in]
            n1199 = Decimal String To Number(string=w2144, offset=0) -> (number=w2143:i32)  [unwired: 1 in, 1 out]
            n1200 = property on="R velocity PV step/sec" class="DigNum (strict)"("Val(Sgnl)"=w2143) -> ()  [unwired: 2 in, 2 out]
          }
          frame #3 {
            n1201 = Wait (ms)(milliseconds to wait=u32 100) -> ()  [unwired: 1 out]
          }
          frame #4 {
            n1202 = property on="Scan Go" class="Bool (strict)"("DisabledEnum"=T9."Enabled" ("Disabled")) -> ()  [unwired: 2 in, 2 out]
            n1203 = property on="R Scan Velocity SP steps/sec" class="DigNum (strict)"("DisabledEnum"=T9."Disabled and Grayed Out" ("Disabled")) -> ()  [unwired: 2 in, 2 out]
            n1204 = property on="R Scan Length SP steps" class="DigNum (strict)"("DisabledEnum"=T9."Disabled and Grayed Out" ("Disabled")) -> ()  [unwired: 2 in, 2 out]
          }
          frame #5 {
            n1205 = property on="R Scan" class="Bool (strict)"("Val(Sgnl)"=TRUE ("Slew Ready 2")) -> ()  [unwired: 2 in, 2 out]
          }
        }
        n1206 = flat-sequence {
          tunnel: [w2190] -> w2114
          tunnel: [w2189] -> w2113
          tunnel: w2104 -> [w2188]
          tunnel: w2103 -> [w2187]
          tunnel: w2114 -> [w2196]
          tunnel: [w2196] -> w2112
          tunnel: w2113 -> [w2195]
          tunnel: [w2195] -> w2111
          tunnel: w2112 -> [w2200]
          tunnel: [w2199] -> w2110
          tunnel: w2111 -> [w2198]
          tunnel: [w2197] -> w2109
          tunnel: w2110 -> [w2208]
          tunnel: [w2208] -> w2108
          tunnel: w2109 -> [w2207]
          tunnel: [w2207] -> w2107
          tunnel: w2108 -> [w2213]
          tunnel: w2107 -> [w2212]
          tunnel: [w2213] -> w2106
          tunnel: [w2212] -> w2105
          tunnel: [w2215] -> _
          tunnel: [w2216] -> _
          tunnel: w2106 -> [w2216]
          tunnel: w2105 -> [w2215]
          frame #0 {
            n1207 = property on="Y Scan Velocity SP steps/sec" class="DigNum (strict)"() -> ("Value"=w2192:i32)  [unwired: 2 in, 2 out]
            n1208 = Number To Decimal String(number=w2192) -> (decimal integer string=w2193:string)  [unwired: 1 in]
            n1209 = call "mdrive send command.vi"("error in (no error)"=w2188, "Extra"=w2193, "Command"=T10."Max Velocity", "VISA resource name"=w2187) -> ("error out"=w2189:errorcluster, "VISA resource name out"=w2190:refnum<visa-resource-name>)  [unwired: 3 in, 1 out]
          }
          frame #1 {
            n1210 = Wait (ms)(milliseconds to wait=u32 100) -> ()  [unwired: 1 out]
          }
          frame #2 {
            # "VELOCITY"
            n1211 = call "mdrive send command.vi"("error in (no error)"=w2198, "Extra"="VM", "Command"=T10."Print Parameter", "VISA resource name"=w2200) -> ("error out"=w2197:errorcluster, "read buffer"=w2204:string, "VISA resource name out"=w2199:refnum<visa-resource-name>)  [unwired: 3 in]
            n1212 = Decimal String To Number(string=w2204, offset=0) -> (number=w2202:i32)  [unwired: 1 in, 1 out]
            n1213 = property on="Y velocity PV step/sec" class="DigNum (strict)"("Val(Sgnl)"=w2202) -> ()  [unwired: 2 in, 2 out]
          }
          frame #3 {
            n1214 = Wait (ms)(milliseconds to wait=u32 100) -> ()  [unwired: 1 out]
          }
          frame #4 {
            n1215 = property on="Scan Go" class="Bool (strict)"("DisabledEnum"=T9."Enabled" ("Disabled")) -> ()  [unwired: 2 in, 2 out]
            n1216 = property on="Y Scan Velocity SP steps/sec" class="DigNum (strict)"("DisabledEnum"=T9."Disabled and Grayed Out" ("Disabled")) -> ()  [unwired: 2 in, 2 out]
            n1217 = property on="Y Scan Length SP steps" class="DigNum (strict)"("DisabledEnum"=T9."Disabled and Grayed Out" ("Disabled")) -> ()  [unwired: 2 in, 2 out]
          }
          frame #5 {
            n1218 = property on="Y Scan" class="Bool (strict)"("Val(Sgnl)"=TRUE ("Slew Ready 2")) -> ()  [unwired: 2 in, 2 out]
          }
        }
        n1219 = flat-sequence {
          tunnel: [w2218] -> w2118
          tunnel: [w2217] -> w2116
          tunnel: w2124 -> [w2220]
          tunnel: w2123 -> [w2219]
          tunnel: w2118 -> [w2226]
          tunnel: [w2226] -> w2117
          tunnel: w2116 -> [w2225]
          tunnel: [w2225] -> w2115
          tunnel: w2117 -> [w2230]
          tunnel: [w2229] -> w2120
          tunnel: w2115 -> [w2228]
          tunnel: [w2227] -> w2119
          tunnel: w2120 -> [w2238]
          tunnel: [w2238] -> w2122
          tunnel: w2119 -> [w2237]
          tunnel: [w2237] -> w2121
          tunnel: w2122 -> [w2243]
          tunnel: w2121 -> [w2242]
          tunnel: [w2243] -> w2126
          tunnel: [w2242] -> w2125
          tunnel: [w2245] -> _
          tunnel: [w2246] -> _
          tunnel: w2126 -> [w2246]
          tunnel: w2125 -> [w2245]
          frame #0 {
            n1220 = property on="X Scan Velocity SP steps/sec" class="DigNum (strict)"() -> ("Value"=w2222:i32)  [unwired: 2 in, 2 out]
            n1221 = Number To Decimal String(number=w2222) -> (decimal integer string=w2223:string)  [unwired: 1 in]
            n1222 = call "mdrive send command.vi"("error in (no error)"=w2220, "Extra"=w2223, "Command"=T10."Max Velocity", "VISA resource name"=w2219) -> ("error out"=w2217:errorcluster, "VISA resource name out"=w2218:refnum<visa-resource-name>)  [unwired: 3 in, 1 out]
          }
          frame #1 {
            n1223 = Wait (ms)(milliseconds to wait=u32 100) -> ()  [unwired: 1 out]
          }
          frame #2 {
            # "VELOCITY"
            n1224 = call "mdrive send command.vi"("error in (no error)"=w2228, "Extra"="VM", "Command"=T10."Print Parameter", "VISA resource name"=w2230) -> ("error out"=w2227:errorcluster, "read buffer"=w2233:string, "VISA resource name out"=w2229:refnum<visa-resource-name>)  [unwired: 3 in]
            n1225 = Decimal String To Number(string=w2233, offset=0) -> (number=w2231:i32)  [unwired: 1 in, 1 out]
            n1226 = property on="X velocity PV step/sec" class="DigNum (strict)"("Val(Sgnl)"=w2231) -> ()  [unwired: 2 in, 2 out]
          }
          frame #3 {
            n1227 = Wait (ms)(milliseconds to wait=u32 100) -> ()  [unwired: 1 out]
          }
          frame #4 {
            n1228 = property on="Scan Go" class="Bool (strict)"("DisabledEnum"=T9."Enabled" ("Disabled")) -> ()  [unwired: 2 in, 2 out]
            n1229 = property on="X Scan Velocity SP steps/sec" class="DigNum (strict)"("DisabledEnum"=T9."Disabled and Grayed Out" ("Disabled")) -> ()  [unwired: 2 in, 2 out]
            n1230 = property on="X Scan Length SP steps" class="DigNum (strict)"("DisabledEnum"=T9."Disabled and Grayed Out" ("Disabled")) -> ()  [unwired: 2 in, 2 out]
          }
          frame #5 {
            n1231 = property on="X Scan" class="Bool (strict)"("Val(Sgnl)"=TRUE ("Slew Ready 2")) -> ()  [unwired: 2 in, 2 out]
          }
        }
        n1232 = flat-sequence {
          tunnel: [w2160] -> w2102
          tunnel: [w2159] -> w2101
          tunnel: w2092 -> [w2158]
          tunnel: w2091 -> [w2157]
          tunnel: w2102 -> [w2166]
          tunnel: [w2166] -> w2100
          tunnel: w2101 -> [w2165]
          tunnel: [w2165] -> w2099
          tunnel: w2100 -> [w2172]
          tunnel: [w2171] -> w2098
          tunnel: w2099 -> [w2170]
          tunnel: [w2169] -> w2097
          tunnel: w2098 -> [w2178]
          tunnel: [w2178] -> w2096
          tunnel: w2097 -> [w2177]
          tunnel: [w2177] -> w2095
          tunnel: w2096 -> [w2183]
          tunnel: w2095 -> [w2182]
          tunnel: [w2183] -> w2094
          tunnel: [w2182] -> w2093
          tunnel: [w2185] -> _
          tunnel: [w2186] -> _
          tunnel: w2094 -> [w2186]
          tunnel: w2093 -> [w2185]
          frame #0 {
            n1233 = property on="Z Scan Velocity SP steps/sec" class="DigNum (strict)"() -> ("Value"=w2162:i32)  [unwired: 2 in, 2 out]
            n1234 = Number To Decimal String(number=w2162) -> (decimal integer string=w2163:string)  [unwired: 1 in]
            n1235 = call "mdrive send command.vi"("error in (no error)"=w2158, "Extra"=w2163, "Command"=T10."Max Velocity", "VISA resource name"=w2157) -> ("error out"=w2159:errorcluster, "VISA resource name out"=w2160:refnum<visa-resource-name>)  [unwired: 3 in, 1 out]
          }
          frame #1 {
            n1236 = Wait (ms)(milliseconds to wait=u32 100) -> ()  [unwired: 1 out]
          }
          frame #2 {
            # "VELOCITY"
            n1237 = call "mdrive send command.vi"("error in (no error)"=w2170, "Extra"="VM", "Command"=T10."Print Parameter", "VISA resource name"=w2172) -> ("error out"=w2169:errorcluster, "read buffer"=w2173:string, "VISA resource name out"=w2171:refnum<visa-resource-name>)  [unwired: 3 in]
            n1238 = Decimal String To Number(string=w2173, offset=0) -> (number=w2174:i32)  [unwired: 1 in, 1 out]
            n1239 = property on="Z  velocity PV step/sec" class="DigNum (strict)"("Val(Sgnl)"=w2174) -> ()  [unwired: 2 in, 2 out]
          }
          frame #3 {
            n1240 = Wait (ms)(milliseconds to wait=u32 100) -> ()  [unwired: 1 out]
          }
          frame #4 {
            n1241 = property on="Scan Go" class="Bool (strict)"("DisabledEnum"=T9."Enabled" ("Disabled")) -> ()  [unwired: 2 in, 2 out]
            n1242 = property on="Z Scan Velocity SP steps/sec" class="DigNum (strict)"("DisabledEnum"=T9."Disabled and Grayed Out" ("Disabled")) -> ()  [unwired: 2 in, 2 out]
            n1243 = property on="Z Scan Length SP steps" class="DigNum (strict)"("DisabledEnum"=T9."Disabled and Grayed Out" ("Disabled")) -> ()  [unwired: 2 in, 2 out]
          }
          frame #5 {
            n1244 = property on="Z Scan" class="Bool (strict)"("Val(Sgnl)"=TRUE ("Slew Ready 2")) -> ()  [unwired: 2 in, 2 out]
          }
        }
        n1245 = local write "STATUS"("READY TO SCAN" ("STATUS")) -> ()
        n1246 = property on="GO" class="Bool"("DisabledEnum"=T9."Disabled and Grayed Out" ("Disabled")) -> ()  [unwired: 2 in, 2 out]
      }
      event #13 {
        n1247 = event-data() -> ()  [unwired: 1 in, 7 out]
        n1248 = flat-sequence {
          tunnel: [w2271] -> w2259
          tunnel: [w2270] -> w2258
          tunnel: w2252 -> [w2268]
          tunnel: w2250 -> [w2267]
          tunnel: [w2275] -> _
          tunnel: [w2276] -> _
          tunnel: w2259 -> [w2276]
          tunnel: w2258 -> [w2275]
          frame #0 {
            n1249 = call "mDrive Send Command.vi"("error in (no error)"=w2267, "Command"=T10."Stop", "VISA resource name"=w2268) -> ("error out"=w2270:errorcluster, "VISA resource name out"=w2271:refnum<visa-resource-name>)  [unwired: 4 in, 1 out]
          }
          frame #1 {
            n1250 = property on="R Scan" class="Bool (strict)"("Value"=FALSE ("Slew Ready")) -> ()  [unwired: 2 in, 2 out]
            n1251 = property on="R Scan Length SP steps" class="DigNum (strict)"("DisabledEnum"=T9."Enabled" ("Disabled")) -> ()  [unwired: 2 in, 2 out]
            n1252 = property on="R Scan Velocity SP steps/sec" class="DigNum (strict)"("DisabledEnum"=T9."Enabled" ("Disabled")) -> ()  [unwired: 2 in, 2 out]
          }
        }
        n1253 = flat-sequence {
          tunnel: [w2291] -> w2263
          tunnel: [w2290] -> w2262
          tunnel: w2257 -> [w2288]
          tunnel: w2255 -> [w2287]
          tunnel: [w2295] -> _
          tunnel: [w2296] -> _
          tunnel: w2263 -> [w2296]
          tunnel: w2262 -> [w2295]
          frame #0 {
            n1254 = call "mDrive Send Command.vi"("error in (no error)"=w2287, "Command"=T10."Stop", "VISA resource name"=w2288) -> ("error out"=w2290:errorcluster, "VISA resource name out"=w2291:refnum<visa-resource-name>)  [unwired: 4 in, 1 out]
          }
          frame #1 {
            n1255 = property on="X Scan" class="Bool (strict)"("Value"=FALSE ("Slew Ready")) -> ()  [unwired: 2 in, 2 out]
            n1256 = property on="X Scan Velocity SP steps/sec" class="DigNum (strict)"("DisabledEnum"=T9."Enabled" ("Disabled")) -> ()  [unwired: 2 in, 2 out]
            n1257 = property on="X Scan Length SP steps" class="DigNum (strict)"("DisabledEnum"=T9."Enabled" ("Disabled")) -> ()  [unwired: 2 in, 2 out]
          }
        }
        n1258 = flat-sequence {
          tunnel: [w2281] -> w2261
          tunnel: [w2280] -> w2260
          tunnel: w2256 -> [w2278]
          tunnel: w2254 -> [w2277]
          tunnel: [w2285] -> _
          tunnel: [w2286] -> _
          tunnel: w2261 -> [w2286]
          tunnel: w2260 -> [w2285]
          frame #0 {
            n1259 = call "mDrive Send Command.vi"("error in (no error)"=w2277, "Command"=T10."Stop", "VISA resource name"=w2278) -> ("error out"=w2280:errorcluster, "VISA resource name out"=w2281:refnum<visa-resource-name>)  [unwired: 4 in, 1 out]
          }
          frame #1 {
            n1260 = property on="Z Scan" class="Bool (strict)"("Value"=FALSE ("Slew Ready")) -> ()  [unwired: 2 in, 2 out]
            n1261 = property on="Z Scan Velocity SP steps/sec" class="DigNum (strict)"("DisabledEnum"=T9."Enabled" ("Disabled")) -> ()  [unwired: 2 in, 2 out]
            n1262 = property on="Z Scan Length SP steps" class="DigNum (strict)"("DisabledEnum"=T9."Enabled" ("Disabled")) -> ()  [unwired: 2 in, 2 out]
          }
        }
        n1263 = flat-sequence {
          tunnel: [w2301] -> w2265
          tunnel: [w2300] -> w2264
          tunnel: w2253 -> [w2298]
          tunnel: w2251 -> [w2297]
          tunnel: [w2305] -> _
          tunnel: [w2306] -> _
          tunnel: w2265 -> [w2306]
          tunnel: w2264 -> [w2305]
          frame #0 {
            n1264 = call "mDrive Send Command.vi"("error in (no error)"=w2297, "Command"=T10."Stop", "VISA resource name"=w2298) -> ("error out"=w2300:errorcluster, "VISA resource name out"=w2301:refnum<visa-resource-name>)  [unwired: 4 in, 1 out]
          }
          frame #1 {
            n1265 = property on="Y Scan" class="Bool (strict)"("Value"=FALSE ("Slew Ready")) -> ()  [unwired: 2 in, 2 out]
            n1266 = property on="Y Scan Velocity SP steps/sec" class="DigNum (strict)"("DisabledEnum"=T9."Enabled" ("Disabled")) -> ()  [unwired: 2 in, 2 out]
            n1267 = property on="Y Scan Length SP steps" class="DigNum (strict)"("DisabledEnum"=T9."Enabled" ("Disabled")) -> ()  [unwired: 2 in, 2 out]
          }
        }
        n1268 = property on="GO" class="Bool"("DisabledEnum"=T9."Enabled" ("Disabled")) -> ()  [unwired: 2 in, 2 out]
        n1269 = property on="Set Scan \nParameters" class="Bool"("DisabledEnum"=T9."Enabled" ("Disabled")) -> ()  [unwired: 2 in, 2 out]
        n1270 = property on="Send scan parameter" class="Bool"("DisabledEnum"=T9."Enabled" ("Disabled")) -> ()  [unwired: 2 in, 2 out]
        n1271 = property on="Scan Go" class="Bool (strict)"("DisabledEnum"=T9."Disabled and Grayed Out" ("Disabled")) -> ()  [unwired: 2 in, 2 out]
      }
      event #14 {
        w2307 = T9."Disabled and Grayed Out" ("Disabled")
        n1272 = event-data() -> ()  [unwired: 1 in, 7 out]
        n1273 = flat-sequence {
          tunnel: [w2380] -> w2364
          tunnel: [w2378] -> w2357
          tunnel: [w2379] -> w2354
          tunnel: [w2373] -> w2353
          tunnel: [w2377] -> w2352
          tunnel: [w2376] -> w2351
          tunnel: [w2375] -> w2350
          tunnel: [w2374] -> w2349
          tunnel: w2324 -> [w2372]
          tunnel: w2323 -> [w2371]
          tunnel: w2322 -> [w2370]
          tunnel: w2321 -> [w2369]
          tunnel: w2320 -> [w2368]
          tunnel: w2319 -> [w2367]
          tunnel: w2318 -> [w2366]
          tunnel: w2317 -> [w2365]
          tunnel: [w2372] -> w2316
          tunnel: [w2371] -> w2315
          tunnel: [w2370] -> w2314
          tunnel: [w2369] -> w2313
          tunnel: [w2368] -> w2312
          tunnel: [w2367] -> w2311
          tunnel: [w2366] -> w2310
          tunnel: [w2365] -> w2309
          tunnel: [w2432] -> w2361
          tunnel: [w2431] -> w2359
          tunnel: w2364 -> [w2430]
          tunnel: w2357 -> [w2429]
          tunnel: [w2429] -> w2355
          tunnel: w2354 -> [w2428]
          tunnel: w2353 -> [w2417]
          tunnel: w2352 -> [w2427]
          tunnel: w2351 -> [w2423]
          tunnel: w2350 -> [w2420]
          tunnel: w2349 -> [w2426]
          tunnel: [w2425] -> w2347
          tunnel: [w2424] -> w2345
          tunnel: [w2423] -> w2342
          tunnel: [w2422] -> w2340
          tunnel: [w2421] -> w2338
          tunnel: [w2420] -> w2336
          tunnel: [w2419] -> w2334
          tunnel: [w2418] -> w2332
          tunnel: [w2417] -> w2331
          tunnel: w2316 -> [w2416]
          tunnel: w2315 -> [w2415]
          tunnel: w2314 -> [w2414]
          tunnel: w2313 -> [w2413]
          tunnel: w2312 -> [w2412]
          tunnel: w2311 -> [w2411]
          tunnel: w2310 -> [w2410]
          tunnel: w2309 -> [w2409]
          tunnel: w2361 -> [w2473]
          tunnel: [w2473] -> w2360
          tunnel: w2359 -> [w2472]
          tunnel: [w2472] -> w2358
          tunnel: [w2471] -> w2356
          tunnel: w2355 -> [w2471]
          tunnel: [w2470] -> w2348
          tunnel: w2347 -> [w2470]
          tunnel: [w2469] -> w2346
          tunnel: w2345 -> [w2469]
          tunnel: [w2468] -> w2344
          tunnel: [w2467] -> w2343
          tunnel: w2342 -> [w2467]
          tunnel: [w2466] -> w2341
          tunnel: w2340 -> [w2466]
          tunnel: [w2465] -> w2339
          tunnel: w2338 -> [w2465]
          tunnel: [w2464] -> w2337
          tunnel: w2336 -> [w2464]
          tunnel: [w2463] -> w2335
          tunnel: w2334 -> [w2463]
          tunnel: [w2462] -> w2333
          tunnel: w2332 -> [w2462]
          tunnel: w2331 -> [w2468]
          tunnel: w2360 -> [w2493]
          tunnel: [w2491] -> w2363
          tunnel: w2358 -> [w2492]
          tunnel: [w2490] -> w2362
          tunnel: w2356 -> [w2489]
          tunnel: w2348 -> [w2488]
          tunnel: w2346 -> [w2487]
          tunnel: w2344 -> [w2486]
          tunnel: w2343 -> [w2485]
          tunnel: w2341 -> [w2484]
          tunnel: w2339 -> [w2483]
          tunnel: w2337 -> [w2482]
          tunnel: w2335 -> [w2481]
          tunnel: w2333 -> [w2480]
          tunnel: [w2479] -> w2330
          tunnel: [w2478] -> w2329
          tunnel: [w2477] -> w2328
          tunnel: [w2476] -> w2327
          tunnel: [w2475] -> w2326
          tunnel: [w2474] -> w2325
          tunnel: w2363 -> [w2550]
          tunnel: w2362 -> [w2549]
          tunnel: [w2550] -> _
          tunnel: [w2549] -> _
          tunnel: [w2544] -> _
          tunnel: w2330 -> [w2544]
          tunnel: [w2543] -> _
          tunnel: w2329 -> [w2543]
          tunnel: w2328 -> [w2533]
          tunnel: [w2533] -> _
          tunnel: [w2532] -> _
          tunnel: w2327 -> [w2532]
          tunnel: [w2531] -> _
          tunnel: w2326 -> [w2531]
          tunnel: [w2530] -> _
          tunnel: w2325 -> [w2530]
          frame #0 {
            n1274 = property on="X Scan" class="Bool (strict)"() -> ("Value"=w2373:bool)  [unwired: 2 in, 2 out]
            n1275 = property on="Z Scan" class="Bool (strict)"() -> ("Value"=w2375:bool)  [unwired: 2 in, 2 out]
            n1276 = property on="Y Scan" class="Bool (strict)"() -> ("Value"=w2378:bool)  [unwired: 2 in, 2 out]
            n1277 = property on="R Scan" class="Bool (strict)"() -> ("Value"=w2376:bool)  [unwired: 2 in, 2 out]
            n1278 = case shown="False" w2373 {
              tunnel: ["" w2396] -> w2379
              frame #0 {
              }
              frame #1 {
                n1279 = property on="X Scan Length SP steps" class="DigNum (strict)"() -> ("Value"=w2401:i32)  [unwired: 2 in, 2 out]
                n1280 = Number To Decimal String(number=w2401) -> (decimal integer string=w2398:string)  [unwired: 1 in]
                n1281 = call <vilib>:"Space Constant.vi"() -> ("String"=w2399:string)
                n1282 = Concatenate Strings("MR", w2399, w2398, "\r") -> (w2396:string)
              }
            }
            n1283 = case shown="False" w2375 {
              tunnel: ["" w2389] -> w2377
              frame #0 {
              }
              frame #1 {
                n1284 = property on="Z Scan Length SP steps" class="DigNum (strict)"() -> ("Value"=w2394:i32)  [unwired: 2 in, 2 out]
                n1285 = Number To Decimal String(number=w2394) -> (decimal integer string=w2391:string)  [unwired: 1 in]
                n1286 = call <vilib>:"Space Constant.vi"() -> ("String"=w2392:string)
                n1287 = Concatenate Strings("MR", w2392, w2391, "\r") -> (w2389:string)
              }
            }
            n1288 = case shown="False" w2378 {
              tunnel: ["" w2403] -> w2380
              frame #0 {
              }
              frame #1 {
                n1289 = property on="Y Scan Length SP steps" class="DigNum (strict)"() -> ("Value"=w2408:i32)  [unwired: 2 in, 2 out]
                n1290 = Number To Decimal String(number=w2408) -> (decimal integer string=w2405:string)  [unwired: 1 in]
                n1291 = call <vilib>:"Space Constant.vi"() -> ("String"=w2406:string)
                n1292 = Concatenate Strings("MR", w2406, w2405, "\r") -> (w2403:string)
              }
            }
            n1293 = case shown="False" w2376 {
              tunnel: ["" w2382] -> w2374
              frame #0 {
              }
              frame #1 {
                n1294 = property on="R Scan Length SP steps" class="DigNum (strict)"() -> ("Value"=w2387:i32)  [unwired: 2 in, 2 out]
                n1295 = Number To Decimal String(number=w2387) -> (decimal integer string=w2384:string)  [unwired: 1 in]
                n1296 = call <vilib>:"Space Constant.vi"() -> ("String"=w2385:string)
                n1297 = Concatenate Strings("MR", w2385, w2384, "\r") -> (w2382:string)
              }
            }
          }
          frame #1 {
            n1298 = case shown="False" w2417 {
              tunnel: [w2448 w2453] -> w2425
              tunnel: [w2447 w2452] -> w2424
              tunnel: w2428 -> [_ w2451]
              tunnel: w2416 -> [w2448 w2450]
              tunnel: w2415 -> [w2447 w2449]
              frame #0 {
              }
              frame #1 {
                n1299 = VISA Write(VISA resource name=w2450, write buffer=w2451, error in (no error)=w2449) -> (VISA resource name out=w2453:refnum<visa-resource-name>, error out=w2452:errorcluster)  [unwired: 1 out]
              }
            }
            n1300 = case shown="True" w2420 {
              tunnel: [w2441 w2446] -> w2419
              tunnel: [w2440 w2445] -> w2418
              tunnel: w2427 -> [_ w2444]
              tunnel: w2414 -> [w2441 w2443]
              tunnel: w2413 -> [w2440 w2442]
              frame #0 {
              }
              frame #1 {
                n1301 = VISA Write(VISA resource name=w2443, write buffer=w2444, error in (no error)=w2442) -> (VISA resource name out=w2446:refnum<visa-resource-name>, error out=w2445:errorcluster)  [unwired: 1 out]
              }
            }
            n1302 = case shown="True" w2429 {
              tunnel: [w2455 w2460] -> w2432
              tunnel: [w2454 w2459] -> w2431
              tunnel: w2430 -> [_ w2458]
              tunnel: w2412 -> [w2455 w2457]
              tunnel: w2411 -> [w2454 w2456]
              frame #0 {
              }
              frame #1 {
                n1303 = VISA Write(VISA resource name=w2457, write buffer=w2458, error in (no error)=w2456) -> (VISA resource name out=w2460:refnum<visa-resource-name>, error out=w2459:errorcluster)  [unwired: 1 out]
              }
            }
            n1304 = case shown="True" w2423 {
              tunnel: [w2434 w2439] -> w2422
              tunnel: [w2433 w2438] -> w2421
              tunnel: w2426 -> [_ w2437]
              tunnel: w2410 -> [w2434 w2436]
              tunnel: w2409 -> [w2433 w2435]
              frame #0 {
              }
              frame #1 {
                n1305 = VISA Write(VISA resource name=w2436, write buffer=w2437, error in (no error)=w2435) -> (VISA resource name out=w2439:refnum<visa-resource-name>, error out=w2438:errorcluster)  [unwired: 1 out]
              }
            }
          }
          frame #2 {
            n1306 = Wait (ms)(milliseconds to wait=u32 100) -> ()  [unwired: 1 out]
          }
          frame #3 {
            n1307 = case shown="True" w2486 {
              tunnel: w2488 -> [w2513 w2517]
              tunnel: w2487 -> [w2512 w2516]
              tunnel: [w2513 w2515] -> w2475
              tunnel: [w2512 w2514] -> w2474
              frame #0 {
              }
              frame #1 {
                n1308 = property class="Instr"(reference=w2517, error in=w2516) -> (reference out=w2519:refnum<visa-resource-name>, error out=w2518:errorcluster, "Serial Settings:Number of Bytes at Serial Port"=w2520:u32)
                n1309 = VISA Read(VISA resource name=w2519, byte count=w2520, error in (no error)=w2518) -> (VISA resource name out=w2515:refnum<visa-resource-name>, error out=w2514:errorcluster)  [unwired: 2 out]
              }
            }
            n1310 = case shown="True" w2482 {
              tunnel: w2481 -> [w2495 w2499]
              tunnel: w2480 -> [w2494 w2498]
              tunnel: [w2495 w2497] -> w2479
              tunnel: [w2494 w2496] -> w2478
              frame #0 {
              }
              frame #1 {
                n1311 = property class="Instr"(reference=w2499, error in=w2498) -> (reference out=w2501:refnum<visa-resource-name>, error out=w2500:errorcluster, "Serial Settings:Number of Bytes at Serial Port"=w2502:u32)
                n1312 = VISA Read(VISA resource name=w2501, byte count=w2502, error in (no error)=w2500) -> (VISA resource name out=w2497:refnum<visa-resource-name>, error out=w2496:errorcluster)  [unwired: 2 out]
              }
            }
            n1313 = case shown="True" w2489 {
              tunnel: w2493 -> [w2522 w2526]
              tunnel: w2492 -> [w2521 w2525]
              tunnel: [w2522 w2524] -> w2491
              tunnel: [w2521 w2523] -> w2490
              frame #0 {
              }
              frame #1 {
                n1314 = property class="Instr"(reference=w2526, error in=w2525) -> (reference out=w2528:refnum<visa-resource-name>, error out=w2527:errorcluster, "Serial Settings:Number of Bytes at Serial Port"=w2529:u32)
                n1315 = VISA Read(VISA resource name=w2528, byte count=w2529, error in (no error)=w2527) -> (VISA resource name out=w2524:refnum<visa-resource-name>, error out=w2523:errorcluster)  [unwired: 2 out]
              }
            }
            n1316 = case shown="True" w2485 {
              tunnel: w2484 -> [w2504 w2508]
              tunnel: w2483 -> [w2503 w2507]
              tunnel: [w2504 w2506] -> w2477
              tunnel: [w2503 w2505] -> w2476
              frame #0 {
              }
              frame #1 {
                n1317 = property class="Instr"(reference=w2508, error in=w2507) -> (reference out=w2510:refnum<visa-resource-name>, error out=w2509:errorcluster, "Serial Settings:Number of Bytes at Serial Port"=w2511:u32)
                n1318 = VISA Read(VISA resource name=w2510, byte count=w2511, error in (no error)=w2509) -> (VISA resource name out=w2506:refnum<visa-resource-name>, error out=w2505:errorcluster)  [unwired: 2 out]
              }
            }
          }
          frame #4 {
            n1319 = property on="R Scan" class="Bool (strict)"("Val(Sgnl)"=FALSE ("Slew Ready 2")) -> ()  [unwired: 2 in, 2 out]
            n1320 = property on="Z Scan" class="Bool (strict)"("Val(Sgnl)"=FALSE ("Slew Ready 2")) -> ()  [unwired: 2 in, 2 out]
            n1321 = property on="Y Scan" class="Bool (strict)"("Val(Sgnl)"=FALSE ("Slew Ready 2")) -> ()  [unwired: 2 in, 2 out]
            n1322 = property on="X Scan" class="Bool (strict)"("Val(Sgnl)"=FALSE ("Slew Ready 2")) -> ()  [unwired: 2 in, 2 out]
            n1323 = property on="R Scan Length SP steps" class="DigNum (strict)"("DisabledEnum"=T9."Enabled" ("Disabled")) -> ()  [unwired: 2 in, 2 out]
            n1324 = property on="Z Scan Velocity SP steps/sec" class="DigNum (strict)"("DisabledEnum"=T9."Enabled" ("Disabled")) -> ()  [unwired: 2 in, 2 out]
            n1325 = property on="X Scan Length SP steps" class="DigNum (strict)"("DisabledEnum"=T9."Enabled" ("Disabled")) -> ()  [unwired: 2 in, 2 out]
            n1326 = property on="Y Scan Selocity SP steps/sec" class="DigNum (strict)"("DisabledEnum"=T9."Enabled" ("Disabled")) -> ()  [unwired: 2 in, 2 out]
            n1327 = property on="Z Scan Length SP steps" class="DigNum (strict)"("DisabledEnum"=T9."Enabled" ("Disabled")) -> ()  [unwired: 2 in, 2 out]
            n1328 = property on="X Scan Velocity SP steps/sec" class="DigNum (strict)"("DisabledEnum"=T9."Enabled" ("Disabled")) -> ()  [unwired: 2 in, 2 out]
            n1329 = property on="Y Scan Length SP steps" class="DigNum (strict)"("DisabledEnum"=T9."Enabled" ("Disabled")) -> ()  [unwired: 2 in, 2 out]
            n1330 = property on="R Scan Velocity SP steps/sec" class="DigNum (strict)"("DisabledEnum"=T9."Enabled" ("Disabled")) -> ()  [unwired: 2 in, 2 out]
            n1331 = property on="Scan Go" class="Bool (strict)"("DisabledEnum"=T9."Disabled and Grayed Out" ("Disabled")) -> ()  [unwired: 2 in, 2 out]
          }
        }
        n1332 = local write "STATUS"("SCANNING" ("STATUS")) -> ()
        n1333 = property on="GO" class="Bool"("DisabledEnum"=w2307) -> ()  [unwired: 2 in, 2 out]
        n1334 = property on="Set Scan \nParameters" class="Bool"("DisabledEnum"=w2307) -> ()  [unwired: 2 in, 2 out]
        n1335 = property on="Send scan parameter" class="Bool"("DisabledEnum"=w2307) -> ()  [unwired: 2 in, 2 out]
      }
      event #15 {
        n1336 = event-data() -> ()  [unwired: 1 in, 7 out]
        n1337 = flat-sequence {
          tunnel: [w2562] -> _
          tunnel: [w2563] -> _
          tunnel: w2555 -> [w2560]
          tunnel: w2551 -> [w2559]
          frame #0 {
            n1338 = property on="Reset R Motor Steps" class="DigNum (strict)"() -> ("Value"=w2561:i32)  [unwired: 2 in, 2 out]
            n1339 = Number To Decimal String(number=w2561) -> (decimal integer string=w2564:string)  [unwired: 1 in]
            n1340 = call "mDrive Send Command.vi"("error in (no error)"=w2560, "Extra"=w2564, "Command"=T10."Set Current Position", "VISA resource name"=w2559) -> ("error out"=w2563:errorcluster, "VISA resource name out"=w2562:refnum<visa-resource-name>)  [unwired: 3 in, 1 out]
          }
        }
        n1341 = flat-sequence {
          tunnel: [w2582] -> _
          tunnel: [w2583] -> _
          tunnel: w2558 -> [w2581]
          tunnel: w2554 -> [w2580]
          frame #0 {
            n1342 = property on="Reset X Motor Steps" class="DigNum (strict)"() -> ("Value"=w2584:i32)  [unwired: 2 in, 2 out]
            n1343 = Number To Decimal String(number=w2584) -> (decimal integer string=w2585:string)  [unwired: 1 in]
            n1344 = call "mDrive Send Command.vi"("error in (no error)"=w2581, "Extra"=w2585, "Command"=T10."Set Current Position", "VISA resource name"=w2580) -> ("error out"=w2583:errorcluster, "VISA resource name out"=w2582:refnum<visa-resource-name>)  [unwired: 3 in, 1 out]
          }
        }
        n1345 = flat-sequence {
          tunnel: [w2576] -> _
          tunnel: [w2577] -> _
          tunnel: w2557 -> [w2574]
          tunnel: w2553 -> [w2573]
          frame #0 {
            n1346 = property on="Reset Z Motor Steps" class="DigNum (strict)"() -> ("Value"=w2575:i32)  [unwired: 2 in, 2 out]
            n1347 = Number To Decimal String(number=w2575) -> (decimal integer string=w2578:string)  [unwired: 1 in]
            n1348 = call "mDrive Send Command.vi"("error in (no error)"=w2574, "Extra"=w2578, "Command"=T10."Set Current Position", "VISA resource name"=w2573) -> ("error out"=w2577:errorcluster, "VISA resource name out"=w2576:refnum<visa-resource-name>)  [unwired: 3 in, 1 out]
          }
        }
        n1349 = flat-sequence {
          tunnel: [w2569] -> _
          tunnel: [w2570] -> _
          tunnel: w2556 -> [w2567]
          tunnel: w2552 -> [w2566]
          frame #0 {
            n1350 = property on="Reset Y Motor Steps" class="DigNum (strict)"() -> ("Value"=w2568:i32)  [unwired: 2 in, 2 out]
            n1351 = Number To Decimal String(number=w2568) -> (decimal integer string=w2571:string)  [unwired: 1 in]
            n1352 = call "mDrive Send Command.vi"("error in (no error)"=w2567, "Extra"=w2571, "Command"=T10."Set Current Position", "VISA resource name"=w2566) -> ("error out"=w2570:errorcluster, "VISA resource name out"=w2569:refnum<visa-resource-name>)  [unwired: 3 in, 1 out]
          }
        }
      }
      event #16 {
        n1353 = event-data() -> ()  [unwired: 1 in, 7 out]
        n1354 = flat-sequence {
          tunnel: w2606 -> [w4192]
          tunnel: [w4192] -> w2605
          tunnel: w2604 -> [w4191]
          tunnel: [w4191] -> w2603
          tunnel: w2602 -> [w4190]
          tunnel: [w4190] -> w2601
          tunnel: w2600 -> [w4189]
          tunnel: [w4189] -> w2599
          tunnel: w2598 -> [w4188]
          tunnel: [w4188] -> w2597
          tunnel: w2596 -> [w4187]
          tunnel: [w4187] -> w2595
          tunnel: w2594 -> [w4186]
          tunnel: [w4186] -> w2593
          tunnel: w2592 -> [w4185]
          tunnel: [w4185] -> w2591
          frame #0 {
            w4193 = T9."Disabled and Grayed Out" ("Disabled")
            n1355 = local write "STATUS"("ENTERING LOOP" ("STATUS")) -> ()
            n1356 = property on="Z Scan Length SP steps" class="DigNum (strict)"("DisabledEnum"=T9."Disabled and Grayed Out" ("Disabled")) -> ()  [unwired: 2 in, 2 out]
            n1357 = property on="Z Scan Velocity SP steps/sec" class="DigNum (strict)"("DisabledEnum"=T9."Disabled and Grayed Out" ("Disabled")) -> ()  [unwired: 2 in, 2 out]
            n1358 = property on="GO" class="Bool"("DisabledEnum"=w4193) -> ()  [unwired: 2 in, 2 out]
            n1359 = property on="Set Scan \nParameters" class="Bool"("DisabledEnum"=w4193) -> ()  [unwired: 2 in, 2 out]
            n1360 = property on="Scan Go" class="Bool (strict)"("DisabledEnum"=w4193) -> ()  [unwired: 2 in, 2 out]
            n1361 = property on="Send scan parameter" class="Bool"("DisabledEnum"=w4193) -> ()  [unwired: 2 in, 2 out]
            n1362 = property on="R Scan Length SP steps" class="DigNum (strict)"("DisabledEnum"=T9."Disabled and Grayed Out" ("Disabled")) -> ()  [unwired: 2 in, 2 out]
            n1363 = property on="R Scan Velocity SP steps/sec" class="DigNum (strict)"("DisabledEnum"=T9."Disabled and Grayed Out" ("Disabled")) -> ()  [unwired: 2 in, 2 out]
            n1364 = property on="Y Scan Length SP steps" class="DigNum (strict)"("DisabledEnum"=T9."Disabled and Grayed Out" ("Disabled")) -> ()  [unwired: 2 in, 2 out]
            n1365 = property on="Y Scan Velocity SP steps/sec" class="DigNum (strict)"("DisabledEnum"=T9."Disabled and Grayed Out" ("Disabled")) -> ()  [unwired: 2 in, 2 out]
            n1366 = property on="X Scan Length SP steps" class="DigNum (strict)"("DisabledEnum"=T9."Disabled and Grayed Out" ("Disabled")) -> ()  [unwired: 2 in, 2 out]
            n1367 = property on="X Scan Velocity SP steps/sec" class="DigNum (strict)"("DisabledEnum"=T9."Disabled and Grayed Out" ("Disabled")) -> ()  [unwired: 2 in, 2 out]
          }
        }
        n1368 = while {
          tunnel: w2601 -> [w2663]
          tunnel: w2597 -> [w2662]
          tunnel: w2599 -> [w2661]
          tunnel: w2595 -> [w2660]
          tunnel: w2593 -> [w2659]
          tunnel: w2591 -> [w2658]
          tunnel: w2603 -> [w2657]
          tunnel: w2605 -> [w2656]
          tunnel: [w2655] -> w2590 mode=indexing
          tunnel: [w2654] -> w2589 mode=indexing
          tunnel: [w2653] -> w2588 mode=indexing
          tunnel: [w2652] -> w2587 mode=indexing
          i -> [w2618]
          stop <- w2607 stop-if-true
          # "XZYR"
          n1369 = flat-sequence {
            tunnel: w2662 -> [w2691]
            tunnel: w2663 -> [w2692]
            tunnel: [w2688] -> w2679
            tunnel: [w2681] -> w2678
            tunnel: [w2687] -> w2677
            tunnel: [w2686] -> w2676
            tunnel: [w2685] -> w2675
            tunnel: [w2684] -> w2674
            tunnel: [w2680] -> w2673
            tunnel: [w2683] -> w2672
            tunnel: w2661 -> [w2696]
            tunnel: w2660 -> [w2695]
            tunnel: w2659 -> [w2694]
            tunnel: w2658 -> [w2693]
            tunnel: w2657 -> [w2690]
            tunnel: w2656 -> [w2689]
            tunnel: [w2826] -> w2635
            tunnel: [w2825] -> w2633
            tunnel: [w2824] -> w2631
            tunnel: [w2823] -> w2629
            tunnel: [w2821] -> w2627
            tunnel: [w2820] -> w2625
            tunnel: [w2822] -> w2623
            tunnel: w2679 -> [w2819]
            tunnel: w2678 -> [w2818]
            tunnel: w2677 -> [w2817]
            tunnel: w2676 -> [w2816]
            tunnel: w2675 -> [w2815]
            tunnel: w2674 -> [w2814]
            tunnel: w2673 -> [w2813]
            tunnel: w2672 -> [w2812]
            tunnel: [w2811] -> w2621
            tunnel: w2635 -> [w2951]
            tunnel: [w2951] -> w2634
            tunnel: w2633 -> [w2950]
            tunnel: [w2950] -> w2632
            tunnel: w2631 -> [w2949]
            tunnel: [w2949] -> w2630
            tunnel: w2629 -> [w2948]
            tunnel: [w2948] -> w2628
            tunnel: w2627 -> [w2947]
            tunnel: [w2947] -> w2626
            tunnel: w2625 -> [w2946]
            tunnel: [w2946] -> w2624
            tunnel: w2623 -> [w2945]
            tunnel: [w2945] -> w2622
            tunnel: w2621 -> [w2944]
            tunnel: [w2944] -> w2620
            tunnel: [w2966] -> w2651
            tunnel: [w2964] -> w2649
            tunnel: [w2957] -> w2647
            tunnel: [w2956] -> w2645
            tunnel: [w2955] -> w2643
            tunnel: [w2954] -> w2641
            tunnel: [w2953] -> w2639
            tunnel: [w2952] -> w2637
            tunnel: w2634 -> [w2967]
            tunnel: w2632 -> [w2965]
            tunnel: w2630 -> [w2962]
            tunnel: w2628 -> [w2961]
            tunnel: w2626 -> [w2959]
            tunnel: w2624 -> [w2958]
            tunnel: w2622 -> [w2960]
            tunnel: w2620 -> [w2963]
            tunnel: w2651 -> [w3246]
            tunnel: [w3246] -> w2650
            tunnel: w2649 -> [w3245]
            tunnel: [w3245] -> w2648
            tunnel: w2647 -> [w3244]
            tunnel: [w3244] -> w2646
            tunnel: w2645 -> [w3243]
            tunnel: [w3243] -> w2644
            tunnel: w2643 -> [w3242]
            tunnel: [w3242] -> w2642
            tunnel: w2641 -> [w3241]
            tunnel: [w3241] -> w2640
            tunnel: w2639 -> [w3240]
            tunnel: [w3240] -> w2638
            tunnel: w2637 -> [w3239]
            tunnel: [w3239] -> w2636
            tunnel: w2650 -> [w3264]
            tunnel: w2648 -> [w3262]
            tunnel: w2646 -> [w3263]
            tunnel: w2644 -> [w3261]
            tunnel: w2642 -> [w3260]
            tunnel: w2640 -> [w3259]
            tunnel: w2638 -> [w3258]
            tunnel: w2636 -> [w3257]
            tunnel: [w3256] -> w2671
            tunnel: [w3255] -> w2670
            tunnel: [w3254] -> w2669
            tunnel: [w3253] -> w2668
            tunnel: [w3252] -> w2667
            tunnel: [w3251] -> w2666
            tunnel: [w3250] -> w2665
            tunnel: [w3249] -> w2664
            tunnel: w2671 -> [w3557]
            tunnel: w2670 -> [w3558]
            tunnel: w2669 -> [w3560]
            tunnel: w2668 -> [w3559]
            tunnel: w2667 -> [w3563]
            tunnel: w2666 -> [w3564]
            tunnel: w2665 -> [w3561]
            tunnel: w2664 -> [w3562]
            tunnel: [w3566] -> w2617
            tunnel: [w3565] -> w2616
            tunnel: [w3567] -> w2615
            tunnel: [w3568] -> w2614
            tunnel: [w3571] -> w2613
            tunnel: [w3572] -> w2612
            tunnel: [w3569] -> w2611
            tunnel: [w3570] -> w2610
            tunnel: [w4164] -> _
            tunnel: [w4165] -> w2655
            tunnel: [w4166] -> _
            tunnel: [w4167] -> w2654
            tunnel: [w4168] -> _
            tunnel: [w4169] -> w2652
            tunnel: [w4170] -> w2653
            tunnel: [w4171] -> _
            tunnel: w2617 -> [w4171]
            tunnel: w2616 -> [w4170]
            tunnel: w2615 -> [w4169]
            tunnel: w2614 -> [w4168]
            tunnel: w2613 -> [w4167]
            tunnel: w2612 -> [w4166]
            tunnel: w2611 -> [w4165]
            tunnel: w2610 -> [w4164]
            frame #0 {
              n1370 = flat-sequence {
                tunnel: [w2788] -> w2720
                tunnel: [w2787] -> w2719
                tunnel: w2691 -> [w2790]
                tunnel: w2692 -> [w2789]
                tunnel: w2720 -> [w2796]
                tunnel: [w2796] -> w2718
                tunnel: w2719 -> [w2795]
                tunnel: [w2795] -> w2717
                tunnel: w2718 -> [w2800]
                tunnel: [w2799] -> w2716
                tunnel: w2717 -> [w2798]
                tunnel: [w2797] -> w2715
                tunnel: w2716 -> [w2808]
                tunnel: w2715 -> [w2806]
                tunnel: [w2808] -> w2688
                tunnel: [w2806] -> w2681
                frame #0 {
                  n1371 = property on="X Scan Velocity SP steps/sec" class="DigNum (strict)"() -> ("Value"=w2792:i32)  [unwired: 2 in, 2 out]
                  n1372 = Number To Decimal String(number=w2792) -> (decimal integer string=w2793:string)  [unwired: 1 in]
                  n1373 = call "mDrive Send Command.vi"("error in (no error)"=w2790, "Extra"=w2793, "Command"=T10."Max Velocity", "VISA resource name"=w2789) -> ("error out"=w2787:errorcluster, "VISA resource name out"=w2788:refnum<visa-resource-name>)  [unwired: 3 in, 1 out]
                }
                frame #1 {
                  n1374 = Wait (ms)(milliseconds to wait=u32 100) -> ()  [unwired: 1 out]
                }
                frame #2 {
                  # "VELOCITY"
                  n1375 = call "mDrive Send Command.vi"("error in (no error)"=w2798, "Extra"="VM", "Command"=T10."Print Parameter", "VISA resource name"=w2800) -> ("error out"=w2797:errorcluster, "read buffer"=w2803:string, "VISA resource name out"=w2799:refnum<visa-resource-name>)  [unwired: 3 in]
                  n1376 = Decimal String To Number(string=w2803, offset=0) -> (number=w2801:i32)  [unwired: 1 in, 1 out]
                  n1377 = property on="X velocity PV step/sec" class="DigNum (strict)"("Val(Sgnl)"=w2801) -> ()  [unwired: 2 in, 2 out]
                }
                frame #3 {
                  n1378 = Wait (ms)(milliseconds to wait=u32 100) -> ()  [unwired: 1 out]
                }
              }
              n1379 = flat-sequence {
                tunnel: [w2746] -> w2708
                tunnel: [w2745] -> w2707
                tunnel: w2695 -> [w2744]
                tunnel: w2696 -> [w2743]
                tunnel: w2708 -> [w2752]
                tunnel: [w2752] -> w2706
                tunnel: w2707 -> [w2751]
                tunnel: [w2751] -> w2705
                tunnel: w2706 -> [w2758]
                tunnel: [w2757] -> w2704
                tunnel: w2705 -> [w2756]
                tunnel: [w2755] -> w2703
                tunnel: w2704 -> [w2764]
                tunnel: w2703 -> [w2763]
                tunnel: [w2764] -> w2687
                tunnel: [w2763] -> w2686
                frame #0 {
                  n1380 = property on="Z Scan Velocity SP steps/sec" class="DigNum (strict)"() -> ("Value"=w2748:i32)  [unwired: 2 in, 2 out]
                  n1381 = Number To Decimal String(number=w2748) -> (decimal integer string=w2749:string)  [unwired: 1 in]
                  n1382 = call "mDrive Send Command.vi"("error in (no error)"=w2744, "Extra"=w2749, "Command"=T10."Max Velocity", "VISA resource name"=w2743) -> ("error out"=w2745:errorcluster, "VISA resource name out"=w2746:refnum<visa-resource-name>)  [unwired: 3 in, 1 out]
                }
                frame #1 {
                  n1383 = Wait (ms)(milliseconds to wait=u32 100) -> ()  [unwired: 1 out]
                }
                frame #2 {
                  # "VELOCITY"
                  n1384 = call "mDrive Send Command.vi"("error in (no error)"=w2756, "Extra"="VM", "Command"=T10."Print Parameter", "VISA resource name"=w2758) -> ("error out"=w2755:errorcluster, "read buffer"=w2759:string, "VISA resource name out"=w2757:refnum<visa-resource-name>)  [unwired: 3 in]
                  n1385 = Decimal String To Number(string=w2759, offset=0) -> (number=w2760:i32)  [unwired: 1 in, 1 out]
                  n1386 = property on="Z  velocity PV step/sec" class="DigNum (strict)"("Val(Sgnl)"=w2760) -> ()  [unwired: 2 in, 2 out]
                }
                frame #3 {
                  n1387 = Wait (ms)(milliseconds to wait=u32 100) -> ()  [unwired: 1 out]
                }
              }
              n1388 = flat-sequence {
                tunnel: [w2768] -> w2714
                tunnel: [w2767] -> w2713
                tunnel: w2693 -> [w2766]
                tunnel: w2694 -> [w2765]
                tunnel: w2714 -> [w2774]
                tunnel: [w2774] -> w2712
                tunnel: w2713 -> [w2773]
                tunnel: [w2773] -> w2711
                tunnel: w2712 -> [w2778]
                tunnel: [w2777] -> w2710
                tunnel: w2711 -> [w2776]
                tunnel: [w2775] -> w2709
                tunnel: w2710 -> [w2786]
                tunnel: w2709 -> [w2785]
                tunnel: [w2786] -> w2685
                tunnel: [w2785] -> w2684
                frame #0 {
                  n1389 = property on="Y Scan Velocity SP steps/sec" class="DigNum (strict)"() -> ("Value"=w2770:i32)  [unwired: 2 in, 2 out]
                  n1390 = Number To Decimal String(number=w2770) -> (decimal integer string=w2771:string)  [unwired: 1 in]
                  n1391 = call "mDrive Send Command.vi"("error in (no error)"=w2766, "Extra"=w2771, "Command"=T10."Max Velocity", "VISA resource name"=w2765) -> ("error out"=w2767:errorcluster, "VISA resource name out"=w2768:refnum<visa-resource-name>)  [unwired: 3 in, 1 out]
                }
                frame #1 {
                  n1392 = Wait (ms)(milliseconds to wait=u32 100) -> ()  [unwired: 1 out]
                }
                frame #2 {
                  # "VELOCITY"
                  n1393 = call "mDrive Send Command.vi"("error in (no error)"=w2776, "Extra"="VM", "Command"=T10."Print Parameter", "VISA resource name"=w2778) -> ("error out"=w2775:errorcluster, "read buffer"=w2782:string, "VISA resource name out"=w2777:refnum<visa-resource-name>)  [unwired: 3 in]
                  n1394 = Decimal String To Number(string=w2782, offset=0) -> (number=w2780:i32)  [unwired: 1 in, 1 out]
                  n1395 = property on="Y velocity PV step/sec" class="DigNum (strict)"("Val(Sgnl)"=w2780) -> ()  [unwired: 2 in, 2 out]
                }
                frame #3 {
                  n1396 = Wait (ms)(milliseconds to wait=u32 100) -> ()  [unwired: 1 out]
                }
              }
              n1397 = flat-sequence {
                tunnel: [w2724] -> w2702
                tunnel: [w2723] -> w2701
                tunnel: w2690 -> [w2722]
                tunnel: w2689 -> [w2721]
                tunnel: w2702 -> [w2730]
                tunnel: [w2730] -> w2700
                tunnel: w2701 -> [w2729]
                tunnel: [w2729] -> w2699
                tunnel: w2700 -> [w2736]
                tunnel: [w2735] -> w2698
                tunnel: w2699 -> [w2734]
                tunnel: [w2733] -> w2697
                tunnel: w2698 -> [w2740]
                tunnel: w2697 -> [w2742]
                tunnel: [w2742] -> w2683
                tunnel: [w2740] -> w2680
                frame #0 {
                  n1398 = property on="R Scan Velocity SP steps/sec" class="DigNum (strict)"() -> ("Value"=w2726:i32)  [unwired: 2 in, 2 out]
                  n1399 = Number To Decimal String(number=w2726) -> (decimal integer string=w2727:string)  [unwired: 1 in]
                  n1400 = call "mDrive Send Command.vi"("error in (no error)"=w2722, "Extra"=w2727, "Command"=T10."Max Velocity", "VISA resource name"=w2721) -> ("error out"=w2723:errorcluster, "VISA resource name out"=w2724:refnum<visa-resource-name>)  [unwired: 3 in, 1 out]
                }
                frame #1 {
                  n1401 = Wait (ms)(milliseconds to wait=u32 100) -> ()  [unwired: 1 out]
                }
                frame #2 {
                  # "VELOCITY"
                  n1402 = call "mDrive Send Command.vi"("error in (no error)"=w2734, "Extra"="VM", "Command"=T10."Print Parameter", "VISA resource name"=w2736) -> ("error out"=w2733:errorcluster, "read buffer"=w2738:string, "VISA resource name out"=w2735:refnum<visa-resource-name>)  [unwired: 3 in]
                  n1403 = Decimal String To Number(string=w2738, offset=0) -> (number=w2737:i32)  [unwired: 1 in, 1 out]
                  n1404 = property on="R velocity PV step/sec" class="DigNum (strict)"("Val(Sgnl)"=w2737) -> ()  [unwired: 2 in, 2 out]
                }
                frame #3 {
                  n1405 = Wait (ms)(milliseconds to wait=u32 100) -> ()  [unwired: 1 out]
                }
              }
              n1406 = local write "STATUS"("LOOP INITIALIZING" ("STATUS")) -> ()
            }
            frame #1 {
              w2809 = TRUE ("R in Motion")
              n1407 = flat-sequence {
                tunnel: [w2886] -> w2854
                tunnel: [w2885] -> w2853
                tunnel: [w2884] -> w2852
                tunnel: [w2883] -> w2851
                tunnel: w2819 -> [w2882]
                tunnel: w2818 -> [w2881]
                tunnel: w2817 -> [w2880]
                tunnel: w2816 -> [w2879]
                tunnel: w2815 -> [w2878]
                tunnel: w2814 -> [w2877]
                tunnel: w2813 -> [w2876]
                tunnel: w2812 -> [w2875]
                tunnel: [w2882] -> w2850
                tunnel: [w2881] -> w2849
                tunnel: [w2880] -> w2848
                tunnel: [w2879] -> w2847
                tunnel: [w2878] -> w2846
                tunnel: [w2877] -> w2845
                tunnel: [w2876] -> w2844
                tunnel: [w2875] -> w2843
                tunnel: [w2906] -> w2842
                tunnel: [w2905] -> w2841
                tunnel: w2854 -> [w2904]
                tunnel: w2853 -> [w2903]
                tunnel: w2852 -> [w2902]
                tunnel: w2851 -> [w2901]
                tunnel: [w2900] -> w2840
                tunnel: [w2899] -> w2839
                tunnel: [w2898] -> w2838
                tunnel: [w2897] -> w2837
                tunnel: [w2896] -> w2836
                tunnel: [w2895] -> w2835
                tunnel: w2850 -> [w2894]
                tunnel: w2849 -> [w2893]
                tunnel: w2848 -> [w2892]
                tunnel: w2847 -> [w2891]
                tunnel: w2846 -> [w2890]
                tunnel: w2845 -> [w2889]
                tunnel: w2844 -> [w2888]
                tunnel: w2843 -> [w2887]
                tunnel: w2842 -> [w2915]
                tunnel: [w2915] -> w2834
                tunnel: w2841 -> [w2914]
                tunnel: [w2914] -> w2833
                tunnel: [w2913] -> w2832
                tunnel: w2840 -> [w2913]
                tunnel: [w2912] -> w2831
                tunnel: w2839 -> [w2912]
                tunnel: [w2911] -> w2830
                tunnel: w2838 -> [w2911]
                tunnel: [w2910] -> w2829
                tunnel: w2837 -> [w2910]
                tunnel: [w2909] -> w2828
                tunnel: w2836 -> [w2909]
                tunnel: [w2908] -> w2827
                tunnel: w2835 -> [w2908]
                tunnel: w2834 -> [w2943]
                tunnel: w2833 -> [w2942]
                tunnel: w2832 -> [w2939]
                tunnel: w2831 -> [w2938]
                tunnel: w2830 -> [w2937]
                tunnel: w2829 -> [w2936]
                tunnel: w2828 -> [w2935]
                tunnel: w2827 -> [w2934]
                tunnel: [w2941] -> w2823
                tunnel: [w2940] -> w2822
                tunnel: [w2933] -> w2824
                tunnel: [w2932] -> w2821
                tunnel: [w2931] -> w2820
                tunnel: [w2930] -> w2826
                tunnel: [w2929] -> w2825
                tunnel: [w2916] -> w2811
                frame #0 {
                  n1408 = property on="X Scan Length SP steps" class="DigNum (strict)"() -> ("Value"=w2869:i32)  [unwired: 2 in, 2 out]
                  n1409 = property on="Z Scan Length SP steps" class="DigNum (strict)"() -> ("Value"=w2874:i32)  [unwired: 2 in, 2 out]
                  n1410 = property on="Y Scan Length SP steps" class="DigNum (strict)"() -> ("Value"=w2864:i32)  [unwired: 2 in, 2 out]
                  n1411 = property on="R Scan Length SP steps" class="DigNum (strict)"() -> ("Value"=w2859:i32)  [unwired: 2 in, 2 out]
                  n1412 = Number To Decimal String(number=w2869) -> (decimal integer string=w2866:string)  [unwired: 1 in]
                  n1413 = Number To Decimal String(number=w2874) -> (decimal integer string=w2871:string)  [unwired: 1 in]
                  n1414 = Number To Decimal String(number=w2864) -> (decimal integer string=w2861:string)  [unwired: 1 in]
                  n1415 = Number To Decimal String(number=w2859) -> (decimal integer string=w2856:string)  [unwired: 1 in]
                  n1416 = call <vilib>:"Space Constant.vi"() -> ("String"=w2867:string)
                  n1417 = call <vilib>:"Space Constant.vi"() -> ("String"=w2872:string)
                  n1418 = call <vilib>:"Space Constant.vi"() -> ("String"=w2862:string)
                  n1419 = call <vilib>:"Space Constant.vi"() -> ("String"=w2857:string)
                  n1420 = Concatenate Strings("MR", w2867, w2866, "\r") -> (w2885:string)
                  n1421 = Concatenate Strings("MR", w2872, w2871, "\r") -> (w2884:string)
                  n1422 = Concatenate Strings("MR", w2862, w2861, "\r") -> (w2886:string)
                  n1423 = Concatenate Strings("MR", w2857, w2856, "\r") -> (w2883:string)
                }
                frame #1 {
                  n1424 = VISA Write(VISA resource name=w2894, write buffer=w2903, error in (no error)=w2893) -> (VISA resource name out=w2900:refnum<visa-resource-name>, error out=w2899:errorcluster)  [unwired: 1 out]
                  n1425 = VISA Write(VISA resource name=w2892, write buffer=w2902, error in (no error)=w2891) -> (VISA resource name out=w2896:refnum<visa-resource-name>, error out=w2895:errorcluster)  [unwired: 1 out]
                  n1426 = VISA Write(VISA resource name=w2890, write buffer=w2904, error in (no error)=w2889) -> (VISA resource name out=w2906:refnum<visa-resource-name>, error out=w2905:errorcluster)  [unwired: 1 out]
                  n1427 = VISA Write(VISA resource name=w2888, write buffer=w2901, error in (no error)=w2887) -> (VISA resource name out=w2898:refnum<visa-resource-name>, error out=w2897:errorcluster)  [unwired: 1 out]
                }
                frame #2 {
                  n1428 = Wait (ms)(milliseconds to wait=u32 100) -> ()  [unwired: 1 out]
                }
                frame #3 {
                  n1429 = property class="Instr"(reference=w2939, error in=w2938) -> (reference out=w2921:refnum<visa-resource-name>, error out=w2920:errorcluster, "Serial Settings:Number of Bytes at Serial Port"=w2922:u32)
                  n1430 = property class="Instr"(reference=w2935, error in=w2934) -> (reference out=w2918:refnum<visa-resource-name>, error out=w2917:errorcluster, "Serial Settings:Number of Bytes at Serial Port"=w2919:u32)
                  n1431 = property class="Instr"(reference=w2943, error in=w2942) -> (reference out=w2924:refnum<visa-resource-name>, error out=w2923:errorcluster, "Serial Settings:Number of Bytes at Serial Port"=w2925:u32)
                  n1432 = property class="Instr"(reference=w2937, error in=w2936) -> (reference out=w2927:refnum<visa-resource-name>, error out=w2926:errorcluster, "Serial Settings:Number of Bytes at Serial Port"=w2928:u32)
                  n1433 = VISA Read(VISA resource name=w2921, byte count=w2922, error in (no error)=w2920) -> (VISA resource name out=w2930:refnum<visa-resource-name>, error out=w2929:errorcluster)  [unwired: 2 out]
                  n1434 = VISA Read(VISA resource name=w2918, byte count=w2919, error in (no error)=w2917) -> (VISA resource name out=w2916:refnum<visa-resource-name>, error out=w2933:errorcluster)  [unwired: 2 out]
                  n1435 = VISA Read(VISA resource name=w2924, byte count=w2925, error in (no error)=w2923) -> (VISA resource name out=w2941:refnum<visa-resource-name>, error out=w2940:errorcluster)  [unwired: 2 out]
                  n1436 = VISA Read(VISA resource name=w2927, byte count=w2928, error in (no error)=w2926) -> (VISA resource name out=w2932:refnum<visa-resource-name>, error out=w2931:errorcluster)  [unwired: 2 out]
                }
              }
              n1437 = local write "STATUS"("LOOP SCANNING" ("STATUS")) -> ()
              n1438 = property on="Y in Motion" class="Bool (strict)"("Value"=w2809) -> ()  [unwired: 2 in, 2 out]
              n1439 = property on="Z in Motion" class="Bool (strict)"("Value"=w2809) -> ()  [unwired: 2 in, 2 out]
              n1440 = property on="X  in Motion" class="Bool (strict)"("Value"=w2809) -> ()  [unwired: 2 in, 2 out]
              n1441 = property on="R in Motion" class="Bool (strict)"("Value"=w2809) -> ()  [unwired: 2 in, 2 out]
            }
            frame #2 {
            }
            frame #3 {
              n1442 = while {
                tunnel: w2967 -> [w2989]
                tunnel: [w2977] -> w2966
                tunnel: w2965 -> [w2988]
                tunnel: [w2976] -> w2964
                tunnel: w2963 -> [w2987]
                tunnel: w2962 -> [w2986]
                tunnel: w2961 -> [w2985]
                tunnel: w2960 -> [w2984]
                tunnel: w2959 -> [w2983]
                tunnel: w2958 -> [w2982]
                tunnel: [w2979] -> w2957
                tunnel: [w2978] -> w2956
                tunnel: [w2975] -> w2955
                tunnel: [w2974] -> w2954
                tunnel: [w2973] -> w2953
                tunnel: [w2972] -> w2952
                stop <- w2968 stop-if-true
                n1443 = flat-sequence {
                  tunnel: [w3190] -> w3025
                  tunnel: [w3189] -> w3024
                  tunnel: [w3188] -> w3023
                  tunnel: w2989 -> [w3187]
                  tunnel: w2988 -> [w3186]
                  tunnel: [w3212] -> w3022
                  tunnel: [w3211] -> w3021
                  tunnel: [w3209] -> w3020
                  tunnel: w3025 -> [w3209]
                  tunnel: w3024 -> [w3208]
                  tunnel: w3023 -> [w3207]
                  tunnel: w3022 -> [w3225]
                  tunnel: [w3225] -> w3017
                  tunnel: w3021 -> [w3224]
                  tunnel: [w3224] -> w3018
                  tunnel: w3020 -> [w3223]
                  tunnel: [w3223] -> w3019
                  tunnel: w3019 -> [w3228]
                  tunnel: w3018 -> [w3230]
                  tunnel: w3017 -> [w3229]
                  tunnel: [w3227] -> w2977
                  tunnel: [w3226] -> w2976
                  frame #0 {
                    n1444 = property on="X Step SP" class="DigNum (strict)"() -> ("Maximum"=w3202:dbl)  [unwired: 2 in, 2 out]
                    n1445 = property on="X Step SP" class="DigNum (strict)"() -> ("Minimum"=w3204:dbl)  [unwired: 2 in, 2 out]
                    n1446 = property on="X steps/rev" class="DigNum (strict)"() -> ("Value"=w3199:u32)  [unwired: 2 in, 2 out]
                    n1447 = property on="X offset mm" class="DigNum (strict)"() -> ("Value"=w3195:dbl)  [unwired: 2 in, 2 out]
                    n1448 = To Long Integer(number=w3202) -> (32bit integer=w3201:i32)
                    n1449 = To Long Integer(number=w3204) -> (32bit integer=w3203:i32)
                    n1450 = To Double Precision Float(number=w3199) -> (double precision float=w3200:dbl)
                    n1451 = call "mDrive Send Command.vi"("error in (no error)"=w3186, "Extra"="P", "Command"=T10."Print Parameter", "VISA resource name"=w3187) -> ("error out"=w3188:errorcluster, "read buffer"=w3206:string, "VISA resource name out"=w3189:refnum<visa-resource-name>)  [unwired: 3 in]
                    n1452 = Decimal String To Number(string=w3206, offset=0) -> (number=w3185:i32)  [unwired: 1 in, 1 out]
                    n1453 = property on="X Step PV" class="DigNum (strict)"("Val(Sgnl)"=w3185) -> ()  [unwired: 2 in, 2 out]
                    n1454 = In Range and Coerce(upper limit=w3201, x=w3185, lower limit=w3203) -> (In Range?=w3190:bool)  [unwired: 1 out]
                    n1455 = To Double Precision Float(number=w3185) -> (double precision float=w3194:dbl)
                    n1456 = property on="X  in Range" class="Bool (strict)"("Val(Sgnl)"=w3190) -> ()  [unwired: 2 in, 2 out]
                    n1457 = Divide(x=w3194, y=w3200) -> (x/y=w3198:dbl)
                    n1458 = property on="X mm/rev" class="DigNum (strict)"() -> ("Value"=w3197:dbl)  [unwired: 2 in, 2 out]
                    n1459 = Multiply(x=w3198, y=w3197) -> (x*y=w3196:dbl)
                    n1460 = Add(x=w3196, y=w3195) -> (x+y=w3193:dbl)
                    n1461 = property on="X Position mm PV" class="DigNum (strict)"("Val(Sgnl)"=w3193) -> ()  [unwired: 2 in, 2 out]
                  }
                  frame #1 {
                    n1462 = call "mDrive Send Command.vi"("error in (no error)"=w3207, "Extra"="MV", "Command"=T10."Print Parameter", "VISA resource name"=w3208) -> ("error out"=w3211:errorcluster, "read buffer"=w3215:string, "VISA resource name out"=w3212:refnum<visa-resource-name>)  [unwired: 3 in]
                    n1463 = Decimal String To Number(string=w3215, offset=0 ("offset (0)")) -> (number=w3218:i32)  [unwired: 1 in, 1 out]
                    n1464 = Not Equal?(x=w3215, y="") -> (x != y?=w3213:bool)
                    n1465 = property on="X Ready" class="Bool (strict)"("Val(Sgnl)"=w3213) -> ()  [unwired: 2 in, 2 out]
                    n1466 = Number To Boolean Array(number=w3218) -> (Boolean array=w3217:bool[])
                    n1467 = Index Array(array=w3217, index=0) -> (element=w3210:bool)
                    n1468 = property on="X  in Motion" class="Bool (strict)"("Val(Sgnl)"=w3210) -> ()  [unwired: 2 in, 2 out]
                  }
                  frame #2 {
                    n1469 = Wait (ms)(milliseconds to wait=u32 10) -> ()  [unwired: 1 out]
                  }
                  frame #3 {
                    n1470 = case shown="False" w3228 {
                      tunnel: w3229 -> [w3233 w3237]
                      tunnel: [w3234 w3237] -> w3227
                      tunnel: [w3235 w3236] -> w3226
                      tunnel: w3230 -> [w3232 w3236]
                      frame #0 {
                        n1471 = call "mDrive Send Command.vi"("error in (no error)"=w3232, "Command"=T10."Stop", "VISA resource name"=w3233) -> ("error out"=w3235:errorcluster, "VISA resource name out"=w3234:refnum<visa-resource-name>)  [unwired: 4 in, 1 out]
                      }
                      frame #1 {
                      }
                    }
                  }
                }
                n1472 = flat-sequence {
                  tunnel: [w3143] -> w3016
                  tunnel: [w3134] -> w3015
                  tunnel: [w3133] -> w3014
                  tunnel: w2987 -> [w3137]
                  tunnel: w2986 -> [w3136]
                  tunnel: [w3163] -> w3013
                  tunnel: [w3162] -> w3012
                  tunnel: [w3161] -> w3011
                  tunnel: w3016 -> [w3161]
                  tunnel: w3015 -> [w3160]
                  tunnel: w3014 -> [w3159]
                  tunnel: w3013 -> [w3172]
                  tunnel: [w3172] -> w3008
                  tunnel: w3012 -> [w3171]
                  tunnel: [w3171] -> w3009
                  tunnel: w3011 -> [w3170]
                  tunnel: [w3170] -> w3010
                  tunnel: w3010 -> [w3175]
                  tunnel: w3009 -> [w3177]
                  tunnel: w3008 -> [w3176]
                  tunnel: [w3174] -> w2979
                  tunnel: [w3173] -> w2978
                  frame #0 {
                    n1473 = property on="Z Step SP" class="DigNum (strict)"() -> ("Maximum"=w3144:dbl)  [unwired: 2 in, 2 out]
                    n1474 = property on="Z Step SP" class="DigNum (strict)"() -> ("Minimum"=w3138:dbl)  [unwired: 2 in, 2 out]
                    n1475 = property on="Z steps/rev" class="DigNum (strict)"() -> ("Value"=w3142:u32)  [unwired: 2 in, 2 out]
                    n1476 = property on="Z offset mm" class="DigNum (strict)"() -> ("Value"=w3140:dbl)  [unwired: 2 in, 2 out]
                    n1477 = To Long Integer(number=w3144) -> (32bit integer=w3150:i32)
                    n1478 = To Long Integer(number=w3138) -> (32bit integer=w3151:i32)
                    n1479 = To Double Precision Float(number=w3142) -> (double precision float=w3149:dbl)
                    n1480 = call "mDrive Send Command.vi"("error in (no error)"=w3136, "Extra"="P", "Command"=T10."Print Parameter", "VISA resource name"=w3137) -> ("error out"=w3133:errorcluster, "read buffer"=w3153:string, "VISA resource name out"=w3134:refnum<visa-resource-name>)  [unwired: 3 in]
                    n1481 = Decimal String To Number(string=w3153, offset=0) -> (number=w3132:i32)  [unwired: 1 in, 1 out]
                    n1482 = property on="Z Step PV" class="DigNum (strict)"("Val(Sgnl)"=w3132) -> ()  [unwired: 2 in, 2 out]
                    n1483 = In Range and Coerce(upper limit=w3150, x=w3132, lower limit=w3151) -> (In Range?=w3143:bool)  [unwired: 1 out]
                    n1484 = To Double Precision Float(number=w3132) -> (double precision float=w3147:dbl)
                    n1485 = property on="Z in Range" class="Bool (strict)"("Val(Sgnl)"=w3143) -> ()  [unwired: 2 in, 2 out]
                    n1486 = Divide(x=w3147, y=w3149) -> (x/y=w3148:dbl)
                    n1487 = property on="Z mm/rev" class="DigNum (strict)"() -> ("Value"=w3141:dbl)  [unwired: 2 in, 2 out]
                    n1488 = Multiply(x=w3148, y=w3141) -> (x*y=w3135:dbl)
                    n1489 = Add(x=w3135, y=w3140) -> (x+y=w3139:dbl)
                    n1490 = property on="Z Position mm PV" class="DigNum (strict)"("Val(Sgnl)"=w3139) -> ()  [unwired: 2 in, 2 out]
                  }
                  frame #1 {
                    n1491 = call "mDrive Send Command.vi"("error in (no error)"=w3159, "Extra"="MV", "Command"=T10."Print Parameter", "VISA resource name"=w3160) -> ("error out"=w3162:errorcluster, "read buffer"=w3165:string, "VISA resource name out"=w3163:refnum<visa-resource-name>)  [unwired: 3 in]
                    n1492 = Decimal String To Number(string=w3165, offset=0 ("offset (0)")) -> (number=w3155:i32)  [unwired: 1 in, 1 out]
                    n1493 = Not Equal?(x=w3165, y="") -> (x != y?=w3158:bool)
                    n1494 = property on="Z Ready" class="Bool (strict)"("Val(Sgnl)"=w3158) -> ()  [unwired: 2 in, 2 out]
                    n1495 = Number To Boolean Array(number=w3155) -> (Boolean array=w3157:bool[])
                    n1496 = Index Array(array=w3157, index=0) -> (element=w3154:bool)
                    n1497 = property on="Z in Motion" class="Bool (strict)"("Val(Sgnl)"=w3154) -> ()  [unwired: 2 in, 2 out]
                  }
                  frame #2 {
                    n1498 = Wait (ms)(milliseconds to wait=u32 10) -> ()  [unwired: 1 out]
                  }
                  frame #3 {
                    n1499 = case shown="False" w3175 {
                      tunnel: w3176 -> [w3180 w3184]
                      tunnel: [w3181 w3184] -> w3174
                      tunnel: [w3182 w3183] -> w3173
                      tunnel: w3177 -> [w3179 w3183]
                      frame #0 {
                        n1500 = call "mDrive Send Command.vi"("error in (no error)"=w3179, "Command"=T10."Stop", "VISA resource name"=w3180) -> ("error out"=w3182:errorcluster, "VISA resource name out"=w3181:refnum<visa-resource-name>)  [unwired: 4 in, 1 out]
                      }
                      frame #1 {
                      }
                    }
                  }
                }
                n1501 = flat-sequence {
                  tunnel: [w3088] -> w3007
                  tunnel: [w3090] -> w3006
                  tunnel: [w3089] -> w3005
                  tunnel: w2985 -> [w3081]
                  tunnel: w2984 -> [w3080]
                  tunnel: [w3110] -> w3004
                  tunnel: [w3109] -> w3003
                  tunnel: [w3108] -> w3002
                  tunnel: w3007 -> [w3108]
                  tunnel: w3006 -> [w3107]
                  tunnel: w3005 -> [w3106]
                  tunnel: w3004 -> [w3119]
                  tunnel: [w3119] -> w2999
                  tunnel: w3003 -> [w3118]
                  tunnel: [w3118] -> w3000
                  tunnel: w3002 -> [w3117]
                  tunnel: [w3117] -> w3001
                  tunnel: w3001 -> [w3122]
                  tunnel: w3000 -> [w3124]
                  tunnel: w2999 -> [w3123]
                  tunnel: [w3120] -> w2975
                  tunnel: [w3121] -> w2974
                  frame #0 {
                    n1502 = property on="Y Step SP" class="DigNum (strict)"() -> ("Maximum"=w3083:dbl)  [unwired: 2 in, 2 out]
                    n1503 = property on="Y Step SP" class="DigNum (strict)"() -> ("Minimum"=w3082:dbl)  [unwired: 2 in, 2 out]
                    n1504 = property on="Y steps/rev" class="DigNum (strict)"() -> ("Value"=w3084:u32)  [unwired: 2 in, 2 out]
                    n1505 = property on="Y offset mm" class="DigNum (strict)"() -> ("Value"=w3086:dbl)  [unwired: 2 in, 2 out]
                    n1506 = To Long Integer(number=w3083) -> (32bit integer=w3097:i32)
                    n1507 = To Long Integer(number=w3082) -> (32bit integer=w3098:i32)
                    n1508 = To Double Precision Float(number=w3084) -> (double precision float=w3096:dbl)
                    n1509 = call "mDrive Send Command.vi"("error in (no error)"=w3080, "Extra"="P", "Command"=T10."Print Parameter", "VISA resource name"=w3081) -> ("error out"=w3089:errorcluster, "read buffer"=w3100:string, "VISA resource name out"=w3090:refnum<visa-resource-name>)  [unwired: 3 in]
                    n1510 = Decimal String To Number(string=w3100, offset=0) -> (number=w3079:i32)  [unwired: 1 in, 1 out]
                    n1511 = property on="Y Step PV" class="DigNum (strict)"("Val(Sgnl)"=w3079) -> ()  [unwired: 2 in, 2 out]
                    n1512 = In Range and Coerce(upper limit=w3097, x=w3079, lower limit=w3098) -> (In Range?=w3088:bool)  [unwired: 1 out]
                    n1513 = To Double Precision Float(number=w3079) -> (double precision float=w3093:dbl)
                    n1514 = property on="Y in Range" class="Bool (strict)"("Val(Sgnl)"=w3088) -> ()  [unwired: 2 in, 2 out]
                    n1515 = Divide(x=w3093, y=w3096) -> (x/y=w3095:dbl)
                    n1516 = property on="Y mm/rev" class="DigNum (strict)"() -> ("Value"=w3085:dbl)  [unwired: 2 in, 2 out]
                    n1517 = Multiply(x=w3095, y=w3085) -> (x*y=w3094:dbl)
                    n1518 = Add(x=w3094, y=w3086) -> (x+y=w3087:dbl)
                    n1519 = property on="Y Position mm PV" class="DigNum (strict)"("Val(Sgnl)"=w3087) -> ()  [unwired: 2 in, 2 out]
                  }
                  frame #1 {
                    n1520 = call "mDrive Send Command.vi"("error in (no error)"=w3106, "Extra"="MV", "Command"=T10."Print Parameter", "VISA resource name"=w3107) -> ("error out"=w3109:errorcluster, "read buffer"=w3112:string, "VISA resource name out"=w3110:refnum<visa-resource-name>)  [unwired: 3 in]
                    n1521 = Decimal String To Number(string=w3112, offset=0 ("offset (0)")) -> (number=w3102:i32)  [unwired: 1 in, 1 out]
                    n1522 = Not Equal?(x=w3112, y="") -> (x != y?=w3105:bool)
                    n1523 = property on="Y Ready" class="Bool (strict)"("Val(Sgnl)"=w3105) -> ()  [unwired: 2 in, 2 out]
                    n1524 = Number To Boolean Array(number=w3102) -> (Boolean array=w3104:bool[])
                    n1525 = Index Array(array=w3104, index=0) -> (element=w3101:bool)
                    n1526 = property on="Y in Motion" class="Bool (strict)"("Val(Sgnl)"=w3101) -> ()  [unwired: 2 in, 2 out]
                  }
                  frame #2 {
                    n1527 = Wait (ms)(milliseconds to wait=u32 10) -> ()  [unwired: 1 out]
                  }
                  frame #3 {
                    n1528 = case shown="False" w3122 {
                      tunnel: w3123 -> [w3127 w3130]
                      tunnel: [w3128 w3130] -> w3120
                      tunnel: [w3129 w3131] -> w3121
                      tunnel: w3124 -> [w3126 w3131]
                      frame #0 {
                        n1529 = call "mDrive Send Command.vi"("error in (no error)"=w3126, "Command"=T10."Stop", "VISA resource name"=w3127) -> ("error out"=w3129:errorcluster, "VISA resource name out"=w3128:refnum<visa-resource-name>)  [unwired: 4 in, 1 out]
                      }
                      frame #1 {
                      }
                    }
                  }
                }
                n1530 = flat-sequence {
                  tunnel: [w3035] -> w2998
                  tunnel: [w3037] -> w2997
                  tunnel: [w3036] -> w2996
                  tunnel: w2983 -> [w3028]
                  tunnel: w2982 -> [w3027]
                  tunnel: [w3057] -> w2995
                  tunnel: [w3056] -> w2994
                  tunnel: [w3055] -> w2993
                  tunnel: w2998 -> [w3055]
                  tunnel: w2997 -> [w3054]
                  tunnel: w2996 -> [w3053]
                  tunnel: w2995 -> [w3066]
                  tunnel: [w3066] -> w2990
                  tunnel: w2994 -> [w3065]
                  tunnel: [w3065] -> w2991
                  tunnel: w2993 -> [w3064]
                  tunnel: [w3064] -> w2992
                  tunnel: w2992 -> [w3069]
                  tunnel: w2991 -> [w3071]
                  tunnel: w2990 -> [w3070]
                  tunnel: [w3068] -> w2973
                  tunnel: [w3067] -> w2972
                  frame #0 {
                    n1531 = property on="R Step SP" class="DigNum (strict)"() -> ("Maximum"=w3030:dbl)  [unwired: 2 in, 2 out]
                    n1532 = property on="R Step SP" class="DigNum (strict)"() -> ("Minimum"=w3031:dbl)  [unwired: 2 in, 2 out]
                    n1533 = property on="R steps/rev" class="DigNum (strict)"() -> ("Value"=w3029:u32)  [unwired: 2 in, 2 out]
                    n1534 = property on="R offset deg" class="DigNum (strict)"() -> ("Value"=w3033:dbl)  [unwired: 2 in, 2 out]
                    n1535 = To Long Integer(number=w3030) -> (32bit integer=w3044:i32)
                    n1536 = To Long Integer(number=w3031) -> (32bit integer=w3045:i32)
                    n1537 = To Double Precision Float(number=w3029) -> (double precision float=w3043:dbl)
                    n1538 = call "mDrive Send Command.vi"("error in (no error)"=w3027, "Extra"="P", "Command"=T10."Print Parameter", "VISA resource name"=w3028) -> ("error out"=w3036:errorcluster, "read buffer"=w3047:string, "VISA resource name out"=w3037:refnum<visa-resource-name>)  [unwired: 3 in]
                    n1539 = Decimal String To Number(string=w3047, offset=0) -> (number=w3026:i32)  [unwired: 1 in, 1 out]
                    n1540 = property on="R Step PV" class="DigNum (strict)"("Val(Sgnl)"=w3026) -> ()  [unwired: 2 in, 2 out]
                    n1541 = In Range and Coerce(upper limit=w3044, x=w3026, lower limit=w3045) -> (In Range?=w3035:bool)  [unwired: 1 out]
                    n1542 = To Double Precision Float(number=w3026) -> (double precision float=w3040:dbl)
                    n1543 = property on="R in Range" class="Bool (strict)"("Val(Sgnl)"=w3035) -> ()  [unwired: 2 in, 2 out]
                    n1544 = Divide(x=w3040, y=w3043) -> (x/y=w3042:dbl)
                    n1545 = property on="R deg/rev" class="DigNum (strict)"() -> ("Value"=w3032:dbl)  [unwired: 2 in, 2 out]
                    n1546 = Multiply(x=w3042, y=w3032) -> (x*y=w3041:dbl)
                    n1547 = Add(x=w3041, y=w3033) -> (x+y=w3034:dbl)
                    n1548 = property on="R Position deg PV" class="DigNum (strict)"("Val(Sgnl)"=w3034) -> ()  [unwired: 2 in, 2 out]
                  }
                  frame #1 {
                    n1549 = call "mDrive Send Command.vi"("error in (no error)"=w3053, "Extra"="MV", "Command"=T10."Print Parameter", "VISA resource name"=w3054) -> ("error out"=w3056:errorcluster, "read buffer"=w3059:string, "VISA resource name out"=w3057:refnum<visa-resource-name>)  [unwired: 3 in]
                    n1550 = Decimal String To Number(string=w3059, offset=0 ("offset (0)")) -> (number=w3049:i32)  [unwired: 1 in, 1 out]
                    n1551 = Not Equal?(x=w3059, y="") -> (x != y?=w3052:bool)
                    n1552 = property on="R Ready" class="Bool (strict)"("Val(Sgnl)"=w3052) -> ()  [unwired: 2 in, 2 out]
                    n1553 = Number To Boolean Array(number=w3049) -> (Boolean array=w3051:bool[])
                    n1554 = Index Array(array=w3051, index=0) -> (element=w3048:bool)
                    n1555 = property on="R in Motion" class="Bool (strict)"("Val(Sgnl)"=w3048) -> ()  [unwired: 2 in, 2 out]
                  }
                  frame #2 {
                    n1556 = Wait (ms)(milliseconds to wait=u32 10) -> ()  [unwired: 1 out]
                  }
                  frame #3 {
                    n1557 = case shown="False" w3069 {
                      tunnel: w3070 -> [w3074 w3078]
                      tunnel: [w3075 w3078] -> w3068
                      tunnel: [w3076 w3077] -> w3067
                      tunnel: w3071 -> [w3073 w3077]
                      frame #0 {
                        n1558 = call "mDrive Send Command.vi"("error in (no error)"=w3073, "Command"=T10."Stop", "VISA resource name"=w3074) -> ("error out"=w3076:errorcluster, "VISA resource name out"=w3075:refnum<visa-resource-name>)  [unwired: 4 in, 1 out]
                      }
                      frame #1 {
                      }
                    }
                  }
                }
                n1559 = property on="Y in Motion" class="Bool (strict)"() -> ("Value"=w2981:bool)  [unwired: 2 in, 2 out]
                n1560 = property on="Z in Motion" class="Bool (strict)"() -> ("Value"=w2971:bool)  [unwired: 2 in, 2 out]
                n1561 = property on="X  in Motion" class="Bool (strict)"() -> ("Value"=w2980:bool)  [unwired: 2 in, 2 out]
                n1562 = property on="R in Motion" class="Bool (strict)"() -> ("Value"=w2970:bool)  [unwired: 2 in, 2 out]
                n1563 = Compound Arithmetic op=OR(w2980, w2981, w2971, w2970) -> (w2969:bool)
                n1564 = Not(x=w2969) -> (.not. x?=w2968:bool)
              }
            }
            frame #4 {
              n1565 = Wait (ms)(milliseconds to wait=u32 300) -> ()  [unwired: 1 out]
            }
            frame #5 {
              w3247 = TRUE ("R in Motion")
              n1566 = property on="X Position mm PV" class="DigNum (strict)"() -> ("Value"=w3276:dbl)  [unwired: 2 in, 2 out]
              n1567 = property on="X Position SP mm" class="DigNum (strict)"() -> ("Value"=w3275:dbl)  [unwired: 2 in, 2 out]
              n1568 = property on="Z Position mm PV" class="DigNum (strict)"() -> ("Value"=w3272:dbl)  [unwired: 2 in, 2 out]
              n1569 = property on="Z Position SP mm" class="DigNum (strict)"() -> ("Value"=w3265:dbl)  [unwired: 2 in, 2 out]
              n1570 = property on="Y Position mm PV" class="DigNum (strict)"() -> ("Value"=w3270:dbl)  [unwired: 2 in, 2 out]
              n1571 = property on="Y Position SP mm" class="DigNum (strict)"() -> ("Value"=w3269:dbl)  [unwired: 2 in, 2 out]
              n1572 = property on="R Position SP deg" class="DigNum (strict)"() -> ("Value"=w3267:dbl)  [unwired: 2 in, 2 out]
              n1573 = property on="R Position deg PV" class="DigNum (strict)"() -> ("Value"=w3266:dbl)  [unwired: 2 in, 2 out]
              n1574 = Not Equal?(x=w3276, y=w3275) -> (x != y?=w3274:bool)
              n1575 = Not Equal?(x=w3272, y=w3265) -> (x != y?=w3273:bool)
              n1576 = Not Equal?(x=w3270, y=w3269) -> (x != y?=w3271:bool)
              n1577 = Not Equal?(x=w3267, y=w3266) -> (x != y?=w3268:bool)
              n1578 = local write "STATUS"("LOOP HOMING" ("STATUS")) -> ()
              n1579 = case shown="True" w3274 {
                tunnel: w3264 -> [w3488 w3492]
                tunnel: w3262 -> [w3487 w3491]
                tunnel: [w3488 w3490] -> w3249
                tunnel: [w3487 w3489] -> w3250
                frame #0 {
                }
                frame #1 {
                  n1580 = flat-sequence {
                    tunnel: w3491 -> [w3507]
                    tunnel: w3492 -> [w3520]
                    tunnel: [w3520] -> w3506
                    tunnel: [w3507] -> w3505
                    tunnel: [w3509] -> w3504
                    tunnel: [w3523] -> w3503
                    tunnel: [w3522] -> w3502
                    tunnel: [w3521] -> w3501
                    tunnel: w3504 -> [w3521]
                    tunnel: w3505 -> [w3522]
                    tunnel: w3506 -> [w3523]
                    tunnel: [w3539] -> w3500
                    tunnel: [w3538] -> w3499
                    tunnel: w3503 -> [w3537]
                    tunnel: w3502 -> [w3536]
                    tunnel: w3501 -> [w3535]
                    tunnel: [w3535] -> w3498
                    tunnel: w3500 -> [w3546]
                    tunnel: [w3546] -> w3497
                    tunnel: w3499 -> [w3545]
                    tunnel: [w3545] -> w3496
                    tunnel: [w3543] -> w3495
                    tunnel: w3498 -> [w3543]
                    tunnel: [w3551] -> w3494
                    tunnel: [w3550] -> w3493
                    tunnel: w3497 -> [w3549]
                    tunnel: w3496 -> [w3548]
                    tunnel: w3495 -> [w3547]
                    tunnel: [w3555] -> w3489
                    tunnel: [w3556] -> w3490
                    tunnel: w3494 -> [w3556]
                    tunnel: w3493 -> [w3555]
                    frame #0 {
                      n1581 = property on="X steps/rev" class="DigNum (strict)"() -> ("Value"=w3519:u32)  [unwired: 2 in, 2 out]
                      n1582 = To Double Precision Float(number=w3519) -> (double precision float=w3514:dbl)
                      n1583 = property on="X offset mm" class="DigNum (strict)"() -> ("Value"=w3518:dbl)  [unwired: 2 in, 2 out]
                      n1584 = property on="X Position SP mm" class="DigNum (strict)"() -> ("Value"=w3517:dbl)  [unwired: 2 in, 2 out]
                      n1585 = Subtract(x=w3517, y=w3518) -> (x-y=w3511:dbl)
                      n1586 = property on="X mm/rev" class="DigNum (strict)"() -> ("Value"=w3508:dbl)  [unwired: 2 in, 2 out]
                      n1587 = Divide(x=w3511, y=w3508) -> (x/y=w3510:dbl)
                      n1588 = property on="X Step SP" class="DigNum (strict)"() -> ("Maximum"=w3516:dbl)  [unwired: 2 in, 2 out]
                      n1589 = property on="X Step SP" class="DigNum (strict)"() -> ("Minimum"=w3515:dbl)  [unwired: 2 in, 2 out]
                      n1590 = Multiply(x=w3510, y=w3514) -> (x*y=w3512:dbl)
                      n1591 = In Range and Coerce(upper limit=w3516, x=w3512, lower limit=w3515) -> (coerced(x)=w3513:dbl)  [unwired: 1 out]
                      n1592 = To Long Integer(number=w3513) -> (32bit integer=w3509:i32)
                      n1593 = property on="X Step SP" class="DigNum (strict)"("Val(Sgnl)"=w3509) -> ()  [unwired: 2 in, 2 out]
                    }
                    frame #1 {
                      n1594 = property on="X Step SP" class="DigNum (strict)"() -> ("Value"=w3532:i32)  [unwired: 2 in, 2 out]
                      n1595 = property on="X Step PV" class="DigNum (strict)"() -> ("Value"=w3531:i32)  [unwired: 2 in, 2 out]
                      n1596 = property on="X Backlash" class="DigNum (strict)"() -> ("Value"=w3524:i32)  [unwired: 2 in, 2 out]
                      n1597 = Subtract(x=w3532, y=w3531) -> (x-y=w3530:i32)
                      n1598 = Sign(1:w3524) -> (0:w3528:i32)
                      n1599 = Sign(1:w3530) -> (0:w3529:i32)
                      n1600 = Multiply(x=w3529, y=w3528) -> (x*y=w3527:i32)
                      n1601 = Equal?(x=w3527, y=1) -> (x = y?=w3525:bool)
                      n1602 = case shown="True" w3525 {
                        frame #0 {
                          n1603 = property on="X Backlash corr" class="Bool (strict)"("Val(Sgnl)"=FALSE ("Value (Signaling)")) -> ()  [unwired: 2 in, 2 out]
                        }
                        frame #1 {
                          n1604 = property on="X Backlash corr" class="Bool (strict)"("Val(Sgnl)"=TRUE ("Value (Signaling)")) -> ()  [unwired: 2 in, 2 out]
                        }
                      }
                    }
                    frame #2 {
                      # "Velocity Setting"
                      n1605 = property on="X Velocity SP step/sec" class="DigNum (strict)"() -> ("Value"=w3540:i32)  [unwired: 2 in, 2 out]
                      n1606 = Number To Decimal String(number=w3540) -> (decimal integer string=w3541:string)  [unwired: 1 in]
                      n1607 = call "mDrive Send Command.vi"("error in (no error)"=w3536, "Extra"=w3541, "Command"=T10."Max Velocity", "VISA resource name"=w3537) -> ("error out"=w3538:errorcluster, "VISA resource name out"=w3539:refnum<visa-resource-name>)  [unwired: 3 in, 1 out]
                    }
                    frame #3 {
                      n1608 = Wait (ms)(milliseconds to wait=u32 50) -> ()  [unwired: 1 out]
                    }
                    frame #4 {
                      # "Move to Abs Position"
                      n1609 = Number To Decimal String(number=w3547) -> (decimal integer string=w3553:string)  [unwired: 1 in]
                      n1610 = call "mDrive Send Command.vi"("error in (no error)"=w3548, "Extra"=w3553, "Command"=T10."Move to Absolute Position", "VISA resource name"=w3549) -> ("error out"=w3550:errorcluster, "VISA resource name out"=w3551:refnum<visa-resource-name>)  [unwired: 3 in, 1 out]
                    }
                    frame #5 {
                      n1611 = Wait (ms)(milliseconds to wait=u32 50) -> ()  [unwired: 1 out]
                    }
                  }
                }
              }
              n1612 = case shown="True" w3273 {
                tunnel: w3261 -> [w3417 w3422]
                tunnel: w3263 -> [w3418 w3421]
                tunnel: [w3418 w3420] -> w3251
                tunnel: [w3417 w3419] -> w3252
                frame #0 {
                }
                frame #1 {
                  n1613 = flat-sequence {
                    tunnel: [w3450] -> w3436
                    tunnel: [w3449] -> w3435
                    tunnel: [w3438] -> w3434
                    tunnel: w3422 -> [w3450]
                    tunnel: w3421 -> [w3449]
                    tunnel: [w3453] -> w3433
                    tunnel: [w3452] -> w3432
                    tunnel: [w3451] -> w3431
                    tunnel: w3434 -> [w3451]
                    tunnel: w3435 -> [w3452]
                    tunnel: w3436 -> [w3453]
                    tunnel: [w3469] -> w3430
                    tunnel: [w3468] -> w3429
                    tunnel: w3433 -> [w3467]
                    tunnel: w3432 -> [w3466]
                    tunnel: [w3465] -> w3428
                    tunnel: w3431 -> [w3465]
                    tunnel: w3430 -> [w3476]
                    tunnel: [w3476] -> w3427
                    tunnel: w3429 -> [w3475]
                    tunnel: [w3475] -> w3426
                    tunnel: w3428 -> [w3474]
                    tunnel: [w3474] -> w3425
                    tunnel: [w3481] -> w3424
                    tunnel: [w3480] -> w3423
                    tunnel: w3427 -> [w3479]
                    tunnel: w3426 -> [w3478]
                    tunnel: w3425 -> [w3477]
                    tunnel: [w3485] -> w3419
                    tunnel: [w3486] -> w3420
                    tunnel: w3424 -> [w3486]
                    tunnel: w3423 -> [w3485]
                    frame #0 {
                      n1614 = property on="Z steps/rev" class="DigNum (strict)"() -> ("Value"=w3437:u32)  [unwired: 2 in, 2 out]
                      n1615 = To Double Precision Float(number=w3437) -> (double precision float=w3443:dbl)
                      n1616 = property on="Z offset mm" class="DigNum (strict)"() -> ("Value"=w3445:dbl)  [unwired: 2 in, 2 out]
                      n1617 = property on="Z Position SP mm" class="DigNum (strict)"() -> ("Value"=w3444:dbl)  [unwired: 2 in, 2 out]
                      n1618 = Subtract(x=w3444, y=w3445) -> (x-y=w3440:dbl)
                      n1619 = property on="Z mm/rev" class="DigNum (strict)"() -> ("Value"=w3446:dbl)  [unwired: 2 in, 2 out]
                      n1620 = Divide(x=w3440, y=w3446) -> (x/y=w3439:dbl)
                      n1621 = property on="Z Step SP" class="DigNum (strict)"() -> ("Maximum"=w3448:dbl)  [unwired: 2 in, 2 out]
                      n1622 = property on="Z Step SP" class="DigNum (strict)"() -> ("Minimum"=w3447:dbl)  [unwired: 2 in, 2 out]
                      n1623 = Multiply(x=w3439, y=w3443) -> (x*y=w3441:dbl)
                      n1624 = In Range and Coerce(upper limit=w3448, x=w3441, lower limit=w3447) -> (coerced(x)=w3442:dbl)  [unwired: 1 out]
                      n1625 = To Long Integer(number=w3442) -> (32bit integer=w3438:i32)
                      n1626 = property on="Z Step SP" class="DigNum (strict)"("Val(Sgnl)"=w3438) -> ()  [unwired: 2 in, 2 out]
                    }
                    frame #1 {
                      n1627 = property on="Z Step SP" class="DigNum (strict)"() -> ("Value"=w3462:i32)  [unwired: 2 in, 2 out]
                      n1628 = property on="Z Backlash" class="DigNum (strict)"() -> ("Value"=w3454:i32)  [unwired: 2 in, 2 out]
                      n1629 = property on="Z Step PV" class="DigNum (strict)"() -> ("Value"=w3461:i32)  [unwired: 2 in, 2 out]
                      n1630 = Subtract(x=w3462, y=w3461) -> (x-y=w3460:i32)
                      n1631 = Sign(1:w3454) -> (0:w3458:i32)
                      n1632 = Sign(1:w3460) -> (0:w3459:i32)
                      n1633 = Multiply(x=w3459, y=w3458) -> (x*y=w3457:i32)
                      n1634 = Equal?(x=w3457, y=1) -> (x = y?=w3455:bool)
                      n1635 = case shown="False" w3455 {
                        frame #0 {
                          n1636 = property on="Z Backlash corr" class="Bool (strict)"("Val(Sgnl)"=FALSE ("Value (Signaling)")) -> ()  [unwired: 2 in, 2 out]
                        }
                        frame #1 {
                          n1637 = property on="Z Backlash corr" class="Bool (strict)"("Val(Sgnl)"=TRUE ("Value (Signaling)")) -> ()  [unwired: 2 in, 2 out]
                        }
                      }
                    }
                    frame #2 {
                      # "Velocity Setting"
                      n1638 = property on="Z Velocity SP step/sec" class="DigNum (strict)"() -> ("Value"=w3470:i32)  [unwired: 2 in, 2 out]
                      n1639 = Number To Decimal String(number=w3470) -> (decimal integer string=w3471:string)  [unwired: 1 in]
                      n1640 = call "mDrive Send Command.vi"("error in (no error)"=w3467, "Extra"=w3471, "Command"=T10."Max Velocity", "VISA resource name"=w3466) -> ("error out"=w3468:errorcluster, "VISA resource name out"=w3469:refnum<visa-resource-name>)  [unwired: 3 in, 1 out]
                    }
                    frame #3 {
                      n1641 = Wait (ms)(milliseconds to wait=u32 50) -> ()  [unwired: 1 out]
                    }
                    frame #4 {
                      # "Move to Abs Position"
                      n1642 = Number To Decimal String(number=w3477) -> (decimal integer string=w3483:string)  [unwired: 1 in]
                      n1643 = call "mDrive Send Command.vi"("error in (no error)"=w3478, "Extra"=w3483, "Command"=T10."Move to Absolute Position", "VISA resource name"=w3479) -> ("error out"=w3480:errorcluster, "VISA resource name out"=w3481:refnum<visa-resource-name>)  [unwired: 3 in, 1 out]
                    }
                    frame #5 {
                      n1644 = Wait (ms)(milliseconds to wait=u32 50) -> ()  [unwired: 1 out]
                    }
                  }
                }
              }
              n1645 = case shown="True" w3271 {
                tunnel: w3259 -> [w3347 w3352]
                tunnel: w3260 -> [w3348 w3351]
                tunnel: [w3348 w3350] -> w3253
                tunnel: [w3347 w3349] -> w3254
                frame #0 {
                }
                frame #1 {
                  n1646 = flat-sequence {
                    tunnel: [w3380] -> w3366
                    tunnel: [w3379] -> w3365
                    tunnel: [w3367] -> w3364
                    tunnel: w3351 -> [w3379]
                    tunnel: w3352 -> [w3380]
                    tunnel: [w3383] -> w3363
                    tunnel: [w3382] -> w3362
                    tunnel: [w3381] -> w3361
                    tunnel: w3364 -> [w3381]
                    tunnel: w3365 -> [w3382]
                    tunnel: w3366 -> [w3383]
                    tunnel: [w3399] -> w3360
                    tunnel: [w3398] -> w3359
                    tunnel: w3363 -> [w3397]
                    tunnel: w3362 -> [w3396]
                    tunnel: [w3395] -> w3358
                    tunnel: w3361 -> [w3395]
                    tunnel: w3360 -> [w3406]
                    tunnel: [w3406] -> w3357
                    tunnel: w3359 -> [w3405]
                    tunnel: [w3405] -> w3356
                    tunnel: [w3403] -> w3355
                    tunnel: w3358 -> [w3403]
                    tunnel: [w3411] -> w3354
                    tunnel: [w3410] -> w3353
                    tunnel: w3357 -> [w3409]
                    tunnel: w3356 -> [w3408]
                    tunnel: w3355 -> [w3407]
                    tunnel: [w3414] -> w3349
                    tunnel: [w3416] -> w3350
                    tunnel: w3354 -> [w3416]
                    tunnel: w3353 -> [w3414]
                    frame #0 {
                      n1647 = property on="Y steps/rev" class="DigNum (strict)"() -> ("Value"=w3376:u32)  [unwired: 2 in, 2 out]
                      n1648 = To Double Precision Float(number=w3376) -> (double precision float=w3372:dbl)
                      n1649 = property on="Y offset mm" class="DigNum (strict)"() -> ("Value"=w3374:dbl)  [unwired: 2 in, 2 out]
                      n1650 = property on="Y Position SP mm" class="DigNum (strict)"() -> ("Value"=w3373:dbl)  [unwired: 2 in, 2 out]
                      n1651 = Subtract(x=w3373, y=w3374) -> (x-y=w3369:dbl)
                      n1652 = property on="Y mm/rev" class="DigNum (strict)"() -> ("Value"=w3375:dbl)  [unwired: 2 in, 2 out]
                      n1653 = Divide(x=w3369, y=w3375) -> (x/y=w3368:dbl)
                      n1654 = property on="Y Step SP" class="DigNum (strict)"() -> ("Maximum"=w3377:dbl)  [unwired: 2 in, 2 out]
                      n1655 = property on="Y Step SP" class="DigNum (strict)"() -> ("Minimum"=w3378:dbl)  [unwired: 2 in, 2 out]
                      n1656 = Multiply(x=w3368, y=w3372) -> (x*y=w3370:dbl)
                      n1657 = In Range and Coerce(upper limit=w3377, x=w3370, lower limit=w3378) -> (coerced(x)=w3371:dbl)  [unwired: 1 out]
                      n1658 = To Long Integer(number=w3371) -> (32bit integer=w3367:i32)
                      n1659 = property on="Y Step SP" class="DigNum (strict)"("Val(Sgnl)"=w3367) -> ()  [unwired: 2 in, 2 out]
                    }
                    frame #1 {
                      n1660 = property on="Y Step SP" class="DigNum (strict)"() -> ("Value"=w3392:i32)  [unwired: 2 in, 2 out]
                      n1661 = property on="Y Backlash" class="DigNum (strict)"() -> ("Value"=w3384:i32)  [unwired: 2 in, 2 out]
                      n1662 = property on="Y Step PV" class="DigNum (strict)"() -> ("Value"=w3391:i32)  [unwired: 2 in, 2 out]
                      n1663 = Subtract(x=w3392, y=w3391) -> (x-y=w3390:i32)
                      n1664 = Sign(1:w3384) -> (0:w3388:i32)
                      n1665 = Sign(1:w3390) -> (0:w3389:i32)
                      n1666 = Multiply(x=w3389, y=w3388) -> (x*y=w3387:i32)
                      n1667 = Equal?(x=w3387, y=1) -> (x = y?=w3385:bool)
                      n1668 = case shown="True" w3385 {
                        frame #0 {
                          n1669 = property on="Y Backlash corr" class="Bool (strict)"("Val(Sgnl)"=FALSE ("Value (Signaling)")) -> ()  [unwired: 2 in, 2 out]
                        }
                        frame #1 {
                          n1670 = property on="Y Backlash corr" class="Bool (strict)"("Val(Sgnl)"=TRUE ("Value (Signaling)")) -> ()  [unwired: 2 in, 2 out]
                        }
                      }
                    }
                    frame #2 {
                      # "Velocity Setting"
                      n1671 = property on="Y Velocity SP step/sec" class="DigNum (strict)"() -> ("Value"=w3400:i32)  [unwired: 2 in, 2 out]
                      n1672 = Number To Decimal String(number=w3400) -> (decimal integer string=w3401:string)  [unwired: 1 in]
                      n1673 = call "mDrive Send Command.vi"("error in (no error)"=w3397, "Extra"=w3401, "Command"=T10."Max Velocity", "VISA resource name"=w3396) -> ("error out"=w3398:errorcluster, "VISA resource name out"=w3399:refnum<visa-resource-name>)  [unwired: 3 in, 1 out]
                    }
                    frame #3 {
                      n1674 = Wait (ms)(milliseconds to wait=u32 50) -> ()  [unwired: 1 out]
                    }
                    frame #4 {
                      # "Move to Abs Position"
                      n1675 = Number To Decimal String(number=w3407) -> (decimal integer string=w3413:string)  [unwired: 1 in]
                      n1676 = call "mDrive Send Command.vi"("error in (no error)"=w3408, "Extra"=w3413, "Command"=T10."Move to Absolute Position", "VISA resource name"=w3409) -> ("error out"=w3410:errorcluster, "VISA resource name out"=w3411:refnum<visa-resource-name>)  [unwired: 3 in, 1 out]
                    }
                    frame #5 {
                      n1677 = Wait (ms)(milliseconds to wait=u32 25) -> ()  [unwired: 1 out]
                    }
                  }
                }
              }
              n1678 = case shown="True" w3268 {
                tunnel: w3257 -> [w3277 w3282]
                tunnel: w3258 -> [w3278 w3281]
                tunnel: [w3278 w3280] -> w3256
                tunnel: [w3277 w3279] -> w3255
                frame #0 {
                }
                frame #1 {
                  n1679 = flat-sequence {
                    tunnel: w3281 -> [w3309]
                    tunnel: w3282 -> [w3310]
                    tunnel: [w3310] -> w3296
                    tunnel: [w3309] -> w3295
                    tunnel: [w3297] -> w3294
                    tunnel: [w3313] -> w3293
                    tunnel: [w3312] -> w3292
                    tunnel: [w3311] -> w3291
                    tunnel: w3294 -> [w3311]
                    tunnel: w3295 -> [w3312]
                    tunnel: w3296 -> [w3313]
                    tunnel: [w3329] -> w3290
                    tunnel: [w3328] -> w3289
                    tunnel: w3293 -> [w3327]
                    tunnel: w3292 -> [w3326]
                    tunnel: [w3325] -> w3288
                    tunnel: w3291 -> [w3325]
                    tunnel: w3290 -> [w3336]
                    tunnel: [w3336] -> w3287
                    tunnel: w3289 -> [w3335]
                    tunnel: [w3335] -> w3286
                    tunnel: w3288 -> [w3334]
                    tunnel: [w3334] -> w3285
                    tunnel: [w3341] -> w3284
                    tunnel: [w3340] -> w3283
                    tunnel: w3287 -> [w3339]
                    tunnel: w3286 -> [w3338]
                    tunnel: w3285 -> [w3337]
                    tunnel: [w3346] -> w3280
                    tunnel: w3284 -> [w3346]
                    tunnel: w3283 -> [w3345]
                    tunnel: [w3345] -> w3279
                    frame #0 {
                      n1680 = property on="R steps/rev" class="DigNum (strict)"() -> ("Value"=w3305:u32)  [unwired: 2 in, 2 out]
                      n1681 = To Double Precision Float(number=w3305) -> (double precision float=w3302:dbl)
                      n1682 = property on="R offset deg" class="DigNum (strict)"() -> ("Value"=w3306:dbl)  [unwired: 2 in, 2 out]
                      n1683 = property on="R Position SP deg" class="DigNum (strict)"() -> ("Value"=w3307:dbl)  [unwired: 2 in, 2 out]
                      n1684 = Subtract(x=w3307, y=w3306) -> (x-y=w3299:dbl)
                      n1685 = property on="R deg/rev" class="DigNum (strict)"() -> ("Value"=w3308:dbl)  [unwired: 2 in, 2 out]
                      n1686 = Divide(x=w3299, y=w3308) -> (x/y=w3298:dbl)
                      n1687 = property on="R Step SP" class="DigNum (strict)"() -> ("Maximum"=w3303:dbl)  [unwired: 2 in, 2 out]
                      n1688 = Multiply(x=w3298, y=w3302) -> (x*y=w3300:dbl)
                      n1689 = property on="R Step SP" class="DigNum (strict)"() -> ("Minimum"=w3304:dbl)  [unwired: 2 in, 2 out]
                      n1690 = In Range and Coerce(upper limit=w3303, x=w3300, lower limit=w3304) -> (coerced(x)=w3301:dbl)  [unwired: 1 out]
                      n1691 = To Long Integer(number=w3301) -> (32bit integer=w3297:i32)
                      n1692 = property on="R Step SP" class="DigNum (strict)"("Val(Sgnl)"=w3297) -> ()  [unwired: 2 in, 2 out]
                    }
                    frame #1 {
                      n1693 = property on="R Step SP" class="DigNum (strict)"() -> ("Value"=w3322:i32)  [unwired: 2 in, 2 out]
                      n1694 = property on="R Step PV" class="DigNum (strict)"() -> ("Value"=w3321:i32)  [unwired: 2 in, 2 out]
                      n1695 = property on="R Backlash" class="DigNum (strict)"() -> ("Value"=w3314:i32)  [unwired: 2 in, 2 out]
                      n1696 = Subtract(x=w3322, y=w3321) -> (x-y=w3320:i32)
                      n1697 = Sign(1:w3314) -> (0:w3318:i32)
                      n1698 = Sign(1:w3320) -> (0:w3319:i32)
                      n1699 = Multiply(x=w3319, y=w3318) -> (x*y=w3317:i32)
                      n1700 = Equal?(x=w3317, y=1) -> (x = y?=w3315:bool)
                      n1701 = case shown="True" w3315 {
                        frame #0 {
                          n1702 = property on="R Backlash corr" class="Bool (strict)"("Val(Sgnl)"=FALSE ("Value (Signaling)")) -> ()  [unwired: 2 in, 2 out]
                        }
                        frame #1 {
                          n1703 = property on="R Backlash corr" class="Bool (strict)"("Val(Sgnl)"=TRUE ("Value (Signaling)")) -> ()  [unwired: 2 in, 2 out]
                        }
                      }
                    }
                    frame #2 {
                      # "Velocity Setting"
                      n1704 = property on="R Velocity SP step/sec" class="DigNum (strict)"() -> ("Value"=w3330:i32)  [unwired: 2 in, 2 out]
                      n1705 = Number To Decimal String(number=w3330) -> (decimal integer string=w3331:string)  [unwired: 1 in]
                      n1706 = call "mDrive Send Command.vi"("error in (no error)"=w3327, "Extra"=w3331, "Command"=T10."Max Velocity", "VISA resource name"=w3326) -> ("error out"=w3328:errorcluster, "VISA resource name out"=w3329:refnum<visa-resource-name>)  [unwired: 3 in, 1 out]
                    }
                    frame #3 {
                      n1707 = Wait (ms)(milliseconds to wait=u32 50) -> ()  [unwired: 1 out]
                    }
                    frame #4 {
                      # "Move to Abs Position"
                      n1708 = Number To Decimal String(number=w3337) -> (decimal integer string=w3343:string)  [unwired: 1 in]
                      n1709 = call "mDrive Send Command.vi"("error in (no error)"=w3338, "Extra"=w3343, "Command"=T10."Move to Absolute Position", "VISA resource name"=w3339) -> ("error out"=w3340:errorcluster, "VISA resource name out"=w3341:refnum<visa-resource-name>)  [unwired: 3 in, 1 out]
                    }
                    frame #5 {
                      n1710 = Wait (ms)(milliseconds to wait=u32 25) -> ()  [unwired: 1 out]
                    }
                  }
                }
              }
              n1711 = property on="Y in Motion" class="Bool (strict)"("Value"=w3247) -> ()  [unwired: 2 in, 2 out]
              n1712 = property on="R in Motion" class="Bool (strict)"("Value"=w3247) -> ()  [unwired: 2 in, 2 out]
              n1713 = property on="X  in Motion" class="Bool (strict)"("Value"=w3247) -> ()  [unwired: 2 in, 2 out]
              n1714 = property on="Z in Motion" class="Bool (strict)"("Value"=w3247) -> ()  [unwired: 2 in, 2 out]
            }
            frame #6 {
              n1715 = while {
                tunnel: [w3594] -> w3570
                tunnel: [w3593] -> w3569
                tunnel: [w3592] -> w3572
                tunnel: [w3591] -> w3571
                tunnel: [w3590] -> w3568
                tunnel: [w3589] -> w3567
                tunnel: [w3588] -> w3566
                tunnel: [w3587] -> w3565
                tunnel: w3564 -> [w3576]
                tunnel: w3563 -> [w3575]
                tunnel: w3562 -> [w3578]
                tunnel: w3561 -> [w3577]
                tunnel: w3560 -> [w3583]
                tunnel: w3559 -> [w3582]
                tunnel: w3558 -> [w3581]
                tunnel: w3557 -> [w3580]
                stop <- w3579 stop-if-true
                n1716 = flat-sequence {
                  tunnel: [w4040] -> w3650
                  tunnel: [w4039] -> w3649
                  tunnel: [w4038] -> w3648
                  tunnel: w3576 -> [w4036]
                  tunnel: w3575 -> [w4035]
                  tunnel: [w4062] -> w3647
                  tunnel: [w4061] -> w3646
                  tunnel: [w4059] -> w3645
                  tunnel: [w4060] -> w3644
                  tunnel: w3650 -> [w4059]
                  tunnel: w3649 -> [w4058]
                  tunnel: w3648 -> [w4057]
                  tunnel: w3647 -> [w4076]
                  tunnel: [w4076] -> w3640
                  tunnel: w3646 -> [w4075]
                  tunnel: [w4075] -> w3641
                  tunnel: w3645 -> [w4074]
                  tunnel: [w4074] -> w3642
                  tunnel: w3644 -> [w4073]
                  tunnel: [w4073] -> w3643
                  tunnel: [w4080] -> w3639
                  tunnel: [w4081] -> w3638
                  tunnel: [w4077] -> w3637
                  tunnel: w3643 -> [w4077]
                  tunnel: w3642 -> [w4078]
                  tunnel: w3641 -> [w4082]
                  tunnel: w3640 -> [w4079]
                  tunnel: w3639 -> [w4092]
                  tunnel: w3638 -> [w4093]
                  tunnel: w3637 -> [w4095]
                  tunnel: [w4091] -> w3593
                  tunnel: [w4090] -> w3594
                  frame #0 {
                    n1717 = property on="Z Step SP" class="DigNum (strict)"() -> ("Maximum"=w4052:dbl)  [unwired: 2 in, 2 out]
                    n1718 = property on="Z Step SP" class="DigNum (strict)"() -> ("Minimum"=w4054:dbl)  [unwired: 2 in, 2 out]
                    n1719 = property on="Z steps/rev" class="DigNum (strict)"() -> ("Value"=w4049:u32)  [unwired: 2 in, 2 out]
                    n1720 = property on="Z offset mm" class="DigNum (strict)"() -> ("Value"=w4045:dbl)  [unwired: 2 in, 2 out]
                    n1721 = To Long Integer(number=w4052) -> (32bit integer=w4051:i32)
                    n1722 = To Long Integer(number=w4054) -> (32bit integer=w4053:i32)
                    n1723 = To Double Precision Float(number=w4049) -> (double precision float=w4050:dbl)
                    n1724 = call "mDrive Send Command.vi"("error in (no error)"=w4035, "Extra"="P", "Command"=T10."Print Parameter", "VISA resource name"=w4036) -> ("error out"=w4038:errorcluster, "read buffer"=w4056:string, "VISA resource name out"=w4039:refnum<visa-resource-name>)  [unwired: 3 in]
                    n1725 = Decimal String To Number(string=w4056, offset=0) -> (number=w4037:i32)  [unwired: 1 in, 1 out]
                    n1726 = property on="Z Step PV" class="DigNum (strict)"("Val(Sgnl)"=w4037) -> ()  [unwired: 2 in, 2 out]
                    n1727 = In Range and Coerce(upper limit=w4051, x=w4037, lower limit=w4053) -> (In Range?=w4040:bool)  [unwired: 1 out]
                    n1728 = To Double Precision Float(number=w4037) -> (double precision float=w4044:dbl)
                    n1729 = property on="Z in Range" class="Bool (strict)"("Val(Sgnl)"=w4040) -> ()  [unwired: 2 in, 2 out]
                    n1730 = Divide(x=w4044, y=w4050) -> (x/y=w4048:dbl)
                    n1731 = property on="Z mm/rev" class="DigNum (strict)"() -> ("Value"=w4047:dbl)  [unwired: 2 in, 2 out]
                    n1732 = Multiply(x=w4048, y=w4047) -> (x*y=w4046:dbl)
                    n1733 = Add(x=w4046, y=w4045) -> (x+y=w4043:dbl)
                    n1734 = property on="Z Position mm PV" class="DigNum (strict)"("Val(Sgnl)"=w4043) -> ()  [unwired: 2 in, 2 out]
                  }
                  frame #1 {
                    n1735 = call "mDrive Send Command.vi"("error in (no error)"=w4057, "Extra"="MV", "Command"=T10."Print Parameter", "VISA resource name"=w4058) -> ("error out"=w4061:errorcluster, "read buffer"=w4065:string, "VISA resource name out"=w4062:refnum<visa-resource-name>)  [unwired: 3 in]
                    n1736 = Decimal String To Number(string=w4065, offset=0 ("offset (0)")) -> (number=w4068:i32)  [unwired: 1 in, 1 out]
                    n1737 = Not Equal?(x=w4065, y="") -> (x != y?=w4063:bool)
                    n1738 = property on="Z Ready" class="Bool (strict)"("Val(Sgnl)"=w4063) -> ()  [unwired: 2 in, 2 out]
                    n1739 = Number To Boolean Array(number=w4068) -> (Boolean array=w4067:bool[])
                    n1740 = Index Array(array=w4067, index=0) -> (element=w4060:bool)
                    n1741 = property on="Z in Motion" class="Bool (strict)"("Val(Sgnl)"=w4060) -> ()  [unwired: 2 in, 2 out]
                  }
                  frame #2 {
                    n1742 = Wait (ms)(milliseconds to wait=u32 50) -> ()  [unwired: 1 out]
                  }
                  frame #3 {
                    n1743 = case shown="True" w4078 {
                      tunnel: w4079 -> [w4085 w4089]
                      tunnel: [w4086 w4089] -> w4080
                      tunnel: [w4087 w4088] -> w4081
                      tunnel: w4082 -> [w4084 w4088]
                      frame #0 {
                        n1744 = call "mDrive Send Command.vi"("error in (no error)"=w4084, "Command"=T10."Stop", "VISA resource name"=w4085) -> ("error out"=w4087:errorcluster, "VISA resource name out"=w4086:refnum<visa-resource-name>)  [unwired: 4 in, 1 out]
                      }
                      frame #1 {
                      }
                    }
                  }
                  frame #4 {
                    n1745 = property on="Z Backlash corr" class="Bool (strict)"() -> ("Value"=w4096:bool)  [unwired: 2 in, 2 out]
                    n1746 = Implies(1:w4095, 2:w4096) -> (0:w4094:bool)
                    n1747 = case shown="False" w4094 {
                      tunnel: w4093 -> [w4104 w4161]
                      tunnel: w4092 -> [w4103 w4162]
                      tunnel: [w4098 w4161] -> w4091
                      tunnel: [w4102 w4162] -> w4090
                      frame #0 {
                        # "Backlash"
                        n1748 = flat-sequence {
                          tunnel: [w4119] -> w4116
                          tunnel: [w4121] -> w4115
                          tunnel: [w4120] -> w4114
                          tunnel: w4104 -> [w4118]
                          tunnel: w4103 -> [w4117]
                          tunnel: w4116 -> [w4129]
                          tunnel: [w4129] -> w4113
                          tunnel: w4115 -> [w4128]
                          tunnel: w4114 -> [w4127]
                          tunnel: [w4126] -> w4112
                          tunnel: [w4125] -> w4111
                          tunnel: [w4124] -> w4101
                          tunnel: w4113 -> [w4143]
                          tunnel: w4112 -> [w4134]
                          tunnel: w4111 -> [w4142]
                          tunnel: [w4134] -> w4110
                          tunnel: [w4142] -> w4109
                          tunnel: [w4133] -> w4106
                          tunnel: [w4141] -> w4105
                          tunnel: w4101 -> [w4141]
                          tunnel: w4110 -> [w4146]
                          tunnel: w4109 -> [w4147]
                          tunnel: [w4145] -> w4108
                          tunnel: [w4153] -> w4107
                          tunnel: w4106 -> [w4153]
                          tunnel: w4105 -> [w4149]
                          tunnel: [w4148] -> w4099
                          tunnel: w4108 -> [w4156]
                          tunnel: w4107 -> [w4155]
                          tunnel: [w4157] -> w4100
                          tunnel: w4099 -> [w4157]
                          tunnel: [w4156] -> w4097
                          tunnel: [w4160] -> w4102
                          tunnel: w4100 -> [w4160]
                          tunnel: [w4158] -> w4098
                          tunnel: w4097 -> [w4158]
                          frame #0 {
                            n1749 = property on="Z Backlash steps/sec" class="DigNum (strict)"() -> ("Value"=w4119:i32)  [unwired: 2 in, 2 out]
                            n1750 = Number To Decimal String(number=w4119) -> (decimal integer string=w4122:string)  [unwired: 1 in]
                            n1751 = call "mDrive Send Command.vi"("error in (no error)"=w4118, "Extra"=w4122, "Command"=T10."Max Velocity", "VISA resource name"=w4117) -> ("error out"=w4120:errorcluster, "VISA resource name out"=w4121:refnum<visa-resource-name>)  [unwired: 3 in, 1 out]
                          }
                          frame #1 {
                            n1752 = property on="Z Backlash" class="DigNum (strict)"() -> ("Value"=w4124:i32)  [unwired: 2 in, 2 out]
                            n1753 = Number To Decimal String(number=w4124) -> (decimal integer string=w4130:string)  [unwired: 1 in]
                            n1754 = call "mDrive Send Command.vi"("error in (no error)"=w4127, "Extra"=w4130, "Command"=T10."Move to Relative Position", "VISA resource name"=w4128) -> ("error out"=w4126:errorcluster, "VISA resource name out"=w4125:refnum<visa-resource-name>)  [unwired: 3 in, 1 out]
                          }
                          frame #2 {
                            n1755 = To Double Precision Float(number=w4141) -> (double precision float=w4139:dbl)
                            n1756 = To Double Precision Float(number=w4143) -> (double precision float=w4144:dbl)
                            n1757 = Absolute Value(x=w4139) -> (abs(x)=w4140:dbl)
                            n1758 = Divide(x=w4140, y=w4144) -> (x/y=w4137:dbl)
                            n1759 = Multiply(x=1000.0, y=w4137) -> (x*y=w4135:dbl)
                            n1760 = Add(x=w4135, y=300.0) -> (x+y=w4133:dbl)
                            n1761 = To Unsigned Long Integer(number=w4133) -> (unsigned 32bit integer=w4132:u32)
                            n1762 = Wait (ms)(milliseconds to wait=w4132) -> ()  [unwired: 1 out]
                          }
                          frame #3 {
                            n1763 = Negate(x=w4149) -> (-x=w4150:i32)
                            n1764 = Number To Decimal String(number=w4150) -> (decimal integer string=w4151:string)  [unwired: 1 in]
                            n1765 = call "mDrive Send Command.vi"("error in (no error)"=w4146, "Extra"=w4151, "Command"=T10."Move to Relative Position", "VISA resource name"=w4147) -> ("error out"=w4145:errorcluster, "VISA resource name out"=w4148:refnum<visa-resource-name>)  [unwired: 3 in, 1 out]
                          }
                          frame #4 {
                            n1766 = To Unsigned Long Integer(number=w4155) -> (unsigned 32bit integer=w4154:u32)
                            n1767 = Wait (ms)(milliseconds to wait=w4154) -> ()  [unwired: 1 out]
                          }
                          frame #5 {
                            n1768 = property on="Z Backlash corr" class="Bool (strict)"("Val(Sgnl)"=FALSE ("Value (Signaling)")) -> ()  [unwired: 2 in, 2 out]
                          }
                        }
                      }
                      frame #1 {
                      }
                    }
                  }
                }
                n1769 = flat-sequence {
                  tunnel: [w3918] -> w3636
                  tunnel: [w3911] -> w3635
                  tunnel: [w3910] -> w3634
                  tunnel: w3578 -> [w3908]
                  tunnel: w3577 -> [w3907]
                  tunnel: [w3938] -> w3633
                  tunnel: [w3937] -> w3632
                  tunnel: [w3936] -> w3631
                  tunnel: [w3929] -> w3630
                  tunnel: w3636 -> [w3936]
                  tunnel: w3635 -> [w3935]
                  tunnel: w3634 -> [w3934]
                  tunnel: w3633 -> [w3948]
                  tunnel: [w3948] -> w3626
                  tunnel: w3632 -> [w3947]
                  tunnel: [w3947] -> w3627
                  tunnel: w3631 -> [w3946]
                  tunnel: [w3946] -> w3628
                  tunnel: w3630 -> [w3945]
                  tunnel: [w3945] -> w3629
                  tunnel: [w3952] -> w3625
                  tunnel: [w3953] -> w3624
                  tunnel: [w3949] -> w3623
                  tunnel: w3629 -> [w3949]
                  tunnel: w3628 -> [w3950]
                  tunnel: w3627 -> [w3954]
                  tunnel: w3626 -> [w3951]
                  tunnel: w3625 -> [w3965]
                  tunnel: w3624 -> [w3966]
                  tunnel: w3623 -> [w3968]
                  tunnel: [w3964] -> w3591
                  tunnel: [w3963] -> w3592
                  frame #0 {
                    n1770 = property on="X Step SP" class="DigNum (strict)"() -> ("Maximum"=w3919:dbl)  [unwired: 2 in, 2 out]
                    n1771 = property on="X Step SP" class="DigNum (strict)"() -> ("Minimum"=w3913:dbl)  [unwired: 2 in, 2 out]
                    n1772 = property on="X steps/rev" class="DigNum (strict)"() -> ("Value"=w3917:u32)  [unwired: 2 in, 2 out]
                    n1773 = property on="X offset mm" class="DigNum (strict)"() -> ("Value"=w3915:dbl)  [unwired: 2 in, 2 out]
                    n1774 = To Long Integer(number=w3919) -> (32bit integer=w3925:i32)
                    n1775 = To Long Integer(number=w3913) -> (32bit integer=w3926:i32)
                    n1776 = To Double Precision Float(number=w3917) -> (double precision float=w3924:dbl)
                    n1777 = call "mDrive Send Command.vi"("error in (no error)"=w3907, "Extra"="P", "Command"=T10."Print Parameter", "VISA resource name"=w3908) -> ("error out"=w3910:errorcluster, "read buffer"=w3928:string, "VISA resource name out"=w3911:refnum<visa-resource-name>)  [unwired: 3 in]
                    n1778 = Decimal String To Number(string=w3928, offset=0) -> (number=w3909:i32)  [unwired: 1 in, 1 out]
                    n1779 = property on="X Step PV" class="DigNum (strict)"("Val(Sgnl)"=w3909) -> ()  [unwired: 2 in, 2 out]
                    n1780 = In Range and Coerce(upper limit=w3925, x=w3909, lower limit=w3926) -> (In Range?=w3918:bool)  [unwired: 1 out]
                    n1781 = To Double Precision Float(number=w3909) -> (double precision float=w3922:dbl)
                    n1782 = property on="X  in Range" class="Bool (strict)"("Val(Sgnl)"=w3918) -> ()  [unwired: 2 in, 2 out]
                    n1783 = Divide(x=w3922, y=w3924) -> (x/y=w3923:dbl)
                    n1784 = property on="X mm/rev" class="DigNum (strict)"() -> ("Value"=w3916:dbl)  [unwired: 2 in, 2 out]
                    n1785 = Multiply(x=w3923, y=w3916) -> (x*y=w3912:dbl)
                    n1786 = Add(x=w3912, y=w3915) -> (x+y=w3914:dbl)
                    n1787 = property on="X Position mm PV" class="DigNum (strict)"("Val(Sgnl)"=w3914) -> ()  [unwired: 2 in, 2 out]
                  }
                  frame #1 {
                    n1788 = call "mDrive Send Command.vi"("error in (no error)"=w3934, "Extra"="MV", "Command"=T10."Print Parameter", "VISA resource name"=w3935) -> ("error out"=w3937:errorcluster, "read buffer"=w3940:string, "VISA resource name out"=w3938:refnum<visa-resource-name>)  [unwired: 3 in]
                    n1789 = Decimal String To Number(string=w3940, offset=0 ("offset (0)")) -> (number=w3930:i32)  [unwired: 1 in, 1 out]
                    n1790 = Not Equal?(x=w3940, y="") -> (x != y?=w3933:bool)
                    n1791 = property on="X Ready" class="Bool (strict)"("Val(Sgnl)"=w3933) -> ()  [unwired: 2 in, 2 out]
                    n1792 = Number To Boolean Array(number=w3930) -> (Boolean array=w3932:bool[])
                    n1793 = Index Array(array=w3932, index=0) -> (element=w3929:bool)
                    n1794 = property on="X  in Motion" class="Bool (strict)"("Val(Sgnl)"=w3929) -> ()  [unwired: 2 in, 2 out]
                  }
                  frame #2 {
                    n1795 = Wait (ms)(milliseconds to wait=u32 50) -> ()  [unwired: 1 out]
                  }
                  frame #3 {
                    n1796 = case shown="False" w3950 {
                      tunnel: w3951 -> [w3957 w3961]
                      tunnel: [w3958 w3961] -> w3952
                      tunnel: [w3959 w3960] -> w3953
                      tunnel: w3954 -> [w3956 w3960]
                      frame #0 {
                        n1797 = call "mDrive Send Command.vi"("error in (no error)"=w3956, "Command"=T10."Stop", "VISA resource name"=w3957) -> ("error out"=w3959:errorcluster, "VISA resource name out"=w3958:refnum<visa-resource-name>)  [unwired: 4 in, 1 out]
                      }
                      frame #1 {
                      }
                    }
                  }
                  frame #4 {
                    n1798 = property on="X Backlash corr" class="Bool (strict)"() -> ("Value"=w3962:bool)  [unwired: 2 in, 2 out]
                    n1799 = Implies(1:w3968, 2:w3962) -> (0:w3967:bool)
                    n1800 = case shown="False" w3967 {
                      tunnel: w3966 -> [w3976 w4033]
                      tunnel: w3965 -> [w3975 w4034]
                      tunnel: [w3970 w4033] -> w3964
                      tunnel: [w3974 w4034] -> w3963
                      frame #0 {
                        # "Backlash"
                        n1801 = flat-sequence {
                          tunnel: [w3989] -> w3988
                          tunnel: [w3993] -> w3987
                          tunnel: [w3992] -> w3986
                          tunnel: w3976 -> [w3991]
                          tunnel: w3975 -> [w3990]
                          tunnel: w3988 -> [w4001]
                          tunnel: [w4001] -> w3985
                          tunnel: w3987 -> [w4000]
                          tunnel: w3986 -> [w3999]
                          tunnel: [w3998] -> w3984
                          tunnel: [w3997] -> w3983
                          tunnel: [w3996] -> w3973
                          tunnel: w3985 -> [w4015]
                          tunnel: w3984 -> [w4006]
                          tunnel: w3983 -> [w4014]
                          tunnel: [w4006] -> w3982
                          tunnel: [w4014] -> w3981
                          tunnel: [w4005] -> w3978
                          tunnel: [w4013] -> w3977
                          tunnel: w3973 -> [w4013]
                          tunnel: w3982 -> [w4018]
                          tunnel: w3981 -> [w4019]
                          tunnel: [w4017] -> w3980
                          tunnel: [w4025] -> w3979
                          tunnel: w3978 -> [w4025]
                          tunnel: w3977 -> [w4021]
                          tunnel: [w4020] -> w3971
                          tunnel: w3980 -> [w4028]
                          tunnel: w3979 -> [w4027]
                          tunnel: [w4029] -> w3972
                          tunnel: w3971 -> [w4029]
                          tunnel: [w4028] -> w3969
                          tunnel: [w4032] -> w3974
                          tunnel: w3972 -> [w4032]
                          tunnel: [w4031] -> w3970
                          tunnel: w3969 -> [w4031]
                          frame #0 {
                            n1802 = property on="X Backlash steps/sec" class="DigNum (strict)"() -> ("Value"=w3989:i32)  [unwired: 2 in, 2 out]
                            n1803 = Number To Decimal String(number=w3989) -> (decimal integer string=w3994:string)  [unwired: 1 in]
                            n1804 = call "mDrive Send Command.vi"("error in (no error)"=w3991, "Extra"=w3994, "Command"=T10."Max Velocity", "VISA resource name"=w3990) -> ("error out"=w3992:errorcluster, "VISA resource name out"=w3993:refnum<visa-resource-name>)  [unwired: 3 in, 1 out]
                          }
                          frame #1 {
                            n1805 = property on="X Backlash" class="DigNum (strict)"() -> ("Value"=w3996:i32)  [unwired: 2 in, 2 out]
                            n1806 = Number To Decimal String(number=w3996) -> (decimal integer string=w4002:string)  [unwired: 1 in]
                            n1807 = call "mDrive Send Command.vi"("error in (no error)"=w3999, "Extra"=w4002, "Command"=T10."Move to Relative Position", "VISA resource name"=w4000) -> ("error out"=w3998:errorcluster, "VISA resource name out"=w3997:refnum<visa-resource-name>)  [unwired: 3 in, 1 out]
                          }
                          frame #2 {
                            n1808 = To Double Precision Float(number=w4013) -> (double precision float=w4011:dbl)
                            n1809 = To Double Precision Float(number=w4015) -> (double precision float=w4016:dbl)
                            n1810 = Absolute Value(x=w4011) -> (abs(x)=w4012:dbl)
                            n1811 = Divide(x=w4012, y=w4016) -> (x/y=w4009:dbl)
                            n1812 = Multiply(x=1000.0, y=w4009) -> (x*y=w4007:dbl)
                            n1813 = Add(x=w4007, y=300.0) -> (x+y=w4005:dbl)
                            n1814 = To Unsigned Long Integer(number=w4005) -> (unsigned 32bit integer=w4004:u32)
                            n1815 = Wait (ms)(milliseconds to wait=w4004) -> ()  [unwired: 1 out]
                          }
                          frame #3 {
                            n1816 = Negate(x=w4021) -> (-x=w4022:i32)
                            n1817 = Number To Decimal String(number=w4022) -> (decimal integer string=w4023:string)  [unwired: 1 in]
                            n1818 = call "mDrive Send Command.vi"("error in (no error)"=w4018, "Extra"=w4023, "Command"=T10."Move to Relative Position", "VISA resource name"=w4019) -> ("error out"=w4017:errorcluster, "VISA resource name out"=w4020:refnum<visa-resource-name>)  [unwired: 3 in, 1 out]
                          }
                          frame #4 {
                            n1819 = To Unsigned Long Integer(number=w4027) -> (unsigned 32bit integer=w4026:u32)
                            n1820 = Wait (ms)(milliseconds to wait=w4026) -> ()  [unwired: 1 out]
                          }
                          frame #5 {
                            n1821 = property on="X Backlash corr" class="Bool (strict)"("Val(Sgnl)"=FALSE ("Value (Signaling)")) -> ()  [unwired: 2 in, 2 out]
                          }
                        }
                      }
                      frame #1 {
                      }
                    }
                  }
                }
                n1822 = flat-sequence {
                  tunnel: [w3788] -> w3622
                  tunnel: [w3790] -> w3621
                  tunnel: [w3789] -> w3620
                  tunnel: w3583 -> [w3780]
                  tunnel: w3582 -> [w3779]
                  tunnel: [w3810] -> w3619
                  tunnel: [w3809] -> w3618
                  tunnel: [w3808] -> w3617
                  tunnel: [w3801] -> w3616
                  tunnel: w3622 -> [w3808]
                  tunnel: w3621 -> [w3807]
                  tunnel: w3620 -> [w3806]
                  tunnel: w3619 -> [w3820]
                  tunnel: [w3820] -> w3612
                  tunnel: w3618 -> [w3819]
                  tunnel: [w3819] -> w3613
                  tunnel: w3617 -> [w3818]
                  tunnel: [w3818] -> w3614
                  tunnel: w3616 -> [w3817]
                  tunnel: [w3817] -> w3615
                  tunnel: [w3824] -> w3611
                  tunnel: [w3825] -> w3610
                  tunnel: [w3821] -> w3609
                  tunnel: w3615 -> [w3821]
                  tunnel: w3614 -> [w3822]
                  tunnel: w3613 -> [w3826]
                  tunnel: w3612 -> [w3823]
                  tunnel: w3611 -> [w3837]
                  tunnel: w3610 -> [w3838]
                  tunnel: w3609 -> [w3840]
                  tunnel: [w3836] -> w3589
                  tunnel: [w3835] -> w3590
                  frame #0 {
                    n1823 = property on="Y Step SP" class="DigNum (strict)"() -> ("Maximum"=w3783:dbl)  [unwired: 2 in, 2 out]
                    n1824 = property on="Y Step SP" class="DigNum (strict)"() -> ("Minimum"=w3782:dbl)  [unwired: 2 in, 2 out]
                    n1825 = property on="Y steps/rev" class="DigNum (strict)"() -> ("Value"=w3784:u32)  [unwired: 2 in, 2 out]
                    n1826 = property on="Y offset mm" class="DigNum (strict)"() -> ("Value"=w3786:dbl)  [unwired: 2 in, 2 out]
                    n1827 = To Long Integer(number=w3783) -> (32bit integer=w3797:i32)
                    n1828 = To Long Integer(number=w3782) -> (32bit integer=w3798:i32)
                    n1829 = To Double Precision Float(number=w3784) -> (double precision float=w3796:dbl)
                    n1830 = call "mDrive Send Command.vi"("error in (no error)"=w3780, "Extra"="P", "Command"=T10."Print Parameter", "VISA resource name"=w3779) -> ("error out"=w3789:errorcluster, "read buffer"=w3800:string, "VISA resource name out"=w3790:refnum<visa-resource-name>)  [unwired: 3 in]
                    n1831 = Decimal String To Number(string=w3800, offset=0) -> (number=w3781:i32)  [unwired: 1 in, 1 out]
                    n1832 = property on="Y Step PV" class="DigNum (strict)"("Val(Sgnl)"=w3781) -> ()  [unwired: 2 in, 2 out]
                    n1833 = In Range and Coerce(upper limit=w3797, x=w3781, lower limit=w3798) -> (In Range?=w3788:bool)  [unwired: 1 out]
                    n1834 = To Double Precision Float(number=w3781) -> (double precision float=w3793:dbl)
                    n1835 = property on="Y in Range" class="Bool (strict)"("Val(Sgnl)"=w3788) -> ()  [unwired: 2 in, 2 out]
                    n1836 = Divide(x=w3793, y=w3796) -> (x/y=w3795:dbl)
                    n1837 = property on="Y mm/rev" class="DigNum (strict)"() -> ("Value"=w3785:dbl)  [unwired: 2 in, 2 out]
                    n1838 = Multiply(x=w3795, y=w3785) -> (x*y=w3794:dbl)
                    n1839 = Add(x=w3794, y=w3786) -> (x+y=w3787:dbl)
                    n1840 = property on="Y Position mm PV" class="DigNum (strict)"("Val(Sgnl)"=w3787) -> ()  [unwired: 2 in, 2 out]
                  }
                  frame #1 {
                    n1841 = call "mDrive Send Command.vi"("error in (no error)"=w3806, "Extra"="MV", "Command"=T10."Print Parameter", "VISA resource name"=w3807) -> ("error out"=w3809:errorcluster, "read buffer"=w3812:string, "VISA resource name out"=w3810:refnum<visa-resource-name>)  [unwired: 3 in]
                    n1842 = Decimal String To Number(string=w3812, offset=0 ("offset (0)")) -> (number=w3802:i32)  [unwired: 1 in, 1 out]
                    n1843 = Not Equal?(x=w3812, y="") -> (x != y?=w3805:bool)
                    n1844 = property on="Y Ready" class="Bool (strict)"("Val(Sgnl)"=w3805) -> ()  [unwired: 2 in, 2 out]
                    n1845 = Number To Boolean Array(number=w3802) -> (Boolean array=w3804:bool[])
                    n1846 = Index Array(array=w3804, index=0) -> (element=w3801:bool)
                    n1847 = property on="Y in Motion" class="Bool (strict)"("Val(Sgnl)"=w3801) -> ()  [unwired: 2 in, 2 out]
                  }
                  frame #2 {
                    n1848 = Wait (ms)(milliseconds to wait=u32 50) -> ()  [unwired: 1 out]
                  }
                  frame #3 {
                    n1849 = case shown="False" w3822 {
                      tunnel: w3823 -> [w3829 w3832]
                      tunnel: [w3830 w3832] -> w3824
                      tunnel: [w3831 w3833] -> w3825
                      tunnel: w3826 -> [w3828 w3833]
                      frame #0 {
                        n1850 = call "mDrive Send Command.vi"("error in (no error)"=w3828, "Command"=T10."Stop", "VISA resource name"=w3829) -> ("error out"=w3831:errorcluster, "VISA resource name out"=w3830:refnum<visa-resource-name>)  [unwired: 4 in, 1 out]
                      }
                      frame #1 {
                      }
                    }
                  }
                  frame #4 {
                    n1851 = property on="Y Backlash corr" class="Bool (strict)"() -> ("Value"=w3834:bool)  [unwired: 2 in, 2 out]
                    n1852 = Implies(1:w3840, 2:w3834) -> (0:w3839:bool)
                    n1853 = case shown="False" w3839 {
                      tunnel: w3838 -> [w3848 w3905]
                      tunnel: w3837 -> [w3847 w3906]
                      tunnel: [w3842 w3905] -> w3836
                      tunnel: [w3846 w3906] -> w3835
                      frame #0 {
                        # "Backlash"
                        n1854 = flat-sequence {
                          tunnel: [w3861] -> w3860
                          tunnel: [w3865] -> w3859
                          tunnel: [w3864] -> w3858
                          tunnel: w3848 -> [w3863]
                          tunnel: w3847 -> [w3862]
                          tunnel: w3860 -> [w3873]
                          tunnel: [w3873] -> w3857
                          tunnel: w3859 -> [w3872]
                          tunnel: w3858 -> [w3871]
                          tunnel: [w3870] -> w3856
                          tunnel: [w3869] -> w3855
                          tunnel: [w3868] -> w3845
                          tunnel: w3857 -> [w3887]
                          tunnel: w3856 -> [w3878]
                          tunnel: w3855 -> [w3886]
                          tunnel: [w3878] -> w3854
                          tunnel: [w3886] -> w3853
                          tunnel: [w3877] -> w3850
                          tunnel: [w3885] -> w3849
                          tunnel: w3845 -> [w3885]
                          tunnel: w3854 -> [w3890]
                          tunnel: w3853 -> [w3891]
                          tunnel: [w3889] -> w3852
                          tunnel: [w3897] -> w3851
                          tunnel: w3850 -> [w3897]
                          tunnel: w3849 -> [w3893]
                          tunnel: [w3892] -> w3843
                          tunnel: w3852 -> [w3900]
                          tunnel: w3851 -> [w3899]
                          tunnel: [w3901] -> w3844
                          tunnel: w3843 -> [w3901]
                          tunnel: [w3900] -> w3841
                          tunnel: [w3904] -> w3846
                          tunnel: w3844 -> [w3904]
                          tunnel: [w3903] -> w3842
                          tunnel: w3841 -> [w3903]
                          frame #0 {
                            n1855 = property on="Y Backlash steps/sec" class="DigNum (strict)"() -> ("Value"=w3861:i32)  [unwired: 2 in, 2 out]
                            n1856 = Number To Decimal String(number=w3861) -> (decimal integer string=w3866:string)  [unwired: 1 in]
                            n1857 = call "mDrive Send Command.vi"("error in (no error)"=w3863, "Extra"=w3866, "Command"=T10."Max Velocity", "VISA resource name"=w3862) -> ("error out"=w3864:errorcluster, "VISA resource name out"=w3865:refnum<visa-resource-name>)  [unwired: 3 in, 1 out]
                          }
                          frame #1 {
                            n1858 = property on="Y Backlash" class="DigNum (strict)"() -> ("Value"=w3868:i32)  [unwired: 2 in, 2 out]
                            n1859 = Number To Decimal String(number=w3868) -> (decimal integer string=w3874:string)  [unwired: 1 in]
                            n1860 = call "mDrive Send Command.vi"("error in (no error)"=w3871, "Extra"=w3874, "Command"=T10."Move to Relative Position", "VISA resource name"=w3872) -> ("error out"=w3870:errorcluster, "VISA resource name out"=w3869:refnum<visa-resource-name>)  [unwired: 3 in, 1 out]
                          }
                          frame #2 {
                            n1861 = To Double Precision Float(number=w3885) -> (double precision float=w3883:dbl)
                            n1862 = To Double Precision Float(number=w3887) -> (double precision float=w3888:dbl)
                            n1863 = Absolute Value(x=w3883) -> (abs(x)=w3884:dbl)
                            n1864 = Divide(x=w3884, y=w3888) -> (x/y=w3881:dbl)
                            n1865 = Multiply(x=1000.0, y=w3881) -> (x*y=w3879:dbl)
                            n1866 = Add(x=w3879, y=300.0) -> (x+y=w3877:dbl)
                            n1867 = To Unsigned Long Integer(number=w3877) -> (unsigned 32bit integer=w3876:u32)
                            n1868 = Wait (ms)(milliseconds to wait=w3876) -> ()  [unwired: 1 out]
                          }
                          frame #3 {
                            n1869 = Negate(x=w3893) -> (-x=w3894:i32)
                            n1870 = Number To Decimal String(number=w3894) -> (decimal integer string=w3895:string)  [unwired: 1 in]
                            n1871 = call "mDrive Send Command.vi"("error in (no error)"=w3890, "Extra"=w3895, "Command"=T10."Move to Relative Position", "VISA resource name"=w3891) -> ("error out"=w3889:errorcluster, "VISA resource name out"=w3892:refnum<visa-resource-name>)  [unwired: 3 in, 1 out]
                          }
                          frame #4 {
                            n1872 = To Unsigned Long Integer(number=w3899) -> (unsigned 32bit integer=w3898:u32)
                            n1873 = Wait (ms)(milliseconds to wait=w3898) -> ()  [unwired: 1 out]
                          }
                          frame #5 {
                            n1874 = property on="Y Backlash corr" class="Bool (strict)"("Val(Sgnl)"=FALSE ("Value (Signaling)")) -> ()  [unwired: 2 in, 2 out]
                          }
                        }
                      }
                      frame #1 {
                      }
                    }
                  }
                }
                n1875 = flat-sequence {
                  tunnel: [w3660] -> w3608
                  tunnel: [w3662] -> w3607
                  tunnel: [w3661] -> w3606
                  tunnel: w3581 -> [w3652]
                  tunnel: w3580 -> [w3651]
                  tunnel: [w3682] -> w3605
                  tunnel: [w3681] -> w3604
                  tunnel: [w3680] -> w3603
                  tunnel: [w3673] -> w3602
                  tunnel: w3608 -> [w3680]
                  tunnel: w3607 -> [w3679]
                  tunnel: w3606 -> [w3678]
                  tunnel: w3605 -> [w3692]
                  tunnel: [w3692] -> w3598
                  tunnel: w3604 -> [w3691]
                  tunnel: [w3691] -> w3599
                  tunnel: w3603 -> [w3690]
                  tunnel: [w3690] -> w3600
                  tunnel: w3602 -> [w3689]
                  tunnel: [w3689] -> w3601
                  tunnel: [w3696] -> w3597
                  tunnel: [w3697] -> w3596
                  tunnel: [w3693] -> w3595
                  tunnel: w3601 -> [w3693]
                  tunnel: w3600 -> [w3694]
                  tunnel: w3599 -> [w3698]
                  tunnel: w3598 -> [w3695]
                  tunnel: w3597 -> [w3709]
                  tunnel: w3596 -> [w3710]
                  tunnel: w3595 -> [w3712]
                  tunnel: [w3708] -> w3587
                  tunnel: [w3707] -> w3588
                  frame #0 {
                    n1876 = property on="R Step SP" class="DigNum (strict)"() -> ("Maximum"=w3655:dbl)  [unwired: 2 in, 2 out]
                    n1877 = property on="R Step SP" class="DigNum (strict)"() -> ("Minimum"=w3656:dbl)  [unwired: 2 in, 2 out]
                    n1878 = property on="R steps/rev" class="DigNum (strict)"() -> ("Value"=w3654:u32)  [unwired: 2 in, 2 out]
                    n1879 = property on="R offset deg" class="DigNum (strict)"() -> ("Value"=w3658:dbl)  [unwired: 2 in, 2 out]
                    n1880 = To Long Integer(number=w3655) -> (32bit integer=w3669:i32)
                    n1881 = To Long Integer(number=w3656) -> (32bit integer=w3670:i32)
                    n1882 = To Double Precision Float(number=w3654) -> (double precision float=w3668:dbl)
                    n1883 = call "mDrive Send Command.vi"("error in (no error)"=w3652, "Extra"="P", "Command"=T10."Print Parameter", "VISA resource name"=w3651) -> ("error out"=w3661:errorcluster, "read buffer"=w3672:string, "VISA resource name out"=w3662:refnum<visa-resource-name>)  [unwired: 3 in]
                    n1884 = Decimal String To Number(string=w3672, offset=0) -> (number=w3653:i32)  [unwired: 1 in, 1 out]
                    n1885 = property on="R Step PV" class="DigNum (strict)"("Val(Sgnl)"=w3653) -> ()  [unwired: 2 in, 2 out]
                    n1886 = In Range and Coerce(upper limit=w3669, x=w3653, lower limit=w3670) -> (In Range?=w3660:bool)  [unwired: 1 out]
                    n1887 = To Double Precision Float(number=w3653) -> (double precision float=w3665:dbl)
                    n1888 = property on="R in Range" class="Bool (strict)"("Val(Sgnl)"=w3660) -> ()  [unwired: 2 in, 2 out]
                    n1889 = Divide(x=w3665, y=w3668) -> (x/y=w3667:dbl)
                    n1890 = property on="R deg/rev" class="DigNum (strict)"() -> ("Value"=w3657:dbl)  [unwired: 2 in, 2 out]
                    n1891 = Multiply(x=w3667, y=w3657) -> (x*y=w3666:dbl)
                    n1892 = Add(x=w3666, y=w3658) -> (x+y=w3659:dbl)
                    n1893 = property on="R Position deg PV" class="DigNum (strict)"("Val(Sgnl)"=w3659) -> ()  [unwired: 2 in, 2 out]
                  }
                  frame #1 {
                    n1894 = call "mDrive Send Command.vi"("error in (no error)"=w3678, "Extra"="MV", "Command"=T10."Print Parameter", "VISA resource name"=w3679) -> ("error out"=w3681:errorcluster, "read buffer"=w3684:string, "VISA resource name out"=w3682:refnum<visa-resource-name>)  [unwired: 3 in]
                    n1895 = Decimal String To Number(string=w3684, offset=0 ("offset (0)")) -> (number=w3674:i32)  [unwired: 1 in, 1 out]
                    n1896 = Not Equal?(x=w3684, y="") -> (x != y?=w3677:bool)
                    n1897 = property on="R Ready" class="Bool (strict)"("Val(Sgnl)"=w3677) -> ()  [unwired: 2 in, 2 out]
                    n1898 = Number To Boolean Array(number=w3674) -> (Boolean array=w3676:bool[])
                    n1899 = Index Array(array=w3676, index=0) -> (element=w3673:bool)
                    n1900 = property on="R in Motion" class="Bool (strict)"("Val(Sgnl)"=w3673) -> ()  [unwired: 2 in, 2 out]
                  }
                  frame #2 {
                    n1901 = Wait (ms)(milliseconds to wait=u32 50) -> ()  [unwired: 1 out]
                  }
                  frame #3 {
                    n1902 = case shown="False" w3694 {
                      tunnel: w3695 -> [w3701 w3705]
                      tunnel: [w3702 w3705] -> w3696
                      tunnel: [w3703 w3704] -> w3697
                      tunnel: w3698 -> [w3700 w3704]
                      frame #0 {
                        n1903 = call "mDrive Send Command.vi"("error in (no error)"=w3700, "Command"=T10."Stop", "VISA resource name"=w3701) -> ("error out"=w3703:errorcluster, "VISA resource name out"=w3702:refnum<visa-resource-name>)  [unwired: 4 in, 1 out]
                      }
                      frame #1 {
                      }
                    }
                  }
                  frame #4 {
                    n1904 = property on="R Backlash corr" class="Bool (strict)"() -> ("Value"=w3706:bool)  [unwired: 2 in, 2 out]
                    n1905 = Implies(1:w3712, 2:w3706) -> (0:w3711:bool)
                    n1906 = case shown="False" w3711 {
                      tunnel: w3710 -> [w3720 w3777]
                      tunnel: w3709 -> [w3719 w3778]
                      tunnel: [w3714 w3777] -> w3708
                      tunnel: [w3718 w3778] -> w3707
                      frame #0 {
                        # "Backlash"
                        n1907 = flat-sequence {
                          tunnel: [w3733] -> w3732
                          tunnel: [w3737] -> w3731
                          tunnel: [w3736] -> w3730
                          tunnel: w3720 -> [w3735]
                          tunnel: w3719 -> [w3734]
                          tunnel: w3732 -> [w3745]
                          tunnel: [w3745] -> w3729
                          tunnel: w3731 -> [w3744]
                          tunnel: w3730 -> [w3743]
                          tunnel: [w3742] -> w3728
                          tunnel: [w3741] -> w3727
                          tunnel: [w3740] -> w3717
                          tunnel: w3729 -> [w3759]
                          tunnel: w3728 -> [w3750]
                          tunnel: w3727 -> [w3758]
                          tunnel: [w3750] -> w3726
                          tunnel: [w3758] -> w3725
                          tunnel: [w3749] -> w3722
                          tunnel: [w3757] -> w3721
                          tunnel: w3717 -> [w3757]
                          tunnel: w3726 -> [w3762]
                          tunnel: w3725 -> [w3763]
                          tunnel: [w3761] -> w3724
                          tunnel: [w3769] -> w3723
                          tunnel: w3722 -> [w3769]
                          tunnel: w3721 -> [w3765]
                          tunnel: [w3764] -> w3715
                          tunnel: w3724 -> [w3772]
                          tunnel: w3723 -> [w3771]
                          tunnel: [w3773] -> w3716
                          tunnel: w3715 -> [w3773]
                          tunnel: [w3772] -> w3713
                          tunnel: [w3776] -> w3718
                          tunnel: w3716 -> [w3776]
                          tunnel: [w3775] -> w3714
                          tunnel: w3713 -> [w3775]
                          frame #0 {
                            n1908 = property on="R Backlash steps/sec" class="DigNum (strict)"() -> ("Value"=w3733:i32)  [unwired: 2 in, 2 out]
                            n1909 = Number To Decimal String(number=w3733) -> (decimal integer string=w3738:string)  [unwired: 1 in]
                            n1910 = call "mDrive Send Command.vi"("error in (no error)"=w3735, "Extra"=w3738, "Command"=T10."Max Velocity", "VISA resource name"=w3734) -> ("error out"=w3736:errorcluster, "VISA resource name out"=w3737:refnum<visa-resource-name>)  [unwired: 3 in, 1 out]
                          }
                          frame #1 {
                            n1911 = property on="R Backlash steps/sec" class="DigNum (strict)"() -> ("Value"=w3740:i32)  [unwired: 2 in, 2 out]
                            n1912 = Number To Decimal String(number=w3740) -> (decimal integer string=w3746:string)  [unwired: 1 in]
                            n1913 = call "mDrive Send Command.vi"("error in (no error)"=w3743, "Extra"=w3746, "Command"=T10."Move to Relative Position", "VISA resource name"=w3744) -> ("error out"=w3742:errorcluster, "VISA resource name out"=w3741:refnum<visa-resource-name>)  [unwired: 3 in, 1 out]
                          }
                          frame #2 {
                            n1914 = To Double Precision Float(number=w3757) -> (double precision float=w3755:dbl)
                            n1915 = To Double Precision Float(number=w3759) -> (double precision float=w3760:dbl)
                            n1916 = Absolute Value(x=w3755) -> (abs(x)=w3756:dbl)
                            n1917 = Divide(x=w3756, y=w3760) -> (x/y=w3753:dbl)
                            n1918 = Multiply(x=1000.0, y=w3753) -> (x*y=w3751:dbl)
                            n1919 = Add(x=w3751, y=300.0) -> (x+y=w3749:dbl)
                            n1920 = To Unsigned Long Integer(number=w3749) -> (unsigned 32bit integer=w3748:u32)
                            n1921 = Wait (ms)(milliseconds to wait=w3748) -> ()  [unwired: 1 out]
                          }
                          frame #3 {
                            n1922 = Negate(x=w3765) -> (-x=w3766:i32)
                            n1923 = Number To Decimal String(number=w3766) -> (decimal integer string=w3767:string)  [unwired: 1 in]
                            n1924 = call "mDrive Send Command.vi"("error in (no error)"=w3762, "Extra"=w3767, "Command"=T10."Move to Relative Position", "VISA resource name"=w3763) -> ("error out"=w3761:errorcluster, "VISA resource name out"=w3764:refnum<visa-resource-name>)  [unwired: 3 in, 1 out]
                          }
                          frame #4 {
                            n1925 = To Unsigned Long Integer(number=w3771) -> (unsigned 32bit integer=w3770:u32)
                            n1926 = Wait (ms)(milliseconds to wait=w3770) -> ()  [unwired: 1 out]
                          }
                          frame #5 {
                            n1927 = property on="R Backlash corr" class="Bool (strict)"("Val(Sgnl)"=FALSE ("Value (Signaling)")) -> ()  [unwired: 2 in, 2 out]
                          }
                        }
                      }
                      frame #1 {
                      }
                    }
                  }
                }
                n1928 = property on="Y in Motion" class="Bool (strict)"() -> ("Value"=w3586:bool)  [unwired: 2 in, 2 out]
                n1929 = property on="Z in Motion" class="Bool (strict)"() -> ("Value"=w3574:bool)  [unwired: 2 in, 2 out]
                n1930 = property on="X  in Motion" class="Bool (strict)"() -> ("Value"=w3585:bool)  [unwired: 2 in, 2 out]
                n1931 = property on="R in Motion" class="Bool (strict)"() -> ("Value"=w3573:bool)  [unwired: 2 in, 2 out]
                n1932 = Compound Arithmetic op=OR(w3585, w3586, w3574, w3573) -> (w3584:bool)
                n1933 = Not(x=w3584) -> (.not. x?=w3579:bool)
              }
            }
            frame #7 {
              n1934 = Wait (ms)(milliseconds to wait=u32 1000) -> ()  [unwired: 1 out]
            }
          }
          n1935 = Increment(x=w2618) -> (x+1=w2619:i32)
          n1936 = property on="#th loop" class="DigNum (strict)"("Val(Sgnl)"=w2619) -> ()  [unwired: 2 in, 2 out]
          n1937 = property on="#th loop" class="DigNum (strict)"() -> ("Value"=w2608:dbl)  [unwired: 2 in, 2 out]
          n1938 = property on="# of loops" class="DigNum (strict)"() -> ("Value"=w2609:dbl)  [unwired: 2 in, 2 out]
          n1939 = Greater Or Equal?(x=w2608, y=w2609) -> (x >= y?=w2607:bool)
        }
        n1940 = flat-sequence {
          tunnel: [w4173] -> _
          tunnel: w2590 -> [w4173]
          tunnel: w2589 -> [_]
          tunnel: [w4172] -> _
          tunnel: w2588 -> [w4172]
          tunnel: w2587 -> [_]
          frame #0 {
            w4176 = T9."Enabled" ("Disabled")
            n1941 = property on="Z Scan Length SP steps" class="DigNum (strict)"("DisabledEnum"=T9."Enabled" ("Disabled")) -> ()  [unwired: 2 in, 2 out]
            n1942 = property on="Z Scan Velocity SP steps/sec" class="DigNum (strict)"("DisabledEnum"=T9."Enabled" ("Disabled")) -> ()  [unwired: 2 in, 2 out]
            n1943 = property on="R Scan Length SP steps" class="DigNum (strict)"("DisabledEnum"=T9."Enabled" ("Disabled")) -> ()  [unwired: 2 in, 2 out]
            n1944 = property on="X Scan Velocity SP steps/sec" class="DigNum (strict)"("DisabledEnum"=T9."Enabled" ("Disabled")) -> ()  [unwired: 2 in, 2 out]
            n1945 = property on="GO" class="Bool"("DisabledEnum"=w4176) -> ()  [unwired: 2 in, 2 out]
            n1946 = property on="Set Scan \nParameters" class="Bool"("DisabledEnum"=w4176) -> ()  [unwired: 2 in, 2 out]
            n1947 = property on="Y Scan Length SP steps" class="DigNum (strict)"("DisabledEnum"=T9."Enabled" ("Disabled")) -> ()  [unwired: 2 in, 2 out]
            n1948 = local write "STATUS"("LEAVING LOOP" ("STATUS")) -> ()
            n1949 = property on="R Scan Velocity SP steps/sec" class="DigNum (strict)"("DisabledEnum"=T9."Enabled" ("Disabled")) -> ()  [unwired: 2 in, 2 out]
            n1950 = property on="X Scan Length SP steps" class="DigNum (strict)"("DisabledEnum"=T9."Enabled" ("Disabled")) -> ()  [unwired: 2 in, 2 out]
            n1951 = property on="Y Scan Selocity SP steps/sec" class="DigNum (strict)"("DisabledEnum"=T9."Enabled" ("Disabled")) -> ()  [unwired: 2 in, 2 out]
            n1952 = property on="Send scan parameter" class="Bool"("DisabledEnum"=w4176) -> ()  [unwired: 2 in, 2 out]
            n1953 = property on="Scan Go" class="Bool (strict)"("DisabledEnum"=T9."Disabled and Grayed Out" ("Disabled")) -> ()  [unwired: 2 in, 2 out]
          }
        }
      }
    }
    n1954 = case shown="False" "Delete Button" {
      tunnel: w296 -> [_ w329]
      frame #0 {
      }
      frame #1 {
        n1955 = local read "Preset positions"() -> (w327:i32)
        n1956 = local read "Presets"() -> (w328:i32[][])
        n1957 = Delete From Array(array=w329, index=w327) -> (array with subset deleted=w325:string[])  [unwired: 1 in, 1 out]
        n1958 = property on="Preset positions" class="Ring (strict)"("Strings []"=w325) -> ()  [unwired: 2 in, 2 out]
        n1959 = Delete From Array(array=w328, index (row)=w327) -> (array with subset deleted=w326:i32[][])  [unwired: 2 in, 1 out]
        n1960 = local write "Presets"(w326) -> ()
      }
    }
    n1961 = case shown="False" "Add Button" {
      tunnel: w296 -> [_ w339]
      frame #0 {
      }
      frame #1 {
        n1962 = property on="X Step PV" class="DigNum (strict)"() -> ("Value"=w333:i32)  [unwired: 2 in, 2 out]
        n1963 = property on="Y Step PV" class="DigNum (strict)"() -> ("Value"=w332:i32)  [unwired: 2 in, 2 out]
        n1964 = property on="Z Step PV" class="DigNum (strict)"() -> ("Value"=w330:i32)  [unwired: 2 in, 2 out]
        n1965 = property on="R Step PV" class="DigNum (strict)"() -> ("Value"=w331:i32)  [unwired: 2 in, 2 out]
        n1966 = Build Array(w333, w332, w330, w331) -> (w336:i32[])
        n1967 = Build Array (concatenate)(w339, "String") -> (w334:string[])
        n1968 = local read "Presets"() -> (w337:i32[][])
        n1969 = property on="Preset positions" class="Ring (strict)"("Strings []"=w334) -> ()  [unwired: 2 in, 2 out]
        n1970 = Build Array (concatenate)(w337, w336) -> (w335:i32[][])
        n1971 = local write "Presets"(w335) -> ()
      }
    }
    n1972 = case shown="False" "Set Button" {
      tunnel: "Preset positions" -> [_ w346]
      frame #0 {
      }
      frame #1 {
        n1973 = local read "Presets"() -> (w347:i32[][])
        n1974 = Index Array(array=w347, index (row)=w346) -> (element=w345:i32[])  [unwired: 1 in]
        n1975 = Array To Cluster(array=w345) -> (cluster=w344:T11)
        n1976 = Unbundle(w344) -> ("Presets[0]"=w343:i32, "Presets[1]"=w342:i32, "Presets[2]"=w341:i32, "Presets[3]"=w340:i32)  [unwired: 5 out]
        n1977 = property on="X Step SP" class="DigNum (strict)"("Val(Sgnl)"=w343) -> ()  [unwired: 2 in, 2 out]
        n1978 = property on="Y Step SP" class="DigNum (strict)"("Val(Sgnl)"=w342) -> ()  [unwired: 2 in, 2 out]
        n1979 = property on="Z Step SP" class="DigNum (strict)"("Val(Sgnl)"=w341) -> ()  [unwired: 2 in, 2 out]
        n1980 = property on="R Step SP" class="DigNum (strict)"("Val(Sgnl)"=w340) -> ()  [unwired: 2 in, 2 out]
      }
    }
    n1981 = property on="STATUS" class="Str"() -> ("Value"=w289:string)  [unwired: 2 in, 2 out]
    n1982 = Equal?(x=w289, y="SCANNING MODE" ("STATUS")) -> (x = y?=w287:bool)
    "Scanning" <- w287
    n1983 = case shown="True" "Laser Shutter" {
      tunnel: "SHUTTER SYNC" -> [w323 _]
      tunnel: w287 -> [w322 _]
      frame #0 {
        # "SHUTTER SLAVE MODE"
        n1984 = And(x=w323, y=w322) -> (x .and. y?=w324:bool)
        n1985 = case shown="False" w324 {
          frame #0 {
            # "CLOE SHUTTER"
          }
          frame #1 {
            # "OPEN SHUTTER"
          }
        }
      }
      frame #1 {
        # "FORCE TO OPEN SHUTTER"
      }
    }
    n1986 = case shown="False" "Stop" {
      selector: "Stop" -> [w356 w398]
      tunnel: [w356 w395] -> w303
      tunnel: w286 -> [w355 w364]
      tunnel: w283 -> [w354 w363]
      tunnel: [w355 w371] -> w312
      tunnel: [w353 w377] -> w311
      tunnel: [w352 w374] -> w310
      tunnel: [w351 w383] -> w309
      tunnel: [w349 w366] -> w308
      tunnel: [w348 w365] -> w307
      tunnel: [w350 w380] -> w306
      tunnel: [w354 w368] -> w305
      tunnel: w302 -> [_ w390]
      tunnel: w301 -> [_ w367]
      tunnel: w285 -> [w353 w362]
      tunnel: w284 -> [w352 w361]
      tunnel: w282 -> [w351 w360]
      tunnel: w281 -> [w350 w359]
      tunnel: w280 -> [w348 w358]
      tunnel: w279 -> [w349 w357]
      frame #0 {
      }
      frame #1 {
        n1987 = flat-sequence {
          tunnel: w398 -> [w464]
          tunnel: [w464] -> w397
          tunnel: [w463] -> w393
          tunnel: [w462] -> w391
          tunnel: w390 -> [w462]
          tunnel: [w417] -> w388
          tunnel: [w416] -> w386
          tunnel: [w426] -> w384
          tunnel: [w425] -> w381
          tunnel: [w436] -> w378
          tunnel: [w434] -> w375
          tunnel: [w445] -> w372
          tunnel: [w443] -> w369
          tunnel: w367 -> [w453]
          tunnel: w364 -> [w406]
          tunnel: w363 -> [w405]
          tunnel: w362 -> [w404]
          tunnel: w361 -> [w403]
          tunnel: w360 -> [w402]
          tunnel: w359 -> [w401]
          tunnel: w358 -> [w400]
          tunnel: w357 -> [w399]
          tunnel: w397 -> [w476]
          tunnel: [w476] -> w396
          tunnel: [w465] -> w394
          tunnel: w393 -> [w475]
          tunnel: [w474] -> w392
          tunnel: w391 -> [w474]
          tunnel: [w473] -> w389
          tunnel: w388 -> [w473]
          tunnel: [w472] -> w387
          tunnel: w386 -> [w472]
          tunnel: [w471] -> w385
          tunnel: w384 -> [w471]
          tunnel: [w470] -> w382
          tunnel: w381 -> [w470]
          tunnel: [w469] -> w379
          tunnel: w378 -> [w469]
          tunnel: [w468] -> w376
          tunnel: w375 -> [w468]
          tunnel: [w467] -> w373
          tunnel: w372 -> [w467]
          tunnel: [w466] -> w370
          tunnel: w369 -> [w466]
          tunnel: w396 -> [w488]
          tunnel: [w488] -> w395
          tunnel: w394 -> [w479]
          tunnel: w392 -> [w487]
          tunnel: w389 -> [w478]
          tunnel: [w478] -> _
          tunnel: w387 -> [w486]
          tunnel: [w486] -> w365
          tunnel: w385 -> [w485]
          tunnel: [w485] -> w383
          tunnel: [w484] -> w380
          tunnel: w382 -> [w484]
          tunnel: [w483] -> w377
          tunnel: w379 -> [w483]
          tunnel: [w482] -> w374
          tunnel: w376 -> [w482]
          tunnel: [w481] -> w371
          tunnel: w373 -> [w481]
          tunnel: [w480] -> w368
          tunnel: w370 -> [w480]
          tunnel: [w478] -> w366
          frame #0 {
            # "R"
            # "Y"
            # "Z"
            # "X"
            n1988 = local read "Presets"() -> (w452:i32[][])
            n1989 = property on="Preset positions" class="Ring (strict)"() -> ("Strings []"=w451:string[])  [unwired: 2 in, 2 out]
            n1990 = property on="R Ready" class="Bool (strict)"("Val(Sgnl)"=FALSE ("Value (Signaling)")) -> ()  [unwired: 2 in, 2 out]
            n1991 = property on="R in Range" class="Bool (strict)"("Val(Sgnl)"=FALSE ("Value (Signaling)")) -> ()  [unwired: 2 in, 2 out]
            n1992 = property on="Z in Range" class="Bool (strict)"("Val(Sgnl)"=FALSE ("Value (Signaling)")) -> ()  [unwired: 2 in, 2 out]
            n1993 = property on="Z Ready" class="Bool (strict)"("Val(Sgnl)"=FALSE ("Value (Signaling)")) -> ()  [unwired: 2 in, 2 out]
            n1994 = property on="Y in Range" class="Bool (strict)"("Val(Sgnl)"=FALSE ("Value (Signaling)")) -> ()  [unwired: 2 in, 2 out]
            n1995 = property on="X  in Range" class="Bool (strict)"("Val(Sgnl)"=FALSE ("Value (Signaling)")) -> ()  [unwired: 2 in, 2 out]
            n1996 = property on="Y Ready" class="Bool (strict)"("Val(Sgnl)"=FALSE ("Value (Signaling)")) -> ()  [unwired: 2 in, 2 out]
            n1997 = property on="X Ready" class="Bool (strict)"("Val(Sgnl)"=FALSE ("Value (Signaling)")) -> ()  [unwired: 2 in, 2 out]
            n1998 = Number To Fractional String(number=w452) -> (F-format string=w454:string[][])  [unwired: 3 in]
            n1999 = call "mDrive Send Command.vi"("error in (no error)"=w405, "Command"=T10."Stop", "VISA resource name"=w406) -> ("error out"=w444:errorcluster, "VISA resource name out"=w446:refnum<visa-resource-name>)  [unwired: 4 in, 1 out]
            n2000 = call "mDrive Send Command.vi"("error in (no error)"=w403, "Command"=T10."Stop", "VISA resource name"=w404) -> ("error out"=w435:errorcluster, "VISA resource name out"=w437:refnum<visa-resource-name>)  [unwired: 4 in, 1 out]
            n2001 = Transpose 2D Array(2D array=w454) -> (transposed array=w455:string[][])
            n2002 = call "mDrive Send Command.vi"("error in (no error)"=w401, "Command"=T10."Stop", "VISA resource name"=w402) -> ("error out"=w427:errorcluster, "VISA resource name out"=w428:refnum<visa-resource-name>)  [unwired: 4 in, 1 out]
            n2003 = call "mDrive Send Command.vi"("error in (no error)"=w400, "Command"=T10."Stop", "VISA resource name"=w399) -> ("error out"=w418:errorcluster, "VISA resource name out"=w419:refnum<visa-resource-name>)  [unwired: 4 in, 1 out]
            n2004 = Build Array (concatenate)(w451, w455) -> (w456:string[][])
            n2005 = Transpose 2D Array(2D array=w456) -> (transposed array=w457:string[][])
            n2006 = call "mDrive Send Command.vi"("error in (no error)"=w444, "Extra"="P", "Command"=T10."Print Parameter", "VISA resource name"=w446) -> ("error out"=w443:errorcluster, "read buffer"=w450:string, "VISA resource name out"=w445:refnum<visa-resource-name>)  [unwired: 3 in]
            n2007 = call "mDrive Send Command.vi"("error in (no error)"=w435, "Extra"="P", "Command"=T10."Print Parameter", "VISA resource name"=w437) -> ("error out"=w434:errorcluster, "read buffer"=w441:string, "VISA resource name out"=w436:refnum<visa-resource-name>)  [unwired: 3 in]
            n2008 = call "mDrive Send Command.vi"("error in (no error)"=w427, "Extra"="P", "Command"=T10."Print Parameter", "VISA resource name"=w428) -> ("error out"=w425:errorcluster, "read buffer"=w432:string, "VISA resource name out"=w426:refnum<visa-resource-name>)  [unwired: 3 in]
            n2009 = call "mDrive Send Command.vi"("error in (no error)"=w418, "Extra"="P", "Command"=T10."Print Parameter", "VISA resource name"=w419) -> ("error out"=w416:errorcluster, "read buffer"=w423:string, "VISA resource name out"=w417:refnum<visa-resource-name>)  [unwired: 3 in]
            n2010 = call-poly <vilib>:"Write To Spreadsheet File.vi"("2D data"=w457, "file path (dialog if empty)"=w453) -> ()  [unwired: 6 in, 1 out]
            n2011 = Decimal String To Number(string=w450, offset=0) -> (number=w442:i32)  [unwired: 1 in, 1 out]
            n2012 = Decimal String To Number(string=w441, offset=0) -> (number=w433:i32)  [unwired: 1 in, 1 out]
            n2013 = Decimal String To Number(string=w432, offset=0) -> (number=w424:i32)  [unwired: 1 in, 1 out]
            n2014 = Decimal String To Number(string=w423, offset=0) -> (number=w415:i32)  [unwired: 1 in, 1 out]
            n2015 = Build Array(w442, w424, w433, w415) -> (w463:i32[])
          }
          frame #1 {
            n2016 = To Double Precision Float(number=w475) -> (double precision float=w465:dbl[])
            n2017 = Wait (ms)(milliseconds to wait=u32 20) -> ()  [unwired: 1 out]
          }
          frame #2 {
            n2018 = call-poly <vilib>:"Write To Spreadsheet File.vi"("1D data"=w479, "file path (dialog if empty)"=w487) -> ()  [unwired: 6 in, 1 out]
          }
        }
      }
    }
  }
  n2019 = flat-sequence {
    tunnel: w58 -> [w4207]
    tunnel: w57 -> [w4204]
    frame #0 {
      n2020 = call "mDrive Send Command.vi"("error in (no error)"=w4204, "Command"=T10."Stop", "VISA resource name"=w4207) -> ("error out"=w4205:errorcluster, "VISA resource name out"=w4206:refnum<visa-resource-name>)  [unwired: 4 in, 1 out]
      n2021 = VISA Close(VISA resource name=w4206, error in (no error)=w4205) -> ()  [unwired: 1 out]
    }
  }
  n2022 = flat-sequence {
    tunnel: w52 -> [w4212]
    tunnel: w51 -> [w4209]
    frame #0 {
      n2023 = call "mDrive Send Command.vi"("error in (no error)"=w4209, "Command"=T10."Stop", "VISA resource name"=w4212) -> ("error out"=w4210:errorcluster, "VISA resource name out"=w4211:refnum<visa-resource-name>)  [unwired: 4 in, 1 out]
      n2024 = VISA Close(VISA resource name=w4211, error in (no error)=w4210) -> ()  [unwired: 1 out]
    }
  }
  n2025 = flat-sequence {
    tunnel: w50 -> [w4217]
    tunnel: w49 -> [w4214]
    frame #0 {
      n2026 = call "mDrive Send Command.vi"("error in (no error)"=w4214, "Command"=T10."Stop", "VISA resource name"=w4217) -> ("error out"=w4215:errorcluster, "VISA resource name out"=w4216:refnum<visa-resource-name>)  [unwired: 4 in, 1 out]
      n2027 = VISA Close(VISA resource name=w4216, error in (no error)=w4215) -> ()  [unwired: 1 out]
    }
  }
  n2028 = flat-sequence {
    tunnel: w48 -> [w4222]
    tunnel: w47 -> [w4219]
    frame #0 {
      n2029 = call "mDrive Send Command.vi"("error in (no error)"=w4219, "Command"=T10."Stop", "VISA resource name"=w4222) -> ("error out"=w4220:errorcluster, "VISA resource name out"=w4221:refnum<visa-resource-name>)  [unwired: 4 in, 1 out]
      n2030 = VISA Close(VISA resource name=w4221, error in (no error)=w4220) -> ()  [unwired: 1 out]
    }
  }
  "YCONSTArray" <- w46
  "XCONSTArray" <- w45
  "RCONSTArray" <- w44
  "ZCONSTArray" <- w43
  "RUNHOLDArray" <- w42
